vi "SPARC4_AC.vi"() -> ()   [LabVIEW 2018]
uses:
  SPARC4_AC/SPARC4_AC.lvclass
  Channel Manager/Channel Manager.lvclass/Channel Manager.ctl
  Sync Box/Sync Box.lvclass
  Readout delay charact/Readout Delay Charact/Readout Charact.lvclass
  Channel Manager/Channel Manager.lvclass
  RxTx/RxTx.lvclass
  Interface/Interface.lvclass
  State Machine/State Machine.lvclass
  Setup File/Setup File.lvclass
panel:
  out "String":string="#img      1st Time       2nd Time      3th Time      4th Time      5th Time\n------------------------------------------------------------------------\n"
  in  "Camera Setup":T1={"Image Name"="Image", "Image Path"="C:\\Users\\Cliente\\Desktop\\SPARC4_AC\\Imagens\\", "# Images"=0, "Exposure Time"=0.0, "Pre-amp gain"=0, "Readout Rate"=0, "Vertical Shift Speed"=3, "Acquisition Mode"=1, "Read Mode"=4, "EM Mode"=0, "EM Gain"=2, "Shutter Mode"=2, "Shutter TTL"=0, "Time to open shutter"=50, "Time to close shutter"=50, "Vertical Binning"=1, "Horizontal Binning"=1, "Initial Line"=1, "Initial Cloumn"=1, "Final Line"=1024, "Final Column"=1024, "Cooler ON/OFF"=0, "Set temperature"=20, "Number of exp"=0, "Exposições realizadas"=0, "Kinetic Serie Length"=0, "Number of Accumulations"=0, "Kinetic Cycle Time"=0, "Frame Transfer"=FALSE, "Vertical Clock Amplitude"=0, "Trigger"=0} {"Trigger" items=["Internal", "External", "N/A", "N/A", "N/A", "N/A", "External Start"]; "Vertical Clock Amplitude" items=["Normal", "+1", "+2", "+3", "+4"]; "Set temperature" min=0 max=0; "Cooler ON/OFF" items=["Cooler OFF", "Cooler ON"]; "Shutter TTL" items=["TTL Low", "TTl High"]; "Shutter Mode" items=["Fully Auto", "OPEN", "CLOSED"]; "EM Mode" items=["Electron Multiplying", "Conventional"]; "Read Mode" items=["Full Vertical Binning", "Multi-Track", "Random-track", "Single-Track", "Image"]; "Acquisition Mode" items=["N/A", "Single", "Accumulate", "Kinetic", "Fast Kinetic"]; "Vertical Shift Speed" items=["0.6", "1.13", "2.2", "4.33"]; "Readout Rate" items=["1 MHz", "10 MHz", "20 MHz", "30 MHz"]; "Pre-amp gain" items=["Gain 1", "Gain 2"]}
  in  "Setup":T2
  in  "Initial Line 6":u16=1 min=1
  in  "Interface de controle":enum32{"Acquisition", "Setup"}(tab)
  in  "Pausar 5":bool
  in  "Stop Acq 5":bool
  in  "Adquirir 5":bool
  in  "Abort 5":bool
  in  "Pausar 2":bool
  in  "Stop Acq 2":bool
  in  "Adquirir 2":bool
  in  "Abort 2":bool
  in  "Pausar 4":bool
  in  "Stop Acq 4":bool
  in  "Adquirir 4":bool
  in  "Abort 4":bool
  in  "Pausar":bool
  in  "Stop Acq":bool
  in  "Adquirir":bool
  in  "Abort":bool
  in  "Sync Mode":bool
  out "Exposing":bool
  in  "Image Name":string="CH1"
  out "Temperature":i16
  in  "Exposure Time":dbl=1e-05 min=1e-05
  in  "# Ciclos":u32=1 min=1
  out "% Acquired":dbl format="%#.2g"
  in  "Night Directory":string="C:\\Users\\observer\\Desktop\\SPARC4 Acquisition Control\\Imagens"
  in  "COMP":bool
  in  "FLAT":bool
  in  "BIAS":bool
  in  "SCIENCE":bool
  in  "Load Setup":bool
  out "Setup File Path:":string
  in  "Read mode":enum32{"No Selection", "1", "2", "3"}(radio)=enum."1"
  in  "Sync Mode: 2":T3(radio)
  in  "Image Name 4":string="CH1"
  out "Initialization 4":bool
  in  "Exposure Time 6":dbl
  in  "# Images 4":u32=1 min=1
  out "Temperature 4":i16
  out "Exposing 4":bool
  out "% Acquired 4":dbl format="%#.2g"
  out "Exposições realizadas 4":u8(slide) max=1 scale=0.0..1.0
  in  "Image Name 3":string="CH1"
  out "Initialization 3":bool
  in  "Exposure Time 5":dbl
  in  "# Images 3":u32=1 min=1
  out "Temperature 3":i16
  out "Exposing 3":bool
  out "% Acquired 3":dbl format="%#.2g"
  out "Exposições realizadas 3":u8(slide) max=1 scale=0.0..1.0
  in  "Pausar 3":bool
  in  "Stop Acq 3":bool
  in  "Abort 3":bool
  in  "Adquirir 3":bool
  in  "Image Name 2":string="CH2"
  out "Initialization 2":bool
  in  "Exposure Time 3":u32
  in  "# Images 2":u32=1 min=1
  out "Temperature 2":i16
  out "Exposing 2":bool
  out "% Acquired 2":dbl format="%#.2g"
  out "Exposições realizadas 2":u8(slide) max=1 scale=0.0..1.0
  out "Initialization":bool
  out "Exposições realizadas":u8(slide) max=1 scale=0.0..1.0
  in  "Stop Button":bool
  in  "Tab Control 2":T4(tab)
  in  "Cooler ON/OFF":u16(ring) items=["Cooler OFF", "Cooler ON"]
  in  "Set temperature":i8=20 min=-80 max=20
  out "Temperature ºC":dbl(slide)=20.0 min=-120.0 max=20.0 scale=-80.0..20.0
  in  "Exposure Time 2":dbl=1e-05 min=1e-05
  in  "Readout Rate":u8(ring) items=["30 MHz", "20 MHz", "10 MHz", "  1 MHz"]
  in  "Pre-amp gain":u8(ring) items=["Gain 1", "Gain 2"]
  in  "Kinetic Series Length":u8=1 min=1 max=80
  in  "Sub Image":T5(radio)=enum."1024 x 1024"
  in  "Initial Line":u16=1 min=1 max=1024
  in  "Final Line":u16=1024 min=1 max=1024
  in  "Final Column":u16=1024 min=1 max=1024
  in  "Initial Cloumn":u16=1 min=1 max=1024
  in  "Binning 5":u8=1 min=1 max=2
  in  "EM Gain":u16=2 min=2 max=300
  in  "EM Mode":u8(ring) items=["Electron Multiplying", "Conventional"]
  in  "Save CH1":bool
  in  "Save CH2":bool
  in  "Cooler ON/OFF 2":u16(ring) items=["Cooler OFF", "Cooler ON"]
  in  "Set temperature 2":i8=20 min=-120 max=20
  out "Temperature ºC 2":dbl(slide)=20.0 min=-120.0 max=20.0 scale=-80.0..20.0
  in  "Exposure Time 4":u32
  in  "Readout Rate 2":u8(ring) items=["1 MHz", "10 MHz", "20 MHz", "30 MHz"]
  in  "Pre-amp gain 2":u8(ring) items=["Gain 1", "Gain 2"]
  in  "EM Gain 2":u16=2
  in  "EM Mode 2":u8(ring) items=["Electron Multiplying", "Conventional"]
  in  "Sub Image 2":T5(radio)=enum."1024 x 1024"
  in  "Final Line 2":u16=1024
  in  "Final Column 2":u16=1024
  in  "Initial Cloumn 2":u16=1
  in  "Initial Line 2":u16=1
  in  "Binning 6":u16=1
  in  "Save CH3":bool
  in  "Cooler ON/OFF 3":u16(ring) items=["Cooler OFF", "Cooler ON"]
  in  "Set temperature 3":i8=20 min=-120 max=20
  out "Temperature ºC 3":dbl(slide)=20.0 min=-120.0 max=20.0 scale=-80.0..20.0
  in  "Exposure Time 7":dbl
  in  "Readout Rate 3":u8(ring) items=["1 MHz", "10 MHz", "20 MHz", "30 MHz"]
  in  "Pre-amp gain 3":u8(ring) items=["Gain 1", "Gain 2"]
  in  "EM Gain 3":u16=2
  in  "EM Mode 3":u8(ring) items=["Electron Multiplying", "Conventional"]
  in  "Sub Image 3":T5(radio)=enum."1024 x 1024"
  in  "Final Line 3":u16=1024
  in  "Final Column 3":u16=1024
  in  "Initial Cloumn 3":u16=1
  in  "Initial Line 3":u16=1
  in  "Binning 7":u16=1
  in  "Save CH4":bool
  in  "Cooler ON/OFF 4":u16(ring) items=["Cooler OFF", "Cooler ON"]
  in  "Set temperature 4":i8=20 min=-120 max=20
  out "Temperature ºC 4":dbl(slide)=20.0 min=-120.0 max=20.0 scale=-80.0..20.0
  in  "Exposure Time 8":dbl
  in  "Readout Rate 4":u8(ring) items=["1 MHz", "10 MHz", "20 MHz", "30 MHz"]
  in  "Pre-amp gain 4":u8(ring) items=["Gain 1", "Gain 2"]
  in  "EM Gain 4":u16=2
  in  "EM Mode 4":u8(ring) items=["Electron Multiplying", "Conventional"]
  in  "Sub Image 4":T5(radio)=enum."1024 x 1024"
  in  "Final Line 4":u16=1024
  in  "Final Column 4":u16=1024
  in  "Initial Cloumn 4":u16=1
  in  "Initial Line 4":u16=1
  in  "Binning 8":u16=1
  in  "SPARC4_AC.lvclass":refnum<class "SPARC4_AC.lvclass">
  # "#img      1st Time       2nd Time      3th Time      4th Time      5th Time"
  # "Sparc4:\n Acquisition Controller"
  # "Channel 1"
  # "Channel 2"
  # "Channel 3"
  # "Channel 4"
  # "Timings"
  # "Temperature"
  # "HSS & Preamp"
  # "EM Mode"
  # "Sub Image & Binning"
  # "Timings"
  # "Temperature"
  # "EM Mode"
  # "HSS & Preamp"
  # "Sub Image & Binning"
  # "Timings"
  # "Temperature"
  # "HSS & Preamp"
  # "EM Mode"
  # "Sub Image & Binning"
  # "Temperature"
  # "Timings"
  # "EM Mode"
  # "Horizontal pixel shift"
  # "Sub Image & Binning"
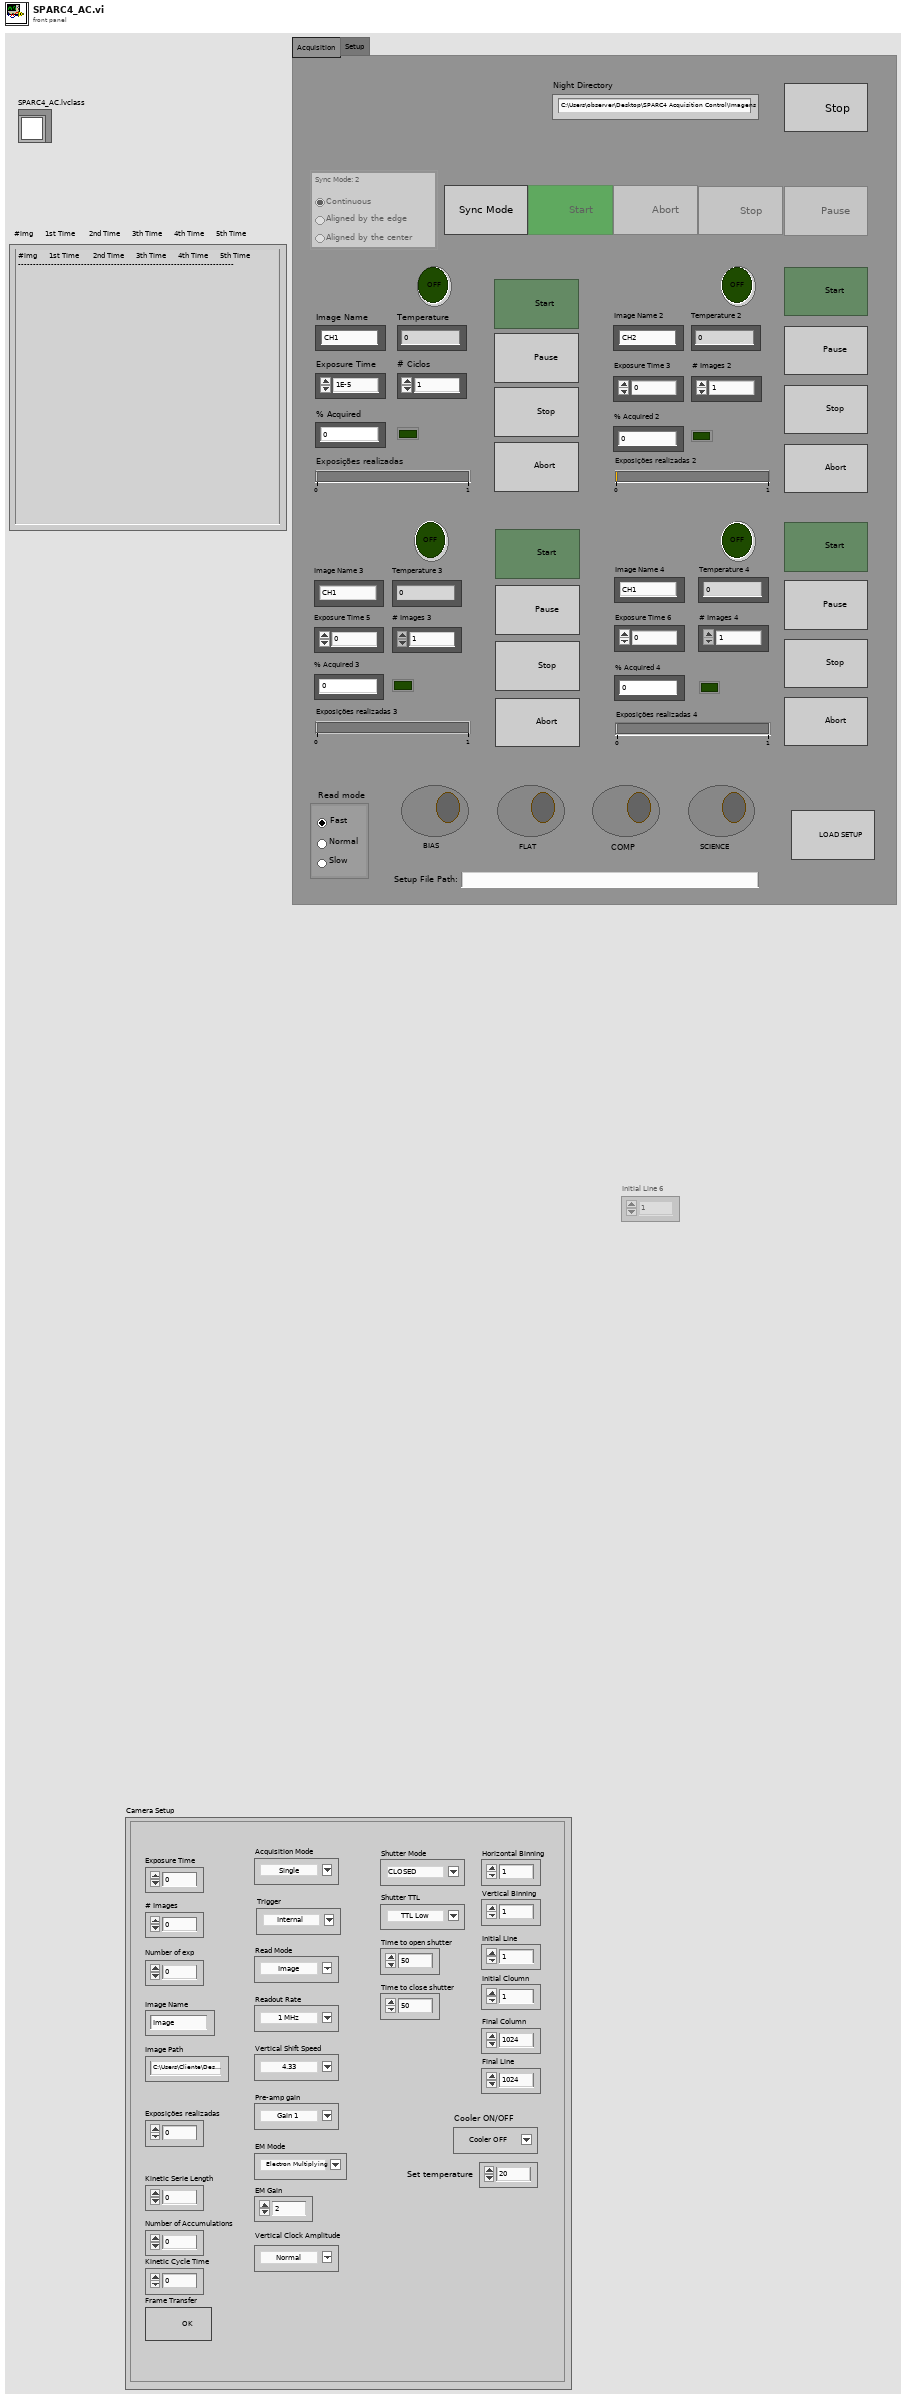
[diagram p1: front panel]
types:
  T1 = cluster{"Image Name":string, "Image Path":string, "# Images":u32, "Exposure Time":dbl, "Pre-amp gain":u8, "Readout Rate":u8, "Vertical Shift Speed":u8, "Acquisition Mode":u8, "Read Mode":u8, "EM Mode":u8, "EM Gain":u16, "Shutter Mode":u8, "Shutter TTL":u8, "Time to open shutter":u16, "Time to close shutter":u16, "Vertical Binning":u16, "Horizontal Binning":u16, "Initial Line":u16, "Initial Cloumn":u16, "Final Line":u16, "Final Column":u16, "Cooler ON/OFF":u16, "Set temperature":i8, "Number of exp":u32, "Exposições realizadas":u16, "Kinetic Serie Length":u32, "Number of Accumulations":u32, "Kinetic Cycle Time":u32, "Frame Transfer":bool, "Vertical Clock Amplitude":u8, "Trigger":u8}
  T2 = cluster{"Read Mode":string, "Acquisition Mode":string, "Trigger":string, "Exposure Time":string, "VShift Speed":string, "Readout rate":string, "Pre amp":string, "Shutter Mode":string, "Shutter TTL":string, "Time to open shutter":string, "Time to close shutter":string, "Cooler":string, "Temperature":string, "Initial Line":string, "Initial Column":string, "Final Line":string, "Final Column":string, "Horizontal binning":string, "Vertical binning":string, "Sub image":string, "CHANNEL":string, "EM Mode":string, "EM Gain":string}
  T3 = enum32{"Radio Selection 1", "Radio Selection 2", "Radio Selection 3", "Radio Selection 4"}
  T4 = enum32{"Channel 1", "Channel 2", "Channel 3", "Channel 4"}
  T5 = enum32{"256 x 256", "512 x 512", "1024 x 1024", "Custom"}
  T6 = cluster{"% Acquired":dbl, "Acquiring":bool, "Current Temperature":dbl, "Temperatue Status":string, "Min Temp":dbl, "Max Temp":dbl, "Exposições realizadas":u32, "Final Column":u16, "Final Line":u16}
  T7 = enum8{"Enabled", "Disabled", "Disabled and Grayed Out"}
  T8 = enum32{"256 x 256", "512 x 512", "1024 x 1024", "Custom", "128 x 128", "64 x 64"}
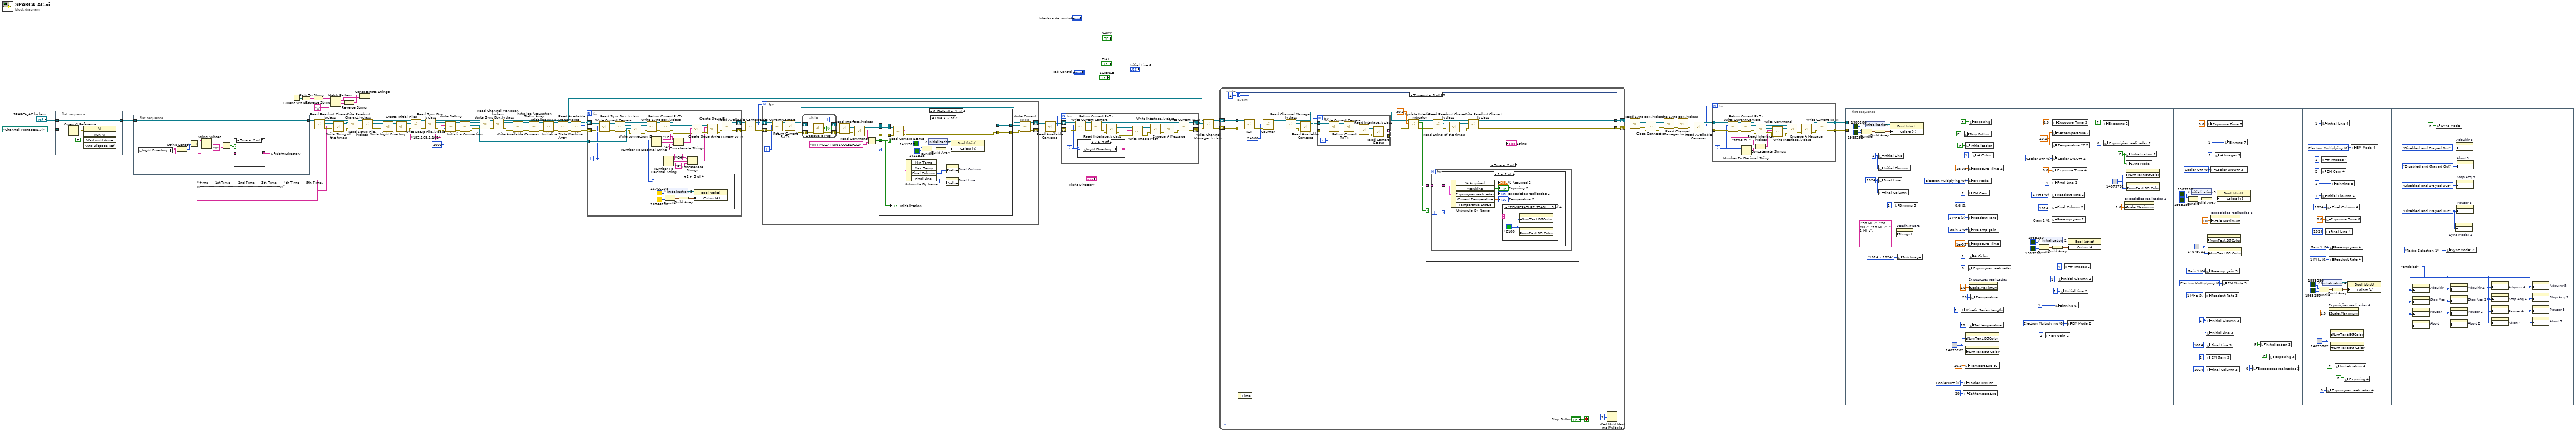
[diagram p0: block diagram]
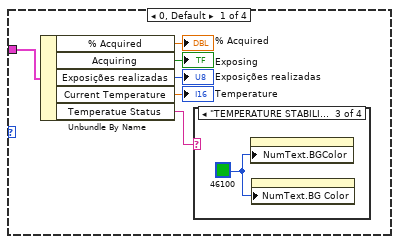
[diagram p3: hidden frame]
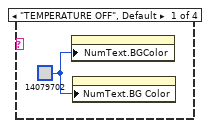
[diagram p4: hidden frame]
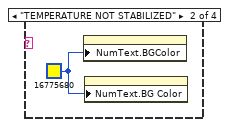
[diagram p5: hidden frame]
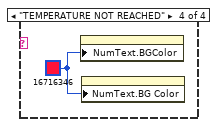
[diagram p6: hidden frame]
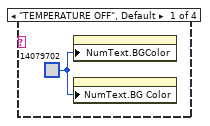
[diagram p7: hidden frame]
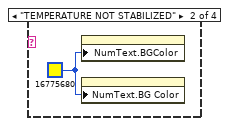
[diagram p8: hidden frame]
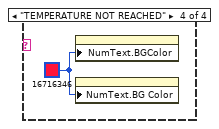
[diagram p9: hidden frame]
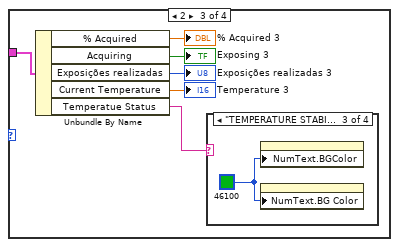
[diagram p10: hidden frame]
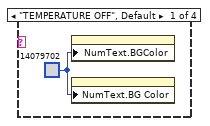
[diagram p11: hidden frame]
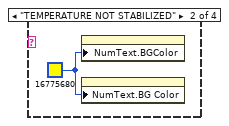
[diagram p12: hidden frame]
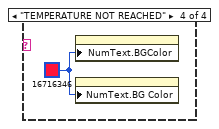
[diagram p13: hidden frame]
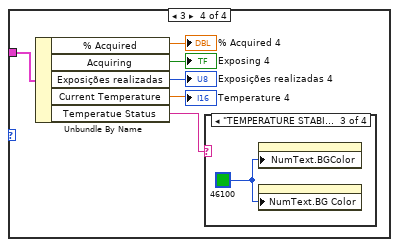
[diagram p14: hidden frame]
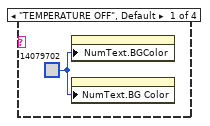
[diagram p15: hidden frame]
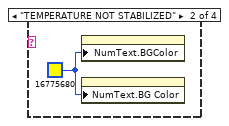
[diagram p16: hidden frame]
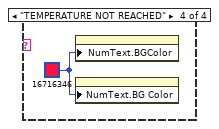
[diagram p17: hidden frame]
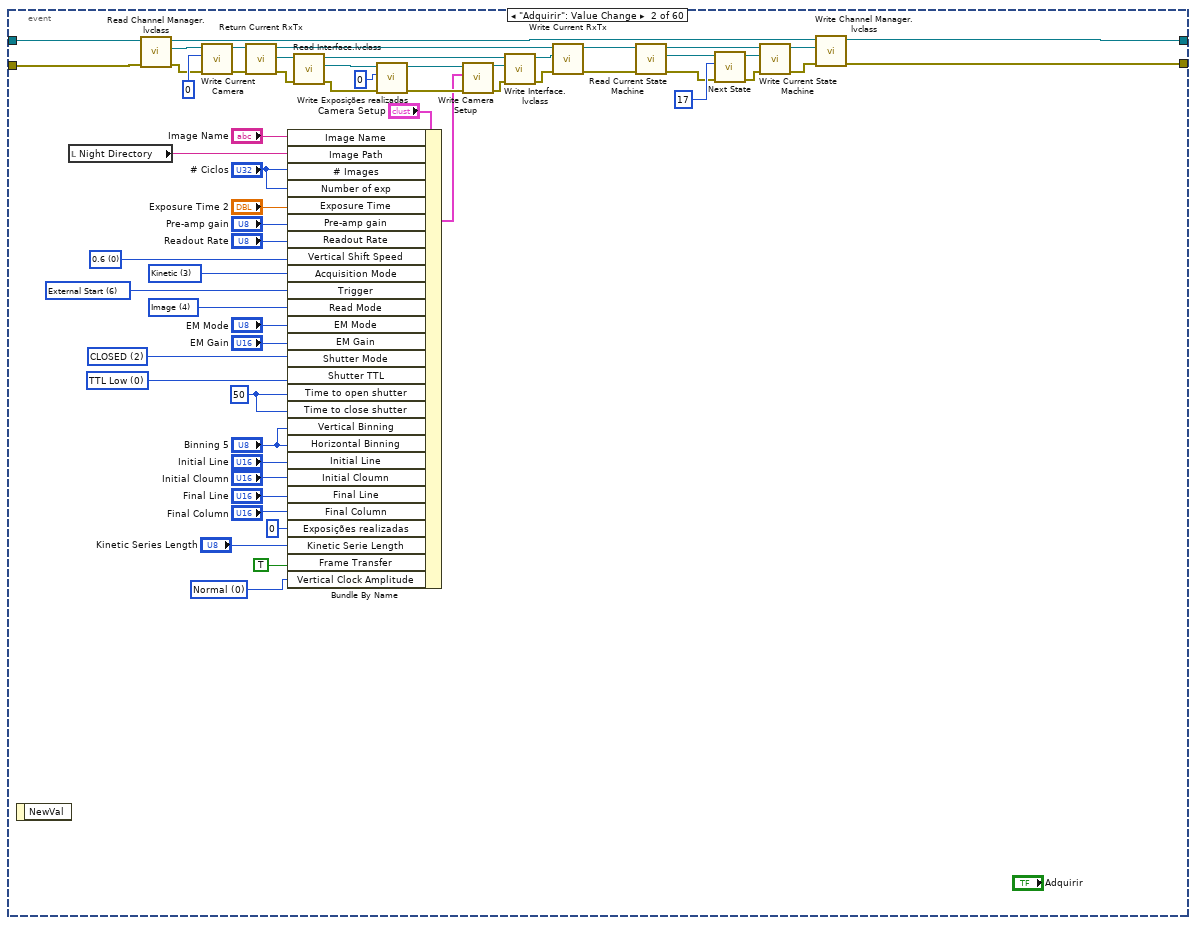
[diagram p18: hidden frame]
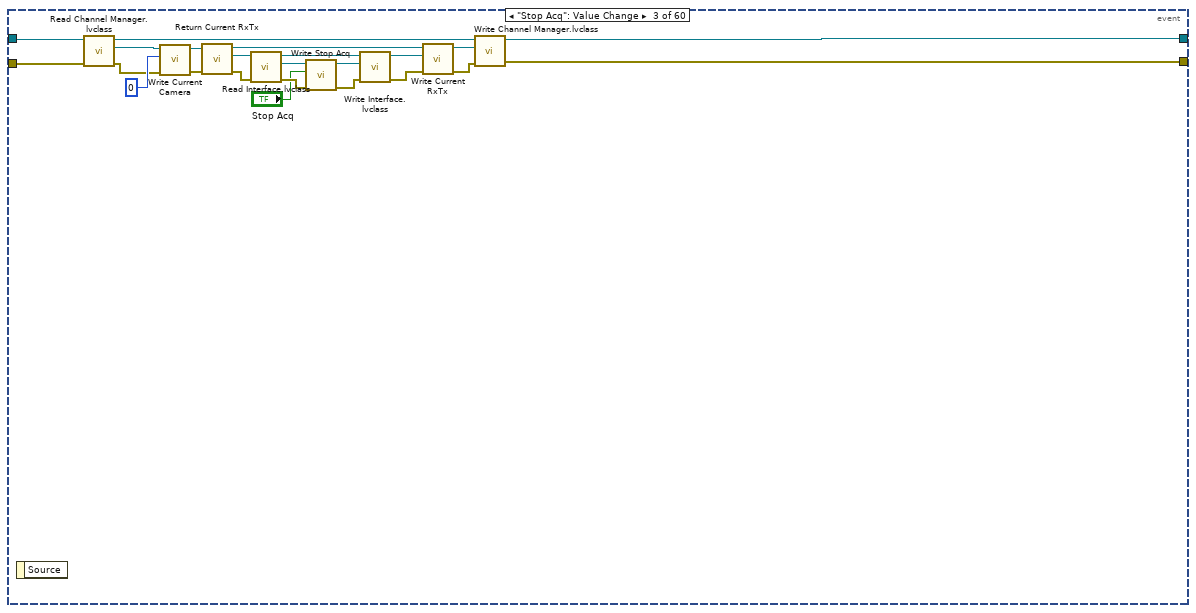
[diagram p19: hidden frame]
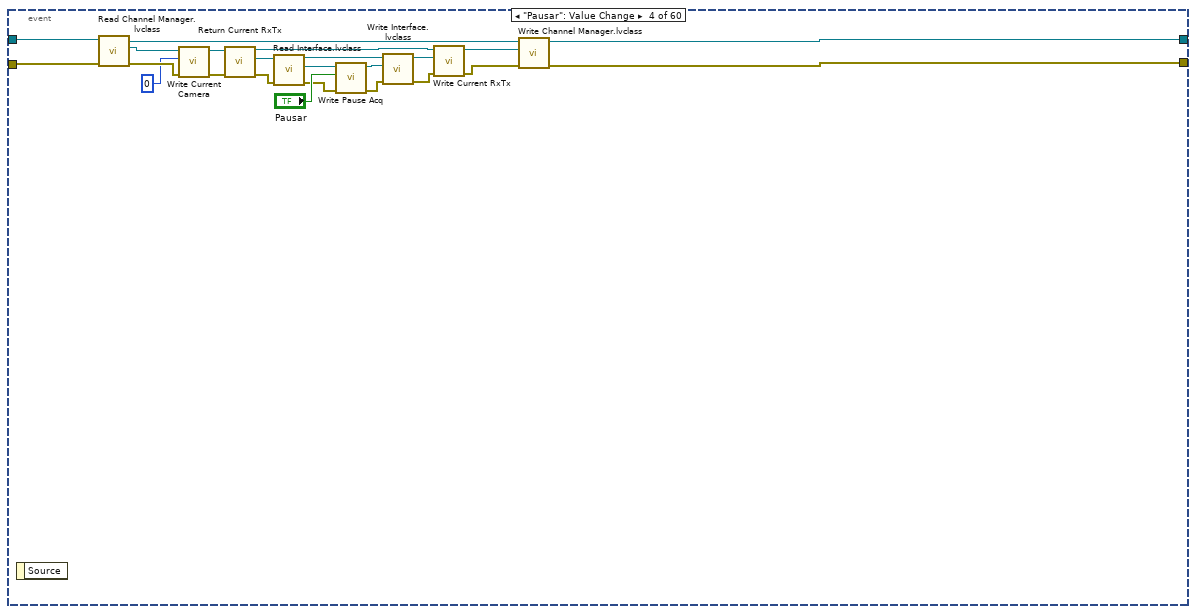
[diagram p20: hidden frame]
diagram:
  n1 = flat-sequence {
    tunnel: "SPARC4_AC.lvclass" -> [w87]
    tunnel: [w87] -> w19
    tunnel: path "Channel_Manager2.vi" ("vi path") -> [w85]
    frame #0 {
      n2 = Open VI Reference(vi path=w85) -> (vi reference=w89:refnum<vi>, error out=w88:errorcluster)  [unwired: 5 in]
      n3 = invoke class="VI" method="Run VI"(reference=w89, error in=w88, "Wait until done"=FALSE ("Wait Until Done")) -> ()  [unwired: 2 in, 5 out]
    }
  }
  n4 = flat-sequence {
    tunnel: w19 -> [w90]
    tunnel: [w90] -> w9
    frame #0 {
      n5 = local read "Night Directory"() -> (w96:string)
      n6 = String Length(string=w96) -> (length=w91:i32)
      n7 = Decrement(x=w91) -> (x-1=w92:i32)
      n8 = String Subset(string=w96, offset (0)=w92) -> (substring=w93:string)  [unwired: 1 in]
      n9 = Equal?(x=w93, y="\\") -> (x = y?=w94:bool)
      n10 = case shown="True" w94 {
        tunnel: [w100 w101] -> w97
        tunnel: w96 -> [w98 w101]
        frame False {
          n11 = Concatenate Strings(w98, "\\") -> (w100:string)
        }
        frame True {
        }
      }
      n12 = local write "Night Directory"(w97) -> ()
    }
  }
  n13 = Current VI's Path() -> (path=w17:path)
  n14 = Path To String(path=w17) -> (string=w16:string)
  n15 = Reverse String(1:w16) -> (0:w15:string)
  n16 = call-dynamic "Read Readout Charact.lvclass.vi"("SPARC4_AC in"=w9) -> ("error out"=w2:errorcluster, "Readout Charact.lvclass"=w4:refnum<class "Readout Charact.lvclass">, "SPARC4_AC out"=w5:refnum<class "SPARC4_AC.lvclass">)  [unwired: 8 in]
  n17 = Match Pattern(string=w15, regular expression="\\") -> (match substring=w11:string, after substring=w13:string)  [unwired: 1 in, 2 out]
  n18 = call-dynamic "Write String of the times.vi"("error in (no error)"=w2, "String of the times"="#img      1st Time       2nd Time      3th Time      4th Time      5th Time\n------------------------------------------------------------------------\n" ("String 2"), "Readout Charact in"=w4) -> ("error out"=w3:errorcluster, "Readout Charact out"=w6:refnum<class "Readout Charact.lvclass">)  [unwired: 7 in]
  n19 = Reverse String(1:w13) -> (0:w12:string)
  n20 = call-dynamic "Write Readout Charact.lvclass.vi"("error in (no error)"=w3, "Readout Charact.lvclass"=w6, "SPARC4_AC in"=w5) -> ("error out"=w7:errorcluster, "SPARC4_AC out"=w8:refnum<class "SPARC4_AC.lvclass">)  [unwired: 7 in]
  n21 = Concatenate Strings(w12, w11) -> (w10:string)
  n22 = call-dynamic "Read Setup File.lvclass.vi"("error in (no error)"=w7, "SPARC4_AC in"=w8) -> ("error out"=w57:errorcluster, "Setup File.lvclass"=w58:refnum<class "Setup File.lvclass">, "SPARC4_AC out"=w61:refnum<class "SPARC4_AC.lvclass">)  [unwired: 7 in]
  n23 = call "Write Night Directory.vi"("error in (no error)"=w57, "Directory"=w10, "Setup File in"=w58) -> ("error out"=w60:errorcluster, "Setup File out"=w59:refnum<class "Setup File.lvclass">)  [unwired: 7 in]
  n24 = call "Create Initial Files.vi"("error in (no error)"=w60, "Setup File in"=w59) -> ("error out"=w62:errorcluster, "Setup File out"=w63:refnum<class "Setup File.lvclass">)  [unwired: 8 in]
  n25 = call-dynamic "Write Setup File.lvclass.vi"("error in (no error)"=w62, "Setup File.lvclass"=w63, "SPARC4_AC in"=w61) -> ("error out"=w65:errorcluster, "SPARC4_AC out"=w64:refnum<class "SPARC4_AC.lvclass">)  [unwired: 7 in]
  n26 = call-dynamic "Read Sync Box.lvclass.vi"("error in (no error)"=w65, "SPARC4_AC in"=w64) -> ("error out"=w78:errorcluster, "Sync Box.lvclass"=w84:refnum<class "Sync Box.lvclass">, "SPARC4_AC out"=w81:refnum<class "SPARC4_AC.lvclass">)  [unwired: 7 in]
  n27 = call "Write Setting.vi"("error in (no error)"=w78, "Remote Port"=u32 2000 ("Remote Port:"), "Address"="192.168.1.101" ("Address:"), "Sync Box in"=w84) -> ("error out"=w83:errorcluster, "Sync Box out"=w82:refnum<class "Sync Box.lvclass">)  [unwired: 6 in]
  n28 = call "Initialize Connection.vi"("error in (no error)"=w83, "Sync Box in"=w82) -> ("error out"=w66:errorcluster, "connection ID"=w51:refnum<k5>, "Sync Box out"=w67:refnum<class "Sync Box.lvclass">)  [unwired: 7 in]
  n29 = call-dynamic "Write Sync Box.lvclass.vi"("error in (no error)"=w66, "Sync Box.lvclass"=w67, "SPARC4_AC in"=w81) -> ("error out"=w35:errorcluster, "SPARC4_AC out"=w36:refnum<class "SPARC4_AC.lvclass">)  [unwired: 7 in]
  n30 = call-dynamic "Read Channel Manager.lvclass.vi"("error in (no error)"=w35, "SPARC4_AC in"=w36) -> ("error out"=w20:errorcluster, "Channel Manager.lvclass"=w21:refnum<class "Channel Manager.lvclass">, "SPARC4_AC out"=w69:refnum<class "SPARC4_AC.lvclass">)  [unwired: 7 in]
  n31 = call-dynamic "Write Available Cameras.vi"("error in (no error)"=w20, "Channel Manager in"=w21) -> ("error out"=w23:errorcluster, "Channel Manager out"=w22:refnum<class "Channel Manager.lvclass">)  [unwired: 8 in]
  n32 = call "Initialize Acquisition Status Array.vi"("error in (no error)"=w23, "Channel Manager in"=w22) -> ("error out"=w25:errorcluster, "Channel Manager out"=w24:refnum<class "Channel Manager.lvclass">)  [unwired: 8 in]
  n33 = call "Initialize RxTx Array.vi"("error in (no error)"=w25, "Channel Manager in"=w24) -> ("error out"=w32:errorcluster, "Channel Manager out"=w31:refnum<class "Channel Manager.lvclass">)  [unwired: 8 in]
  n34 = call "Initialize State Machine Array.vi"("error in (no error)"=w32, "Channel Manager in"=w31) -> ("error out"=w34:errorcluster, "Channel Manager out"=w33:refnum<class "Channel Manager.lvclass">)  [unwired: 8 in]
  n35 = call-dynamic "Read Available Cameras.vi"("error in (no error)"=w34, "Channel Manager in"=w33) -> ("error out"=w48:errorcluster, "Available Cameras"=w50:u8, "Channel Manager out"=w49:refnum<class "Channel Manager.lvclass">)  [unwired: 7 in]
  n36 = for {
    N: w50 -> [_]
    tunnel: w51 -> [w114]
    shift-right: [w102] -> w46
    shift-left: w49 -> [w106]
    shift-right: [w103] -> w47
    shift-left: w48 -> [w105]
    i -> [w104]
    n37 = call-dynamic "Write Current Camera.vi"("error in (no error)"=w105, "Current Camera"=w104, "Channel Manager in"=w106) -> ("error out"=w108:errorcluster, "Channel Manager out"=w107:refnum<class "Channel Manager.lvclass">)  [unwired: 7 in]
    n38 = call "Read Sync Box.lvclass.vi"("error in (no error)"=w108, "Channel Manager in"=w107) -> ("error out"=w110:errorcluster, "Sync Box.lvclass"=w113:refnum<class "Sync Box.lvclass">, "Channel Manager out"=w109:refnum<class "Channel Manager.lvclass">)  [unwired: 7 in]
    n39 = call-dynamic "Write connection ID.vi"("error in (no error)"=w110, "connection ID"=w114, "Sync Box in"=w113) -> ("error out"=w111:errorcluster, "Sync Box out"=w112:refnum<class "Sync Box.lvclass">)  [unwired: 7 in]
    n40 = call "Write Sync Box.lvclass.vi"("error in (no error)"=w111, "Sync Box.lvclass"=w112, "Channel Manager in"=w109) -> ("error out"=w116:errorcluster, "Channel Manager out"=w115:refnum<class "Channel Manager.lvclass">)  [unwired: 7 in]
    n41 = Number To Decimal String(number=w104) -> (decimal integer string=w128:string)  [unwired: 1 in]
    n42 = case shown="2" w104 {
      frame 0, Default {
        n43 = Bundle(u32 16766208, u32 16766208) -> (w136:cluster{u32, u32})  [unwired: 1 in]
        n44 = control-ref of="Initialization"() -> (w134:refnum<vi>)
        n45 = Build Array(w136) -> (w135:cluster{u32, u32}[])
        n46 = property on="Property Node" class="Bool (strict)"(reference=w134, "Colors [4]"=w135) -> ()  [unwired: 1 in, 2 out]
      }
      frame 1 {
        n47 = Bundle(u32 16766208, u32 16766208) -> (w139:cluster{u32, u32})  [unwired: 1 in]
        n48 = control-ref of="Initialization 2"() -> (w141:refnum<vi>)
        n49 = Build Array(w139) -> (w140:cluster{u32, u32}[])
        n50 = property on="Property Node" class="Bool (strict)"(reference=w141, "Colors [4]"=w140) -> ()  [unwired: 1 in, 2 out]
      }
      frame 2 {
        n51 = Bundle(u32 16766208, u32 16766208) -> (w146:cluster{u32, u32})  [unwired: 1 in]
        n52 = control-ref of="Initialization 3"() -> (w144:refnum<vi>)
        n53 = Build Array(w146) -> (w145:cluster{u32, u32}[])
        n54 = property on="Property Node" class="Bool (strict)"(reference=w144, "Colors [4]"=w145) -> ()  [unwired: 1 in, 2 out]
      }
      frame 3 {
        n55 = Bundle(u32 16766208, u32 16766208) -> (w149:cluster{u32, u32})  [unwired: 1 in]
        n56 = control-ref of="Initialization 4"() -> (w151:refnum<vi>)
        n57 = Build Array(w149) -> (w150:cluster{u32, u32}[])
        n58 = property on="Property Node" class="Bool (strict)"(reference=w151, "Colors [4]"=w150) -> ()  [unwired: 1 in, 2 out]
      }
    }
    n59 = call "Return Current RxTx.vi"("error in (no error)"=w116, "Channel Manager in"=w115) -> ("error out"=w120:errorcluster, "RxTx"=w121:refnum<class "RxTx.lvclass">, "Channel Manager out"=w119:refnum<class "Channel Manager.lvclass">)  [unwired: 7 in]
    n60 = Number To Decimal String(number=w104) -> (decimal integer string=w125:string)  [unwired: 1 in]
    n61 = Concatenate Strings("CH", w128, "A") -> (w126:string)
    n62 = Concatenate Strings("CH", w125, "B") -> (w122:string)
    n63 = call "Create Qeue A.vi"("error in (no error)"=w120, "Qeue A"=w126, "RxTx in"=w121) -> ("error out"=w131:errorcluster, "RxTx out"=w130:refnum<class "RxTx.lvclass">)  [unwired: 7 in]
    n64 = call "Create Qeue B.vi"("error in (no error)"=w131, "Qeue B"=w122, "RxTx in"=w130) -> ("error out"=w117:errorcluster, "RxTx out"=w118:refnum<class "RxTx.lvclass">)  [unwired: 7 in]
    n65 = call "Write Current RxTx.vi"("error in (no error)"=w117, "RxTx"=w118, "Channel Manager in"=w119) -> ("error out"=w103:errorcluster, "Channel Manager out"=w102:refnum<class "Channel Manager.lvclass">)  [unwired: 7 in]
  }
  n66 = call-dynamic "Read Available Cameras.vi"("error in (no error)"=w47, "Channel Manager in"=w46) -> ("error out"=w43:errorcluster, "Available Cameras"=w45:u8, "Channel Manager out"=w44:refnum<class "Channel Manager.lvclass">)  [unwired: 7 in]
  n67 = for {
    N: w45 -> [_]
    shift-right: [w158] -> w41
    shift-left: w43 -> [w153]
    shift-right: [w157] -> w40
    shift-left: w44 -> [w154]
    i -> [w152]
    n68 = call-dynamic "Write Current Camera.vi"("error in (no error)"=w153, "Current Camera"=w152, "Channel Manager in"=w154) -> ("error out"=w156:errorcluster, "Channel Manager out"=w155:refnum<class "Channel Manager.lvclass">)  [unwired: 7 in]
    n69 = call "Return Current RxTx.vi"("error in (no error)"=w156, "Channel Manager in"=w155) -> ("error out"=w173:errorcluster, "RxTx"=w172:refnum<class "RxTx.lvclass">, "Channel Manager out"=w159:refnum<class "Channel Manager.lvclass">)  [unwired: 7 in]
    n70 = while {
      shift-right: [w176] -> w167
      shift-left: w173 -> [w178]
      shift-right: [w175] -> w166
      shift-left: w172 -> [w177]
      stop <- w174 continue-if-true
      n71 = call "Deqeue B Msg.vi"("error in (no error)"=w178, "RxTx in"=w177) -> ("error out"=w176:errorcluster, "timeout?"=w174:bool, "RxTx out"=w175:refnum<class "RxTx.lvclass">)  [unwired: 7 in]
    }
    n72 = call-dynamic "Read Interface.lvclass.vi"("error in (no error)"=w167, "RxTx in"=w166) -> ("error out"=w169:errorcluster, "Interface.lvclass"=w168:refnum<class "Interface.lvclass">, "RxTx out"=w162:refnum<class "RxTx.lvclass">)  [unwired: 7 in]
    n73 = call "Read Command.vi"("error in (no error)"=w169, "Interface in"=w168) -> ("error out"=w163:errorcluster, "Command"=w171:string, "Interface out"=w164:refnum<class "Interface.lvclass">)  [unwired: 7 in]
    n74 = Equal?(x=w171, y="INITIALIZATION SUCCESFULL") -> (x = y?=w165:bool)
    n75 = case shown="0, Default" w152 {
      tunnel: w165 -> [w184 w209 w234 w261]
      tunnel: w164 -> [w183 w212 w238 w265]
      tunnel: w163 -> [w182 w211 w237 w264]
      tunnel: w162 -> [w181 w210 w239 w266]
      tunnel: [w180 w208 w235 w262] -> w161
      tunnel: [w179 w207 w236 w263] -> w160
      frame 0, Default {
        n76 = case shown="True" w184 {
          tunnel: w183 -> [w193 w205]
          tunnel: w182 -> [w192 w206]
          tunnel: w181 -> [w194 w203]
          tunnel: [w191 w203] -> w180
          tunnel: [w190 w202] -> w179
          frame False {
            n77 = call-dynamic "Write Interface.lvclass.vi"("error in (no error)"=w192, "Interface.lvclass"=w193, "RxTx in"=w194) -> ("error out"=w190:errorcluster, "RxTx out"=w191:refnum<class "RxTx.lvclass">)  [unwired: 7 in]
            n78 = Bundle(u32 1985280, u32 1985280) -> (w187:cluster{u32, u32})  [unwired: 1 in]
            n79 = control-ref of="Initialization"() -> (w189:refnum<vi>)
            n80 = Build Array(w187) -> (w188:cluster{u32, u32}[])
            n81 = property on="Property Node" class="Bool (strict)"(reference=w189, "Colors [4]"=w188) -> ()  [unwired: 1 in, 2 out]
          }
          frame True {
            n82 = call "Read Camera Status.vi"("error in (no error)"=w206, "Interface in"=w205) -> ("error out"=w202:errorcluster, "Camera Status"=w204:T6)  [unwired: 7 in, 1 out]
            n83 = Unbundle By Name(w204) -> ("Final Column"=w197:u16, "Final Line"=w196:u16)  [unwired: 2 out]
            n84 = Bundle(u32 1411328, u32 1411328) -> (w201:cluster{u32, u32})  [unwired: 1 in]
            n85 = control-ref of="Initialization"() -> (w199:refnum<vi>)
            n86 = Build Array(w201) -> (w200:cluster{u32, u32}[])
            n87 = property on="Final Line" class="DigNum (strict)"("Value"=w196) -> ()  [unwired: 2 in, 2 out]
            n88 = property on="Final Column" class="DigNum (strict)"("Value"=w197) -> ()  [unwired: 2 in, 2 out]
            n89 = property on="Property Node" class="Bool (strict)"(reference=w199, "Colors [4]"=w200) -> ()  [unwired: 1 in, 2 out]
          }
        }
        "Initialization" <- w184
      }
      frame 1 {
        n90 = case shown="True" w209 {
          tunnel: w212 -> [w221 w232]
          tunnel: w211 -> [w220 w233]
          tunnel: w210 -> [w222 w230]
          tunnel: [w219 w230] -> w208
          tunnel: [w218 w229] -> w207
          frame False {
            n91 = call-dynamic "Write Interface.lvclass.vi"("error in (no error)"=w220, "Interface.lvclass"=w221, "RxTx in"=w222) -> ("error out"=w218:errorcluster, "RxTx out"=w219:refnum<class "RxTx.lvclass">)  [unwired: 7 in]
            n92 = Bundle(u32 1985280, u32 1985280) -> (w216:cluster{u32, u32})  [unwired: 1 in]
            n93 = control-ref of="Initialization 2"() -> (w213:refnum<vi>)
            n94 = Build Array(w216) -> (w217:cluster{u32, u32}[])
            n95 = property on="Property Node" class="Bool (strict)"(reference=w213, "Colors [4]"=w217) -> ()  [unwired: 1 in, 2 out]
          }
          frame True {
            w223 = u32 1411328
            n96 = call "Read Camera Status.vi"("error in (no error)"=w233, "Interface in"=w232) -> ("error out"=w229:errorcluster, "Camera Status"=w231:T6)  [unwired: 7 in, 1 out]
            n97 = Unbundle By Name(w231) -> ("Final Line"=w225:u16, "Final Column"=w224:u16)  [unwired: 2 out]
            n98 = Bundle(w223, w223) -> (w228:cluster{u32, u32})  [unwired: 1 in]
            n99 = control-ref of="Initialization 2"() -> (w226:refnum<vi>)
            n100 = Build Array(w228) -> (w227:cluster{u32, u32}[])
            n101 = property on="Final Line 2" class="DigNum (strict)"("Value"=w225) -> ()  [unwired: 2 in, 2 out]
            n102 = property on="Final Column 2" class="DigNum (strict)"("Value"=w224) -> ()  [unwired: 2 in, 2 out]
            n103 = property on="Property Node" class="Bool (strict)"(reference=w226, "Colors [4]"=w227) -> ()  [unwired: 1 in, 2 out]
          }
        }
        "Initialization 2" <- w209
      }
      frame 2 {
        n104 = case shown="True" w234 {
          tunnel: w238 -> [w248 w259]
          tunnel: w237 -> [w247 w260]
          tunnel: w239 -> [w249 w257]
          tunnel: [w246 w257] -> w235
          tunnel: [w245 w256] -> w236
          frame False {
            n105 = call-dynamic "Write Interface.lvclass.vi"("error in (no error)"=w247, "Interface.lvclass"=w248, "RxTx in"=w249) -> ("error out"=w245:errorcluster, "RxTx out"=w246:refnum<class "RxTx.lvclass">)  [unwired: 7 in]
            n106 = Bundle(u32 1985280, u32 1985280) -> (w243:cluster{u32, u32})  [unwired: 1 in]
            n107 = control-ref of="Initialization 3"() -> (w240:refnum<vi>)
            n108 = Build Array(w243) -> (w244:cluster{u32, u32}[])
            n109 = property on="Property Node" class="Bool (strict)"(reference=w240, "Colors [4]"=w244) -> ()  [unwired: 1 in, 2 out]
          }
          frame True {
            w250 = u32 1411328
            n110 = call "Read Camera Status.vi"("error in (no error)"=w260, "Interface in"=w259) -> ("error out"=w256:errorcluster, "Camera Status"=w258:T6)  [unwired: 7 in, 1 out]
            n111 = Bundle(w250, w250) -> (w255:cluster{u32, u32})  [unwired: 1 in]
            n112 = Unbundle By Name(w258) -> ("Final Column"=w252:u16, "Final Line"=w251:u16)  [unwired: 2 out]
            n113 = control-ref of="Initialization 3"() -> (w253:refnum<vi>)
            n114 = Build Array(w255) -> (w254:cluster{u32, u32}[])
            n115 = property on="Property Node" class="Bool (strict)"(reference=w253, "Colors [4]"=w254) -> ()  [unwired: 1 in, 2 out]
            n116 = property on="Final Column 3" class="DigNum (strict)"("Value"=w252) -> ()  [unwired: 2 in, 2 out]
            n117 = property on="Final Line 3" class="DigNum (strict)"("Value"=w251) -> ()  [unwired: 2 in, 2 out]
          }
        }
        "Initialization 3" <- w234
      }
      frame 3 {
        n118 = case shown="True" w261 {
          tunnel: w265 -> [w275 w286]
          tunnel: w264 -> [w274 w287]
          tunnel: w266 -> [w276 w284]
          tunnel: [w273 w284] -> w262
          tunnel: [w272 w283] -> w263
          frame False {
            n119 = call-dynamic "Write Interface.lvclass.vi"("error in (no error)"=w274, "Interface.lvclass"=w275, "RxTx in"=w276) -> ("error out"=w272:errorcluster, "RxTx out"=w273:refnum<class "RxTx.lvclass">)  [unwired: 7 in]
            n120 = Bundle(u32 1985280, u32 1985280) -> (w270:cluster{u32, u32})  [unwired: 1 in]
            n121 = control-ref of="Initialization 4"() -> (w267:refnum<vi>)
            n122 = Build Array(w270) -> (w271:cluster{u32, u32}[])
            n123 = property on="Property Node" class="Bool (strict)"(reference=w267, "Colors [4]"=w271) -> ()  [unwired: 1 in, 2 out]
          }
          frame True {
            w277 = u32 1411328
            n124 = call "Read Camera Status.vi"("error in (no error)"=w287, "Interface in"=w286) -> ("error out"=w283:errorcluster, "Camera Status"=w285:T6)  [unwired: 7 in, 1 out]
            n125 = Unbundle By Name(w285) -> ("Final Line"=w279:u16, "Final Column"=w278:u16)  [unwired: 2 out]
            n126 = Bundle(w277, w277) -> (w282:cluster{u32, u32})  [unwired: 1 in]
            n127 = control-ref of="Initialization 4"() -> (w280:refnum<vi>)
            n128 = Build Array(w282) -> (w281:cluster{u32, u32}[])
            n129 = property on="Property Node" class="Bool (strict)"(reference=w280, "Colors [4]"=w281) -> ()  [unwired: 1 in, 2 out]
            n130 = property on="Final Column 4" class="DigNum (strict)"("Value"=w278) -> ()  [unwired: 2 in, 2 out]
            n131 = property on="Final Line 4" class="DigNum (strict)"("Value"=w279) -> ()  [unwired: 2 in, 2 out]
          }
        }
        "Initialization 4" <- w261
      }
    }
    n132 = call "Write Current RxTx.vi"("error in (no error)"=w160, "RxTx"=w161, "Channel Manager in"=w159) -> ("error out"=w158:errorcluster, "Channel Manager out"=w157:refnum<class "Channel Manager.lvclass">)  [unwired: 7 in]
  }
  n133 = call-dynamic "Read Available Cameras.vi"("error in (no error)"=w41, "Channel Manager in"=w40) -> ("error out"=w37:errorcluster, "Available Cameras"=w39:u8, "Channel Manager out"=w38:refnum<class "Channel Manager.lvclass">)  [unwired: 7 in]
  n134 = for {
    N: w39 -> [_]
    shift-right: [w294] -> w56
    shift-left: w37 -> [w289]
    shift-right: [w293] -> w42
    shift-left: w38 -> [w290]
    i -> [w288]
    n135 = call-dynamic "Write Current Camera.vi"("error in (no error)"=w289, "Current Camera"=w288, "Channel Manager in"=w290) -> ("error out"=w292:errorcluster, "Channel Manager out"=w291:refnum<class "Channel Manager.lvclass">)  [unwired: 7 in]
    n136 = case shown="2" w288 {
      tunnel: [w308 w309 w310 w311] -> w295
      frame 0, Default {
        n137 = local read "Night Directory"() -> (w308:string)
      }
      frame 1 {
        n138 = local read "Night Directory"() -> (w309:string)
      }
      frame 2 {
        n139 = local read "Night Directory"() -> (w310:string)
      }
      frame 3 {
        n140 = local read "Night Directory"() -> (w311:string)
      }
    }
    n141 = call "Return Current RxTx.vi"("error in (no error)"=w292, "Channel Manager in"=w291) -> ("error out"=w306:errorcluster, "RxTx"=w307:refnum<class "RxTx.lvclass">, "Channel Manager out"=w304:refnum<class "Channel Manager.lvclass">)  [unwired: 7 in]
    n142 = call-dynamic "Read Interface.lvclass.vi"("error in (no error)"=w306, "RxTx in"=w307) -> ("error out"=w296:errorcluster, "Interface.lvclass"=w297:refnum<class "Interface.lvclass">, "RxTx out"=w305:refnum<class "RxTx.lvclass">)  [unwired: 7 in]
    n143 = call-dynamic "Write Image Path.vi"("error in (no error)"=w296, "Image Path"=w295, "Interface in"=w297) -> ("error out"=w299:errorcluster, "Interface out"=w298:refnum<class "Interface.lvclass">)  [unwired: 7 in]
    n144 = call-dynamic "Write Interface.lvclass.vi"("error in (no error)"=w299, "Interface.lvclass"=w298, "RxTx in"=w305) -> ("error out"=w303:errorcluster, "RxTx out"=w302:refnum<class "RxTx.lvclass">)  [unwired: 7 in]
    n145 = call "Enqeue A Message.vi"("error in (no error)"=w303, "RxTx in"=w302) -> ("error out"=w300:errorcluster, "RxTx out"=w301:refnum<class "RxTx.lvclass">)  [unwired: 8 in]
    n146 = call "Write Current RxTx.vi"("error in (no error)"=w300, "RxTx"=w301, "Channel Manager in"=w304) -> ("error out"=w294:errorcluster, "Channel Manager out"=w293:refnum<class "Channel Manager.lvclass">)  [unwired: 7 in]
  }
  n147 = call-dynamic "Write Channel Manager.lvclass.vi"("error in (no error)"=w56, "Channel Manager.lvclass"=w42, "SPARC4_AC in"=w69) -> ("error out"=w53:errorcluster, "SPARC4_AC out"=w52:refnum<class "SPARC4_AC.lvclass">)  [unwired: 7 in]
  n148 = while {
    shift-right: [w317] -> w77
    shift-left: w52 -> [w312]
    shift-right: [w315] -> _
    shift-left: w53 -> [w313]
    stop <- "Stop Button" stop-if-true
    n149 = event shown="[0] Timeout" {
      selector: _ -> [_ _ _ _ _ _ _ _ _ _ _ _ _ _ _ _ _ _ _ _ _ _ _ _ _ _ _ _ _ _ _ _ _ _ _ _ _ _ _ _ _ _ _ _ _ _ _ _ _ _ _ _ _ _ _ _ _ _ _ _]
      dyn-events: _ -> [_ _ _ _ _ _ _ _ _ _ _ _ _ _ _ _ _ _ _ _ _ _ _ _ _ _ _ _ _ _ _ _ _ _ _ _ _ _ _ _ _ _ _ _ _ _ _ _ _ _ _ _ _ _ _ _ _ _ _ _]
      timeout: 1 -> [_ _ _ _ _ _ _ _ _ _ _ _ _ _ _ _ _ _ _ _ _ _ _ _ _ _ _ _ _ _ _ _ _ _ _ _ _ _ _ _ _ _ _ _ _ _ _ _ _ _ _ _ _ _ _ _ _ _ _ _]
      tunnel: w313 -> [w345 w457 w481 w503 w526 w556 w589 w592 w598 w602 w637 w656 w723 w746 w769 w791 w822 w853 w857 w861 w866 w883 w921 w944 w1160 w1182 w1205 w1236 w1269 w1324 w1347 w1370 w1393 w1423 w1454 w1458 w1460 w1463 w1481 w1518 w1583 w1606 w1630 w1652 w1682 w1714 w1717 w1720 w1724 w1740 w1778 w1806 w2132 w2220 w2255 w2317 w2362 w2367 w2375 w2390]
      tunnel: w312 -> [w344 w458 w480 w502 w525 w555 w588 w591 w597 w601 w636 w657 w722 w745 w768 w792 w821 w854 w858 w862 w867 w884 w922 w943 w1161 w1181 w1204 w1235 w1268 w1323 w1346 w1369 w1392 w1422 w1455 w1457 w1461 w1464 w1480 w1519 w1584 w1607 w1629 w1653 w1683 w1715 w1718 w1721 w1723 w1739 w1779 w1807 w2133 w2221 w2256 w2316 w2363 w2366 w2374 w2391]
      tunnel: [w322 w456 w477 w500 w523 w553 w586 w592 w596 w602 w615 w656 w720 w743 w766 w789 w819 w851 w857 w860 w866 w881 w921 w941 w1156 w1179 w1203 w1233 w1265 w1321 w1344 w1367 w1390 w1420 w1453 w1458 w1460 w1463 w1478 w1518 w1581 w1604 w1627 w1650 w1680 w1712 w1717 w1720 w1724 w1737 w1778 w1793 w2135 w2223 w2258 w2319 w2362 w2367 w2375 w2390] -> w315
      tunnel: [w323 w455 w478 w501 w524 w554 w587 w591 w595 w601 w616 w657 w721 w744 w767 w790 w820 w852 w858 w859 w867 w882 w922 w940 w1157 w1180 w1202 w1234 w1264 w1322 w1345 w1368 w1391 w1421 w1452 w1457 w1461 w1464 w1479 w1519 w1582 w1605 w1628 w1651 w1681 w1713 w1718 w1721 w1723 w1738 w1779 w1792 w2134 w2222 w2257 w2318 w2363 w2366 w2374 w2391] -> w317
      event Timeout {
        n150 = event-data() -> ()  [unwired: 1 in, 1 out]
        n151 = call "RUN.vi"("error in (no error)"=w345, "SPARC4_AC in"=w344) -> ("error out"=w330:errorcluster, "SPARC4_AC out"=w331:refnum<class "SPARC4_AC.lvclass">)  [unwired: 8 in]
        n152 = call "Counter.vi"("error in (no error)"=w330, "Units"=u16 24000, "SPARC4_AC in"=w331) -> ("error out"=w333:errorcluster, "SPARC4_AC out"=w332:refnum<class "SPARC4_AC.lvclass">)  [unwired: 6 in, 1 out]
        n153 = call-dynamic "Read Channel Manager.lvclass.vi"("error in (no error)"=w333, "SPARC4_AC in"=w332) -> ("error out"=w337:errorcluster, "Channel Manager.lvclass"=w338:refnum<class "Channel Manager.lvclass">, "SPARC4_AC out"=w340:refnum<class "SPARC4_AC.lvclass">)  [unwired: 7 in]
        n154 = call-dynamic "Read Available Cameras.vi"("error in (no error)"=w337, "Channel Manager in"=w338) -> ("error out"=w334:errorcluster, "Available Cameras"=w336:u8, "Channel Manager out"=w335:refnum<class "Channel Manager.lvclass">)  [unwired: 7 in]
        n155 = for {
          N: w336 -> [_]
          tunnel: [w395] -> w343 mode=indexing
          tunnel: w335 -> [w392]
          tunnel: w334 -> [w393]
          tunnel: [w394] -> w339
          i -> [w389]
          n156 = call-dynamic "Write Current Camera.vi"("error in (no error)"=w393, "Current Camera"=w389, "Channel Manager in"=w392) -> ("error out"=w390:errorcluster, "Channel Manager out"=w391:refnum<class "Channel Manager.lvclass">)  [unwired: 7 in]
          n157 = call "Return Current RxTx.vi"("error in (no error)"=w390, "Channel Manager in"=w391) -> ("error out"=w396:errorcluster, "RxTx"=w397:refnum<class "RxTx.lvclass">)  [unwired: 7 in, 1 out]
          n158 = call-dynamic "Read Interface.lvclass.vi"("error in (no error)"=w396, "RxTx in"=w397) -> ("error out"=w399:errorcluster, "Interface.lvclass"=w398:refnum<class "Interface.lvclass">)  [unwired: 7 in, 1 out]
          n159 = call "Read Camera Status.vi"("error in (no error)"=w399, "Interface in"=w398) -> ("error out"=w394:errorcluster, "Camera Status"=w395:T6)  [unwired: 7 in, 1 out]
        }
        n160 = call "Update Interface indicator.vi"("error in (no error)"=w339, "Interval"=30.0, "SPARC4_AC in"=w340) -> ("error out"=w324:errorcluster, "update indicator?"=w341:bool, "SPARC4_AC out"=w325:refnum<class "SPARC4_AC.lvclass">)  [unwired: 6 in]
        n161 = case shown="True" w341 {
          tunnel: w343 -> [_ w346]
          frame False {
          }
          frame True {
            n162 = for {
              tunnel: w346 -> [w347] mode=indexing
              i -> [w348]
              n163 = case shown="1" w348 {
                tunnel: w347 -> [w349 w359 w374 w384]
                frame 0, Default {
                  n164 = Unbundle By Name(w349) -> ("% Acquired"=→"% Acquired":dbl, "Acquiring"=→"Exposing":bool, "Exposições realizadas"=→"Exposições realizadas":u32, "Current Temperature"=→"Temperature":dbl, "Temperatue Status"=w353:string)
                  n165 = case shown="\"TEMPERATURE STABILIZED\"" w353 {
                    frame "TEMPERATURE OFF", Default {
                      w355 = u32 14079702
                      n166 = property on="Temperature" class="DigNum (strict)"("NumText.BGColor"=w355) -> ()  [unwired: 2 in, 2 out]
                      n167 = property on="Temperature" class="DigNum (strict)"("NumText.BG Color"=w355) -> ()  [unwired: 2 in, 2 out]
                    }
                    frame "TEMPERATURE NOT STABILIZED" {
                      w356 = u32 16775680
                      n168 = property on="Temperature" class="DigNum (strict)"("NumText.BGColor"=w356) -> ()  [unwired: 2 in, 2 out]
                      n169 = property on="Temperature" class="DigNum (strict)"("NumText.BG Color"=w356) -> ()  [unwired: 2 in, 2 out]
                    }
                    frame "TEMPERATURE STABILIZED" {
                      w357 = u32 46100
                      n170 = property on="Temperature" class="DigNum (strict)"("NumText.BGColor"=w357) -> ()  [unwired: 2 in, 2 out]
                      n171 = property on="Temperature" class="DigNum (strict)"("NumText.BG Color"=w357) -> ()  [unwired: 2 in, 2 out]
                    }
                    frame "TEMPERATURE NOT REACHED" {
                      w358 = u32 16716346
                      n172 = property on="Temperature" class="DigNum (strict)"("NumText.BGColor"=w358) -> ()  [unwired: 2 in, 2 out]
                      n173 = property on="Temperature" class="DigNum (strict)"("NumText.BG Color"=w358) -> ()  [unwired: 2 in, 2 out]
                    }
                  }
                }
                frame 1 {
                  n174 = Unbundle By Name(w359) -> ("% Acquired"=→"% Acquired 2":dbl, "Acquiring"=→"Exposing 2":bool, "Exposições realizadas"=→"Exposições realizadas 2":u32, "Current Temperature"=→"Temperature 2":dbl, "Temperatue Status"=w364:string)
                  n175 = case shown="\"TEMPERATURE STABILIZED\"" w364 {
                    frame "TEMPERATURE OFF", Default {
                      w365 = u32 14079702
                      n176 = property on="Temperature 2" class="DigNum (strict)"("NumText.BGColor"=w365) -> ()  [unwired: 2 in, 2 out]
                      n177 = property on="Temperature 2" class="DigNum (strict)"("NumText.BG Color"=w365) -> ()  [unwired: 2 in, 2 out]
                    }
                    frame "TEMPERATURE NOT STABILIZED" {
                      w366 = u32 16775680
                      n178 = property on="Temperature 2" class="DigNum (strict)"("NumText.BGColor"=w366) -> ()  [unwired: 2 in, 2 out]
                      n179 = property on="Temperature 2" class="DigNum (strict)"("NumText.BG Color"=w366) -> ()  [unwired: 2 in, 2 out]
                    }
                    frame "TEMPERATURE STABILIZED" {
                      w367 = u32 46100
                      n180 = property on="Temperature 2" class="DigNum (strict)"("NumText.BGColor"=w367) -> ()  [unwired: 2 in, 2 out]
                      n181 = property on="Temperature 2" class="DigNum (strict)"("NumText.BG Color"=w367) -> ()  [unwired: 2 in, 2 out]
                    }
                    frame "TEMPERATURE NOT REACHED" {
                      w368 = u32 16716346
                      n182 = property on="Temperature 2" class="DigNum (strict)"("NumText.BGColor"=w368) -> ()  [unwired: 2 in, 2 out]
                      n183 = property on="Temperature 2" class="DigNum (strict)"("NumText.BG Color"=w368) -> ()  [unwired: 2 in, 2 out]
                    }
                  }
                }
                frame 2 {
                  n184 = Unbundle By Name(w374) -> ("% Acquired"=→"% Acquired 3":dbl, "Acquiring"=→"Exposing 3":bool, "Exposições realizadas"=→"Exposições realizadas 3":u32, "Current Temperature"=→"Temperature 3":dbl, "Temperatue Status"=w370:string)
                  n185 = case shown="\"TEMPERATURE STABILIZED\"" w370 {
                    frame "TEMPERATURE OFF", Default {
                      w375 = u32 14079702
                      n186 = property on="Temperature 3" class="DigNum (strict)"("NumText.BGColor"=w375) -> ()  [unwired: 2 in, 2 out]
                      n187 = property on="Temperature 3" class="DigNum (strict)"("NumText.BG Color"=w375) -> ()  [unwired: 2 in, 2 out]
                    }
                    frame "TEMPERATURE NOT STABILIZED" {
                      w376 = u32 16775680
                      n188 = property on="Temperature 2" class="DigNum (strict)"("NumText.BGColor"=w376) -> ()  [unwired: 2 in, 2 out]
                      n189 = property on="Temperature 2" class="DigNum (strict)"("NumText.BG Color"=w376) -> ()  [unwired: 2 in, 2 out]
                    }
                    frame "TEMPERATURE STABILIZED" {
                      w377 = u32 46100
                      n190 = property on="Temperature 2" class="DigNum (strict)"("NumText.BGColor"=w377) -> ()  [unwired: 2 in, 2 out]
                      n191 = property on="Temperature 2" class="DigNum (strict)"("NumText.BG Color"=w377) -> ()  [unwired: 2 in, 2 out]
                    }
                    frame "TEMPERATURE NOT REACHED" {
                      w378 = u32 16716346
                      n192 = property on="Temperature 2" class="DigNum (strict)"("NumText.BGColor"=w378) -> ()  [unwired: 2 in, 2 out]
                      n193 = property on="Temperature 2" class="DigNum (strict)"("NumText.BG Color"=w378) -> ()  [unwired: 2 in, 2 out]
                    }
                  }
                }
                frame 3 {
                  n194 = Unbundle By Name(w384) -> ("% Acquired"=→"% Acquired 4":dbl, "Acquiring"=→"Exposing 4":bool, "Exposições realizadas"=→"Exposições realizadas 4":u32, "Current Temperature"=→"Temperature 4":dbl, "Temperatue Status"=w383:string)
                  n195 = case shown="\"TEMPERATURE STABILIZED\"" w383 {
                    frame "TEMPERATURE OFF", Default {
                      w385 = u32 14079702
                      n196 = property on="Temperature 4" class="DigNum (strict)"("NumText.BGColor"=w385) -> ()  [unwired: 2 in, 2 out]
                      n197 = property on="Temperature 4" class="DigNum (strict)"("NumText.BG Color"=w385) -> ()  [unwired: 2 in, 2 out]
                    }
                    frame "TEMPERATURE NOT STABILIZED" {
                      w386 = u32 16775680
                      n198 = property on="Temperature 2" class="DigNum (strict)"("NumText.BGColor"=w386) -> ()  [unwired: 2 in, 2 out]
                      n199 = property on="Temperature 2" class="DigNum (strict)"("NumText.BG Color"=w386) -> ()  [unwired: 2 in, 2 out]
                    }
                    frame "TEMPERATURE STABILIZED" {
                      w387 = u32 46100
                      n200 = property on="Temperature 2" class="DigNum (strict)"("NumText.BGColor"=w387) -> ()  [unwired: 2 in, 2 out]
                      n201 = property on="Temperature 2" class="DigNum (strict)"("NumText.BG Color"=w387) -> ()  [unwired: 2 in, 2 out]
                    }
                    frame "TEMPERATURE NOT REACHED" {
                      w388 = u32 16716346
                      n202 = property on="Temperature 2" class="DigNum (strict)"("NumText.BGColor"=w388) -> ()  [unwired: 2 in, 2 out]
                      n203 = property on="Temperature 2" class="DigNum (strict)"("NumText.BG Color"=w388) -> ()  [unwired: 2 in, 2 out]
                    }
                  }
                }
              }
            }
          }
        }
        n204 = call-dynamic "Read Readout Charact.lvclass.vi"("error in (no error)"=w324, "SPARC4_AC in"=w325) -> ("error out"=w320:errorcluster, "Readout Charact.lvclass"=w321:refnum<class "Readout Charact.lvclass">, "SPARC4_AC out"=w328:refnum<class "SPARC4_AC.lvclass">)  [unwired: 7 in]
        n205 = call-dynamic "Read String of the times.vi"("error in (no error)"=w320, "Readout Charact in"=w321) -> ("error out"=w326:errorcluster, "String of the times"=→"String":string, "Readout Charact out"=w327:refnum<class "Readout Charact.lvclass">)  [unwired: 7 in]
        n206 = call-dynamic "Write Readout Charact.lvclass.vi"("error in (no error)"=w326, "Readout Charact.lvclass"=w327, "SPARC4_AC in"=w328) -> ("error out"=w322:errorcluster, "SPARC4_AC out"=w323:refnum<class "SPARC4_AC.lvclass">)  [unwired: 7 in]
      }
      event "Adquirir": Value Change {
        w450 = u8 0 items=["Normal", "+1", "+2", "+3", "+4"] ("Vertical Clock Amplitude")
        w419 = u8 0 items=["0.6", "1.13", "2.2", "4.33"] ("Vertical Shift Speed")
        w423 = u8 4 items=["Full Vertical Binning", "Multi-Track", "Random-track", "Single-Track", "Image"] ("Read Mode")
        w425 = u8 3 items=["N/A", "Single", "Accumulate", "Kinetic", "Fast Kinetic"] ("Acquisition Mode")
        w424 = u8 6 items=["Internal", "External", "RESERVED", "RESERVED", "RESERVED", "RESERVED", "External Start"] ("Trigger")
        w416 = u8 2 items=["Fully Auto", "OPEN", "CLOSED"] ("Shutter Mode")
        w415 = u8 0 items=["TTL Low", "TTl High"] ("Shutter TTL")
        w401 = u16 50 ("Time to open shutter")
        n207 = event-data() -> ()  [unwired: 1 in, 1 out]
        n208 = local read "Night Directory"() -> (w400:string)
        n209 = call-dynamic "Read Channel Manager.lvclass.vi"("error in (no error)"=w457, "SPARC4_AC in"=w458) -> ("error out"=w408:errorcluster, "Channel Manager.lvclass"=w409:refnum<class "Channel Manager.lvclass">, "SPARC4_AC out"=w454:refnum<class "SPARC4_AC.lvclass">)  [unwired: 7 in]
        n210 = call-dynamic "Write Current Camera.vi"("error in (no error)"=w408, "Current Camera"=0, "Channel Manager in"=w409) -> ("error out"=w411:errorcluster, "Channel Manager out"=w412:refnum<class "Channel Manager.lvclass">)  [unwired: 7 in]
        n211 = call "Return Current RxTx.vi"("error in (no error)"=w411, "Channel Manager in"=w412) -> ("error out"=w439:errorcluster, "RxTx"=w438:refnum<class "RxTx.lvclass">, "Channel Manager out"=w435:refnum<class "Channel Manager.lvclass">)  [unwired: 7 in]
        n212 = Bundle By Name(cluster="Camera Setup", "Image Name"="Image Name", "Image Path"=w400, "# Images"="# Ciclos", "Number of exp"="# Ciclos", "Exposure Time"="Exposure Time 2", "Pre-amp gain"="Pre-amp gain", "Readout Rate"="Readout Rate", "Vertical Shift Speed"=w419, "Acquisition Mode"=w425, "Trigger"=w424, "Read Mode"=w423, "EM Mode"="EM Mode", "EM Gain"="EM Gain", "Shutter Mode"=w416, "Shutter TTL"=w415, "Time to open shutter"=w401, "Time to close shutter"=w401, "Vertical Binning"="Binning 5", "Horizontal Binning"="Binning 5", "Initial Line"="Initial Line", "Initial Cloumn"="Initial Cloumn", "Final Line"="Final Line", "Final Column"="Final Column", "Exposições realizadas"=u8 0, "Kinetic Serie Length"="Kinetic Series Length", "Frame Transfer"=TRUE, "Vertical Clock Amplitude"=w450) -> (w430:T1)
        n213 = call-dynamic "Read Interface.lvclass.vi"("error in (no error)"=w439, "RxTx in"=w438) -> ("error out"=w433:errorcluster, "Interface.lvclass"=w434:refnum<class "Interface.lvclass">, "RxTx out"=w429:refnum<class "RxTx.lvclass">)  [unwired: 7 in]
        n214 = call-dynamic "Write Exposições realizadas.vi"("error in (no error)"=w433, "Exposições realizadas"=0, "Interface in"=w434) -> ("error out"=w431:errorcluster, "Interface out"=w432:refnum<class "Interface.lvclass">)  [unwired: 7 in]
        n215 = call "Write Camera Setup.vi"("error in (no error)"=w431, "Camera Setup"=w430, "Interface in"=w432) -> ("error out"=w427:errorcluster, "Interface out"=w428:refnum<class "Interface.lvclass">)  [unwired: 7 in]
        n216 = call-dynamic "Write Interface.lvclass.vi"("error in (no error)"=w427, "Interface.lvclass"=w428, "RxTx in"=w429) -> ("error out"=w437:errorcluster, "RxTx out"=w436:refnum<class "RxTx.lvclass">)  [unwired: 7 in]
        n217 = call "Write Current RxTx.vi"("error in (no error)"=w437, "RxTx"=w436, "Channel Manager in"=w435) -> ("error out"=w441:errorcluster, "Channel Manager out"=w440:refnum<class "Channel Manager.lvclass">)  [unwired: 7 in]
        n218 = call "Read Current State Machine.vi"("error in (no error)"=w441, "Channel Manager in"=w440) -> ("error out"=w443:errorcluster, "State Machine.lvclass"=w442:refnum<class "State Machine.lvclass">, "Channel Manager out"=w446:refnum<class "Channel Manager.lvclass">)  [unwired: 7 in]
        n219 = call "Next State.vi"("error in (no error)"=w443, "New_State"=u32 17, "State Machine in"=w442) -> ("error out"=w444:errorcluster, "State Machine out"=w445:refnum<class "State Machine.lvclass">)  [unwired: 7 in]
        n220 = call "Write Current State Machine.vi"("error in (no error)"=w444, "State Machine.lvclass"=w445, "Channel Manager in"=w446) -> ("error out"=w453:errorcluster, "Channel Manager out"=w407:refnum<class "Channel Manager.lvclass">)  [unwired: 7 in]
        n221 = call-dynamic "Write Channel Manager.lvclass.vi"("error in (no error)"=w453, "Channel Manager.lvclass"=w407, "SPARC4_AC in"=w454) -> ("error out"=w456:errorcluster, "SPARC4_AC out"=w455:refnum<class "SPARC4_AC.lvclass">)  [unwired: 7 in]
      }
      event "Stop Acq": Value Change {
        n222 = event-data() -> ()  [unwired: 1 in, 1 out]
        n223 = call-dynamic "Read Channel Manager.lvclass.vi"("error in (no error)"=w481, "SPARC4_AC in"=w480) -> ("error out"=w460:errorcluster, "Channel Manager.lvclass"=w459:refnum<class "Channel Manager.lvclass">, "SPARC4_AC out"=w479:refnum<class "SPARC4_AC.lvclass">)  [unwired: 7 in]
        n224 = call-dynamic "Write Current Camera.vi"("error in (no error)"=w460, "Current Camera"=0, "Channel Manager in"=w459) -> ("error out"=w463:errorcluster, "Channel Manager out"=w462:refnum<class "Channel Manager.lvclass">)  [unwired: 7 in]
        n225 = call "Return Current RxTx.vi"("error in (no error)"=w463, "Channel Manager in"=w462) -> ("error out"=w473:errorcluster, "RxTx"=w472:refnum<class "RxTx.lvclass">, "Channel Manager out"=w465:refnum<class "Channel Manager.lvclass">)  [unwired: 7 in]
        n226 = call-dynamic "Read Interface.lvclass.vi"("error in (no error)"=w473, "RxTx in"=w472) -> ("error out"=w468:errorcluster, "Interface.lvclass"=w467:refnum<class "Interface.lvclass">, "RxTx out"=w471:refnum<class "RxTx.lvclass">)  [unwired: 7 in]
        n227 = call-dynamic "Write Stop Acq.vi"("error in (no error)"=w468, "Stop Acq"="Stop Acq", "Interface in"=w467) -> ("error out"=w469:errorcluster, "Interface out"=w470:refnum<class "Interface.lvclass">)  [unwired: 7 in]
        n228 = call-dynamic "Write Interface.lvclass.vi"("error in (no error)"=w469, "Interface.lvclass"=w470, "RxTx in"=w471) -> ("error out"=w475:errorcluster, "RxTx out"=w474:refnum<class "RxTx.lvclass">)  [unwired: 7 in]
        n229 = call "Write Current RxTx.vi"("error in (no error)"=w475, "RxTx"=w474, "Channel Manager in"=w465) -> ("error out"=w476:errorcluster, "Channel Manager out"=w464:refnum<class "Channel Manager.lvclass">)  [unwired: 7 in]
        n230 = call-dynamic "Write Channel Manager.lvclass.vi"("error in (no error)"=w476, "Channel Manager.lvclass"=w464, "SPARC4_AC in"=w479) -> ("error out"=w477:errorcluster, "SPARC4_AC out"=w478:refnum<class "SPARC4_AC.lvclass">)  [unwired: 7 in]
      }
      event "Pausar": Value Change {
        n231 = event-data() -> ()  [unwired: 1 in, 1 out]
        n232 = call-dynamic "Read Channel Manager.lvclass.vi"("error in (no error)"=w503, "SPARC4_AC in"=w502) -> ("error out"=w484:errorcluster, "Channel Manager.lvclass"=w483:refnum<class "Channel Manager.lvclass">, "SPARC4_AC out"=w504:refnum<class "SPARC4_AC.lvclass">)  [unwired: 7 in]
        n233 = call-dynamic "Write Current Camera.vi"("error in (no error)"=w484, "Current Camera"=0, "Channel Manager in"=w483) -> ("error out"=w488:errorcluster, "Channel Manager out"=w487:refnum<class "Channel Manager.lvclass">)  [unwired: 7 in]
        n234 = call "Return Current RxTx.vi"("error in (no error)"=w488, "Channel Manager in"=w487) -> ("error out"=w492:errorcluster, "RxTx"=w491:refnum<class "RxTx.lvclass">, "Channel Manager out"=w489:refnum<class "Channel Manager.lvclass">)  [unwired: 7 in]
        n235 = call-dynamic "Read Interface.lvclass.vi"("error in (no error)"=w492, "RxTx in"=w491) -> ("error out"=w498:errorcluster, "Interface.lvclass"=w495:refnum<class "Interface.lvclass">, "RxTx out"=w490:refnum<class "RxTx.lvclass">)  [unwired: 7 in]
        n236 = call-dynamic "Write Pause Acq.vi"("error in (no error)"=w498, "Pause Acq"="Pausar", "Interface in"=w495) -> ("error out"=w497:errorcluster, "Interface out"=w496:refnum<class "Interface.lvclass">)  [unwired: 7 in]
        n237 = call-dynamic "Write Interface.lvclass.vi"("error in (no error)"=w497, "Interface.lvclass"=w496, "RxTx in"=w490) -> ("error out"=w494:errorcluster, "RxTx out"=w493:refnum<class "RxTx.lvclass">)  [unwired: 7 in]
        n238 = call "Write Current RxTx.vi"("error in (no error)"=w494, "RxTx"=w493, "Channel Manager in"=w489) -> ("error out"=w485:errorcluster, "Channel Manager out"=w486:refnum<class "Channel Manager.lvclass">)  [unwired: 7 in]
        n239 = call-dynamic "Write Channel Manager.lvclass.vi"("error in (no error)"=w485, "Channel Manager.lvclass"=w486, "SPARC4_AC in"=w504) -> ("error out"=w500:errorcluster, "SPARC4_AC out"=w501:refnum<class "SPARC4_AC.lvclass">)  [unwired: 7 in]
      }
      event "Abort": Value Change {
        n240 = event-data() -> ()  [unwired: 1 in, 1 out]
        n241 = call-dynamic "Read Channel Manager.lvclass.vi"("error in (no error)"=w526, "SPARC4_AC in"=w525) -> ("error out"=w506:errorcluster, "Channel Manager.lvclass"=w507:refnum<class "Channel Manager.lvclass">, "SPARC4_AC out"=w527:refnum<class "SPARC4_AC.lvclass">)  [unwired: 7 in]
        n242 = call-dynamic "Write Current Camera.vi"("error in (no error)"=w506, "Current Camera"=0, "Channel Manager in"=w507) -> ("error out"=w511:errorcluster, "Channel Manager out"=w510:refnum<class "Channel Manager.lvclass">)  [unwired: 7 in]
        n243 = call "Return Current RxTx.vi"("error in (no error)"=w511, "Channel Manager in"=w510) -> ("error out"=w514:errorcluster, "RxTx"=w513:refnum<class "RxTx.lvclass">, "Channel Manager out"=w517:refnum<class "Channel Manager.lvclass">)  [unwired: 7 in]
        n244 = call-dynamic "Read Interface.lvclass.vi"("error in (no error)"=w514, "RxTx in"=w513) -> ("error out"=w521:errorcluster, "Interface.lvclass"=w520:refnum<class "Interface.lvclass">, "RxTx out"=w512:refnum<class "RxTx.lvclass">)  [unwired: 7 in]
        n245 = call-dynamic "Write Abort.vi"("error in (no error)"=w521, "Abort"="Abort", "Interface in"=w520) -> ("error out"=w522:errorcluster, "Interface out"=w518:refnum<class "Interface.lvclass">)  [unwired: 7 in]
        n246 = call-dynamic "Write Interface.lvclass.vi"("error in (no error)"=w522, "Interface.lvclass"=w518, "RxTx in"=w512) -> ("error out"=w516:errorcluster, "RxTx out"=w515:refnum<class "RxTx.lvclass">)  [unwired: 7 in]
        n247 = call "Write Current RxTx.vi"("error in (no error)"=w516, "RxTx"=w515, "Channel Manager in"=w517) -> ("error out"=w508:errorcluster, "Channel Manager out"=w509:refnum<class "Channel Manager.lvclass">)  [unwired: 7 in]
        n248 = call-dynamic "Write Channel Manager.lvclass.vi"("error in (no error)"=w508, "Channel Manager.lvclass"=w509, "SPARC4_AC in"=w527) -> ("error out"=w523:errorcluster, "SPARC4_AC out"=w524:refnum<class "SPARC4_AC.lvclass">)  [unwired: 7 in]
      }
      event "Cooler ON/OFF": Value Change {
        n249 = event-data() -> ()  [unwired: 1 in, 1 out]
        n250 = call-dynamic "Read Channel Manager.lvclass.vi"("error in (no error)"=w556, "SPARC4_AC in"=w555) -> ("error out"=w529:errorcluster, "Channel Manager.lvclass"=w530:refnum<class "Channel Manager.lvclass">, "SPARC4_AC out"=w557:refnum<class "SPARC4_AC.lvclass">)  [unwired: 7 in]
        n251 = call-dynamic "Write Current Camera.vi"("error in (no error)"=w529, "Current Camera"=0, "Channel Manager in"=w530) -> ("error out"=w533:errorcluster, "Channel Manager out"=w532:refnum<class "Channel Manager.lvclass">)  [unwired: 7 in]
        n252 = local read "Camera Setup"() -> (w551:T1)
        n253 = case shown="0, Default" "Cooler ON/OFF" {
          tunnel: ["TURN COOLER OFF" "TURN COOLER ON"] -> w543
          frame 0, Default {
            n254 = local write "Set temperature"(i8 20 ("Set temperature")) -> ()
          }
          frame 1 {
          }
        }
        n255 = Bundle By Name(cluster=w551, "Cooler ON/OFF"="Cooler ON/OFF") -> (w536:T1)
        n256 = call "Return Current RxTx.vi"("error in (no error)"=w533, "Channel Manager in"=w532) -> ("error out"=w550:errorcluster, "RxTx"=w549:refnum<class "RxTx.lvclass">, "Channel Manager out"=w534:refnum<class "Channel Manager.lvclass">)  [unwired: 7 in]
        n257 = call-dynamic "Read Interface.lvclass.vi"("error in (no error)"=w550, "RxTx in"=w549) -> ("error out"=w537:errorcluster, "Interface.lvclass"=w535:refnum<class "Interface.lvclass">, "RxTx out"=w546:refnum<class "RxTx.lvclass">)  [unwired: 7 in]
        n258 = call "Write Camera Setup.vi"("error in (no error)"=w537, "Camera Setup"=w536, "Interface in"=w535) -> ("error out"=w545:errorcluster, "Interface out"=w544:refnum<class "Interface.lvclass">)  [unwired: 7 in]
        n259 = call "Write Command.vi"("error in (no error)"=w545, "Command"=w543, "Interface in"=w544) -> ("error out"=w540:errorcluster, "Interface out"=w541:refnum<class "Interface.lvclass">)  [unwired: 7 in]
        n260 = call-dynamic "Write Interface.lvclass.vi"("error in (no error)"=w540, "Interface.lvclass"=w541, "RxTx in"=w546) -> ("error out"=w538:errorcluster, "RxTx out"=w539:refnum<class "RxTx.lvclass">)  [unwired: 7 in]
        n261 = call "Enqeue A Message.vi"("error in (no error)"=w538, "RxTx in"=w539) -> ("error out"=w548:errorcluster, "RxTx out"=w547:refnum<class "RxTx.lvclass">)  [unwired: 8 in]
        n262 = call "Write Current RxTx.vi"("error in (no error)"=w548, "RxTx"=w547, "Channel Manager in"=w534) -> ("error out"=w552:errorcluster, "Channel Manager out"=w531:refnum<class "Channel Manager.lvclass">)  [unwired: 7 in]
        n263 = call-dynamic "Write Channel Manager.lvclass.vi"("error in (no error)"=w552, "Channel Manager.lvclass"=w531, "SPARC4_AC in"=w557) -> ("error out"=w553:errorcluster, "SPARC4_AC out"=w554:refnum<class "SPARC4_AC.lvclass">)  [unwired: 7 in]
      }
      event "Set temperature": Value Change {
        n264 = event-data() -> ()  [unwired: 1 in, 1 out]
        n265 = call-dynamic "Read Channel Manager.lvclass.vi"("error in (no error)"=w589, "SPARC4_AC in"=w588) -> ("error out"=w563:errorcluster, "Channel Manager.lvclass"=w562:refnum<class "Channel Manager.lvclass">, "SPARC4_AC out"=w590:refnum<class "SPARC4_AC.lvclass">)  [unwired: 7 in]
        n266 = call-dynamic "Write Current Camera.vi"("error in (no error)"=w563, "Current Camera"=0, "Channel Manager in"=w562) -> ("error out"=w565:errorcluster, "Channel Manager out"=w564:refnum<class "Channel Manager.lvclass">)  [unwired: 7 in]
        n267 = call "Return Current RxTx.vi"("error in (no error)"=w565, "Channel Manager in"=w564) -> ("error out"=w568:errorcluster, "RxTx"=w571:refnum<class "RxTx.lvclass">, "Channel Manager out"=w572:refnum<class "Channel Manager.lvclass">)  [unwired: 7 in]
        n268 = call-dynamic "Read Interface.lvclass.vi"("error in (no error)"=w568, "RxTx in"=w571) -> ("error out"=w577:errorcluster, "Interface.lvclass"=w576:refnum<class "Interface.lvclass">, "RxTx out"=w584:refnum<class "RxTx.lvclass">)  [unwired: 7 in]
        n269 = local read "Camera Setup"() -> (w567:T1)
        n270 = Bundle By Name(cluster=w567, "Set temperature"="Set temperature") -> (w575:T1)
        n271 = call "Write Camera Setup.vi"("error in (no error)"=w577, "Camera Setup"=w575, "Interface in"=w576) -> ("error out"=w574:errorcluster, "Interface out"=w573:refnum<class "Interface.lvclass">)  [unwired: 7 in]
        n272 = call "Write Command.vi"("error in (no error)"=w574, "Command"="SET TEMPERATURE", "Interface in"=w573) -> ("error out"=w582:errorcluster, "Interface out"=w583:refnum<class "Interface.lvclass">)  [unwired: 7 in]
        n273 = call-dynamic "Write Interface.lvclass.vi"("error in (no error)"=w582, "Interface.lvclass"=w583, "RxTx in"=w584) -> ("error out"=w580:errorcluster, "RxTx out"=w581:refnum<class "RxTx.lvclass">)  [unwired: 7 in]
        n274 = call "Enqeue A Message.vi"("error in (no error)"=w580, "RxTx in"=w581) -> ("error out"=w569:errorcluster, "RxTx out"=w570:refnum<class "RxTx.lvclass">)  [unwired: 8 in]
        n275 = call "Write Current RxTx.vi"("error in (no error)"=w569, "RxTx"=w570, "Channel Manager in"=w572) -> ("error out"=w585:errorcluster, "Channel Manager out"=w566:refnum<class "Channel Manager.lvclass">)  [unwired: 7 in]
        n276 = call-dynamic "Write Channel Manager.lvclass.vi"("error in (no error)"=w585, "Channel Manager.lvclass"=w566, "SPARC4_AC in"=w590) -> ("error out"=w586:errorcluster, "SPARC4_AC out"=w587:refnum<class "SPARC4_AC.lvclass">)  [unwired: 7 in]
        "Temperature ºC" <- "Set temperature"
      }
      event "Exposure Time": Value Change {
        n277 = event-data() -> ()  [unwired: 1 in, 1 out]
        n278 = local write "Exposure Time 2"("Exposure Time") -> ()
      }
      event "# Ciclos": Value Change {
        n279 = event-data() -> ()  [unwired: 1 in, 1 out]
        n280 = local read "# Ciclos"() -> (w599:u32)
        n281 = property on="Exposições realizadas" class="Slide (strict)"("Scale.Maximum"=w599) -> ()  [unwired: 2 in, 2 out]
        n282 = call-dynamic "Read Sync Mode.vi"("error in (no error)"=w598, "SPARC4_AC in"=w597) -> ("error out"=w596:errorcluster, "Sync Mode"=w594:u16, "SPARC4_AC out"=w595:refnum<class "SPARC4_AC.lvclass">)  [unwired: 7 in]
        n283 = case shown="1, Default" w594 {
          frame 0 {
          }
          frame 1, Default {
            n284 = local read "# Ciclos"() -> (w600:u32)
            n285 = local write "# Images 2"(w600) -> ()
            n286 = property on="Exposições realizadas 2" class="Slide (strict)"("Scale.Maximum"=w600) -> ()  [unwired: 2 in, 2 out]
          }
        }
      }
      event "Exposure Time 2": Value Change {
        n287 = event-data() -> ()  [unwired: 1 in, 1 out]
        n288 = local read "Exposure Time 2"() -> (w603:dbl)
        n289 = local write "Exposure Time"(w603) -> ()
      }
      event "Sub Image": Value Change {
        n290 = event-data() -> ()  [unwired: 1 in, 1 out]
        n291 = call-dynamic "Read Channel Manager.lvclass.vi"("error in (no error)"=w637, "SPARC4_AC in"=w636) -> ("error out"=w610:errorcluster, "Channel Manager.lvclass"=w611:refnum<class "Channel Manager.lvclass">, "SPARC4_AC out"=w619:refnum<class "SPARC4_AC.lvclass">)  [unwired: 7 in]
        n292 = call-dynamic "Write Current Camera.vi"("error in (no error)"=w610, "Current Camera"=0, "Channel Manager in"=w611) -> ("error out"=w613:errorcluster, "Channel Manager out"=w612:refnum<class "Channel Manager.lvclass">)  [unwired: 7 in]
        n293 = call "Return Current RxTx.vi"("error in (no error)"=w613, "Channel Manager in"=w612) -> ("error out"=w634:errorcluster, "RxTx"=w635:refnum<class "RxTx.lvclass">, "Channel Manager out"=w608:refnum<class "Channel Manager.lvclass">)  [unwired: 7 in]
        n294 = call-dynamic "Read Interface.lvclass.vi"("error in (no error)"=w634, "RxTx in"=w635) -> ("error out"=w632:errorcluster, "Interface.lvclass"=w633:refnum<class "Interface.lvclass">)  [unwired: 7 in, 1 out]
        n295 = call "Read Camera Status.vi"("error in (no error)"=w632, "Interface in"=w633) -> ("error out"=w620:errorcluster, "Camera Status"=w631:T6)  [unwired: 7 in, 1 out]
        n296 = Unbundle By Name(w631) -> ("Final Column"=w626:u16, "Final Line"=w625:u16)
        n297 = call-dynamic "Write Channel Manager.lvclass.vi"("error in (no error)"=w620, "Channel Manager.lvclass"=w608, "SPARC4_AC in"=w619) -> ("error out"=w618:errorcluster, "SPARC4_AC out"=w617:refnum<class "SPARC4_AC.lvclass">)  [unwired: 7 in]
        n298 = case shown="\"1024 x 1024\", Default" "Sub Image" {
          tunnel: [128 256 512 512] -> w624
          frame "256 x 256" {
          }
          frame "512 x 512" {
          }
          frame "1024 x 1024", Default {
          }
          frame "Custom" {
          }
        }
        n299 = case shown="\"1024 x 1024\", Default" "Sub Image" {
          tunnel: [T7."Disabled and Grayed Out" ("Disabled") T7."Enabled" ("Disabled")] -> w614
          frame "1024 x 1024", Default {
          }
          frame "Custom" {
          }
        }
        n300 = Divide(x=w626, y=2) -> (x/y=w629:dbl)
        n301 = Divide(x=w625, y=2) -> (x/y=w630:dbl)
        n302 = Add(x=w629, y=w624) -> (x+y=w607:dbl)
        n303 = Subtract(x=w629, y=w624) -> (x-y=w623:dbl)
        n304 = Subtract(x=w630, y=w624) -> (x-y=w622:dbl)
        n305 = Add(x=w630, y=w624) -> (x+y=w605:dbl)
        n306 = Increment(x=w623) -> (x+1=w606:dbl)
        n307 = Increment(x=w622) -> (x+1=w604:dbl)
        n308 = local write "Final Column"(w607) -> ()
        n309 = local write "Final Line"(w605) -> ()
        n310 = local write "Initial Cloumn"(w606) -> ()
        n311 = local write "Initial Line"(w604) -> ()
        n312 = property on="Initial Line" class="DigNum (strict)"("DisabledEnum"=w614) -> ()  [unwired: 2 in, 2 out]
        n313 = property on="Initial Cloumn" class="DigNum (strict)"("DisabledEnum"=w614) -> ()  [unwired: 2 in, 2 out]
        n314 = property on="Final Line" class="DigNum (strict)"("DisabledEnum"=w614) -> ()  [unwired: 2 in, 2 out]
        n315 = property on="Final Column" class="DigNum (strict)"("DisabledEnum"=w614) -> ()  [unwired: 2 in, 2 out]
        n316 = flat-sequence {
          tunnel: w618 -> [w648]
          tunnel: w617 -> [w649]
          tunnel: [w649] -> w616
          tunnel: [w648] -> w615
          frame #0 {
            w642 = cluster{dbl, dbl} {0.0, 0.0}
            n317 = local read "Initial Cloumn"() -> (w641:u16)
            n318 = local read "Final Column"() -> (w639:u16)
            n319 = local read "Initial Line"() -> (w640:u16)
            n320 = local read "Final Line"() -> (w638:u16)
            n321 = Bundle(cluster=w642, w641, w640) -> (w647:cluster{dbl, dbl})
            n322 = Bundle(cluster=w642, w641, w638) -> (w646:cluster{dbl, dbl})
            n323 = Bundle(cluster=w642, w639, w638) -> (w645:cluster{dbl, dbl})
            n324 = Bundle(cluster=w642, w639, w640) -> (w644:cluster{dbl, dbl})
            n325 = Bundle(cluster=w642, w641, w640) -> (w643:cluster{dbl, dbl})
            n326 = Build Array(w647, w646, w645, w644, w643) -> ()  [unwired: 1 out]
          }
        }
      }
      event "Initial Line", "Initial Cloumn", "Final Line", "Final Column": Value Change {
        n327 = event-data() -> ()  [unwired: 1 in, 1 out]
        n328 = disable-structure shown="Disabled" {
          frame Disabled {
            w659 = cluster{dbl, dbl} {0.0, 0.0}
            n329 = local read "Initial Cloumn"() -> (w663:u16)
            n330 = local read "Final Column"() -> (w661:u16)
            n331 = local read "Initial Line"() -> (w662:u16)
            n332 = local read "Final Line"() -> (w660:u16)
            n333 = Bundle(cluster=w659, w663, w662) -> (w668:cluster{dbl, dbl})
            n334 = Bundle(cluster=w659, w663, w660) -> (w667:cluster{dbl, dbl})
            n335 = Bundle(cluster=w659, w661, w660) -> (w666:cluster{dbl, dbl})
            n336 = Bundle(cluster=w659, w661, w662) -> (w665:cluster{dbl, dbl})
            n337 = Bundle(cluster=w659, w663, w662) -> (w664:cluster{dbl, dbl})
            n338 = Build Array(w668, w667, w666, w665, w664) -> (w658:cluster{dbl, dbl}[])
            n339 = local write item#-1(w658) -> ()
          }
          frame Enabled {
          }
        }
      }
      event "Adquirir 2": Value Change {
        w673 = u8 4 items=["Full Vertical Binning", "Multi-Track", "Random-track", "Single-Track", "Image"] ("Read Mode")
        w676 = u8 3 items=["0.6", "1.13", "2.2", "4.33"] ("Vertical Shift \nSpeed")
        w674 = u8 3 items=["N/A", "Single", "Accumulate", "Kinetic", "Fast Kinetic"] ("Acquisition Mode")
        w675 = u8 6 items=["Internal", "External", "RESERVED", "RESERVED", "RESERVED", "RESERVED", "External Start"] ("Trigger")
        w672 = u8 2 items=["Fully Auto", "OPEN", "CLOSED"] ("Shutter Mode")
        w671 = u8 0 items=["TTL Low", "TTl High"] ("Shutter TTL")
        w670 = u16 50 ("Time to open shutter")
        n340 = event-data() -> ()  [unwired: 1 in, 1 out]
        n341 = local read "Night Directory"() -> (w669:string)
        n342 = call-dynamic "Read Channel Manager.lvclass.vi"("error in (no error)"=w723, "SPARC4_AC in"=w722) -> ("error out"=w678:errorcluster, "Channel Manager.lvclass"=w679:refnum<class "Channel Manager.lvclass">, "SPARC4_AC out"=w724:refnum<class "SPARC4_AC.lvclass">)  [unwired: 7 in]
        n343 = call-dynamic "Write Current Camera.vi"("error in (no error)"=w678, "Current Camera"=1, "Channel Manager in"=w679) -> ("error out"=w683:errorcluster, "Channel Manager out"=w682:refnum<class "Channel Manager.lvclass">)  [unwired: 7 in]
        n344 = local read "Camera Setup"() -> (w684:T1)
        n345 = call "Return Current RxTx.vi"("error in (no error)"=w683, "Channel Manager in"=w682) -> ("error out"=w704:errorcluster, "RxTx"=w705:refnum<class "RxTx.lvclass">, "Channel Manager out"=w708:refnum<class "Channel Manager.lvclass">)  [unwired: 7 in]
        n346 = call-dynamic "Read Interface.lvclass.vi"("error in (no error)"=w704, "RxTx in"=w705) -> ("error out"=w711:errorcluster, "Interface.lvclass"=w710:refnum<class "Interface.lvclass">, "RxTx out"=w715:refnum<class "RxTx.lvclass">)  [unwired: 7 in]
        n347 = Bundle By Name(cluster=w684, "Image Name"="Image Name 2", "Image Path"=w669, "# Images"="# Images 2", "Number of exp"="# Images 2", "Exposure Time"="Exposure Time 4", "Pre-amp gain"="Pre-amp gain 2", "Readout Rate"="Readout Rate 2", "Vertical Shift Speed"=w676, "Acquisition Mode"=w674, "Trigger"=w675, "Read Mode"=w673, "EM Mode"="EM Mode 2", "EM Gain"="EM Gain 2", "Shutter Mode"=w672, "Shutter TTL"=w671, "Time to open shutter"=w670, "Time to close shutter"=w670, "Vertical Binning"="Binning 6", "Horizontal Binning"="Binning 6", "Initial Line"="Initial Line 2", "Initial Cloumn"="Initial Cloumn 2", "Final Line"="Final Line 2", "Final Column"="Final Column 2", "Exposições realizadas"=u8 0) -> (w714:T1)
        n348 = call-dynamic "Write Exposições realizadas.vi"("error in (no error)"=w711, "Exposições realizadas"=0, "Interface in"=w710) -> ("error out"=w713:errorcluster, "Interface out"=w712:refnum<class "Interface.lvclass">)  [unwired: 7 in]
        n349 = call "Write Camera Setup.vi"("error in (no error)"=w713, "Camera Setup"=w714, "Interface in"=w712) -> ("error out"=w717:errorcluster, "Interface out"=w716:refnum<class "Interface.lvclass">)  [unwired: 7 in]
        n350 = call-dynamic "Write Interface.lvclass.vi"("error in (no error)"=w717, "Interface.lvclass"=w716, "RxTx in"=w715) -> ("error out"=w706:errorcluster, "RxTx out"=w707:refnum<class "RxTx.lvclass">)  [unwired: 7 in]
        n351 = call "Write Current RxTx.vi"("error in (no error)"=w706, "RxTx"=w707, "Channel Manager in"=w708) -> ("error out"=w702:errorcluster, "Channel Manager out"=w703:refnum<class "Channel Manager.lvclass">)  [unwired: 7 in]
        n352 = call "Read Current State Machine.vi"("error in (no error)"=w702, "Channel Manager in"=w703) -> ("error out"=w700:errorcluster, "State Machine.lvclass"=w701:refnum<class "State Machine.lvclass">, "Channel Manager out"=w697:refnum<class "Channel Manager.lvclass">)  [unwired: 7 in]
        n353 = call "Next State.vi"("error in (no error)"=w700, "New_State"=u32 2, "State Machine in"=w701) -> ("error out"=w699:errorcluster, "State Machine out"=w698:refnum<class "State Machine.lvclass">)  [unwired: 7 in]
        n354 = call "Write Current State Machine.vi"("error in (no error)"=w699, "State Machine.lvclass"=w698, "Channel Manager in"=w697) -> ("error out"=w719:errorcluster, "Channel Manager out"=w681:refnum<class "Channel Manager.lvclass">)  [unwired: 7 in]
        n355 = call-dynamic "Write Channel Manager.lvclass.vi"("error in (no error)"=w719, "Channel Manager.lvclass"=w681, "SPARC4_AC in"=w724) -> ("error out"=w720:errorcluster, "SPARC4_AC out"=w721:refnum<class "SPARC4_AC.lvclass">)  [unwired: 7 in]
      }
      event "Stop Acq 2": Value Change {
        n356 = event-data() -> ()  [unwired: 1 in, 1 out]
        n357 = call-dynamic "Read Channel Manager.lvclass.vi"("error in (no error)"=w746, "SPARC4_AC in"=w745) -> ("error out"=w726:errorcluster, "Channel Manager.lvclass"=w727:refnum<class "Channel Manager.lvclass">, "SPARC4_AC out"=w747:refnum<class "SPARC4_AC.lvclass">)  [unwired: 7 in]
        n358 = call-dynamic "Write Current Camera.vi"("error in (no error)"=w726, "Current Camera"=1, "Channel Manager in"=w727) -> ("error out"=w729:errorcluster, "Channel Manager out"=w728:refnum<class "Channel Manager.lvclass">)  [unwired: 7 in]
        n359 = call "Return Current RxTx.vi"("error in (no error)"=w729, "Channel Manager in"=w728) -> ("error out"=w738:errorcluster, "RxTx"=w737:refnum<class "RxTx.lvclass">, "Channel Manager out"=w731:refnum<class "Channel Manager.lvclass">)  [unwired: 7 in]
        n360 = call-dynamic "Read Interface.lvclass.vi"("error in (no error)"=w738, "RxTx in"=w737) -> ("error out"=w733:errorcluster, "Interface.lvclass"=w732:refnum<class "Interface.lvclass">, "RxTx out"=w736:refnum<class "RxTx.lvclass">)  [unwired: 7 in]
        n361 = call-dynamic "Write Stop Acq.vi"("error in (no error)"=w733, "Stop Acq"="Stop Acq 2", "Interface in"=w732) -> ("error out"=w734:errorcluster, "Interface out"=w735:refnum<class "Interface.lvclass">)  [unwired: 7 in]
        n362 = call-dynamic "Write Interface.lvclass.vi"("error in (no error)"=w734, "Interface.lvclass"=w735, "RxTx in"=w736) -> ("error out"=w740:errorcluster, "RxTx out"=w739:refnum<class "RxTx.lvclass">)  [unwired: 7 in]
        n363 = call "Write Current RxTx.vi"("error in (no error)"=w740, "RxTx"=w739, "Channel Manager in"=w731) -> ("error out"=w742:errorcluster, "Channel Manager out"=w730:refnum<class "Channel Manager.lvclass">)  [unwired: 7 in]
        n364 = call-dynamic "Write Channel Manager.lvclass.vi"("error in (no error)"=w742, "Channel Manager.lvclass"=w730, "SPARC4_AC in"=w747) -> ("error out"=w743:errorcluster, "SPARC4_AC out"=w744:refnum<class "SPARC4_AC.lvclass">)  [unwired: 7 in]
      }
      event "Pausar 2": Value Change {
        n365 = event-data() -> ()  [unwired: 1 in, 1 out]
        n366 = call-dynamic "Read Channel Manager.lvclass.vi"("error in (no error)"=w769, "SPARC4_AC in"=w768) -> ("error out"=w751:errorcluster, "Channel Manager.lvclass"=w749:refnum<class "Channel Manager.lvclass">, "SPARC4_AC out"=w770:refnum<class "SPARC4_AC.lvclass">)  [unwired: 7 in]
        n367 = call-dynamic "Write Current Camera.vi"("error in (no error)"=w751, "Current Camera"=1, "Channel Manager in"=w749) -> ("error out"=w753:errorcluster, "Channel Manager out"=w752:refnum<class "Channel Manager.lvclass">)  [unwired: 7 in]
        n368 = call "Return Current RxTx.vi"("error in (no error)"=w753, "Channel Manager in"=w752) -> ("error out"=w756:errorcluster, "RxTx"=w755:refnum<class "RxTx.lvclass">, "Channel Manager out"=w759:refnum<class "Channel Manager.lvclass">)  [unwired: 7 in]
        n369 = call-dynamic "Read Interface.lvclass.vi"("error in (no error)"=w756, "RxTx in"=w755) -> ("error out"=w763:errorcluster, "Interface.lvclass"=w760:refnum<class "Interface.lvclass">, "RxTx out"=w754:refnum<class "RxTx.lvclass">)  [unwired: 7 in]
        n370 = call-dynamic "Write Pause Acq.vi"("error in (no error)"=w763, "Pause Acq"="Pausar 2", "Interface in"=w760) -> ("error out"=w762:errorcluster, "Interface out"=w761:refnum<class "Interface.lvclass">)  [unwired: 7 in]
        n371 = call-dynamic "Write Interface.lvclass.vi"("error in (no error)"=w762, "Interface.lvclass"=w761, "RxTx in"=w754) -> ("error out"=w758:errorcluster, "RxTx out"=w757:refnum<class "RxTx.lvclass">)  [unwired: 7 in]
        n372 = call "Write Current RxTx.vi"("error in (no error)"=w758, "RxTx"=w757, "Channel Manager in"=w759) -> ("error out"=w765:errorcluster, "Channel Manager out"=w750:refnum<class "Channel Manager.lvclass">)  [unwired: 7 in]
        n373 = call-dynamic "Write Channel Manager.lvclass.vi"("error in (no error)"=w765, "Channel Manager.lvclass"=w750, "SPARC4_AC in"=w770) -> ("error out"=w766:errorcluster, "SPARC4_AC out"=w767:refnum<class "SPARC4_AC.lvclass">)  [unwired: 7 in]
      }
      event "Abort 2": Value Change {
        n374 = event-data() -> ()  [unwired: 1 in, 1 out]
        n375 = call-dynamic "Read Channel Manager.lvclass.vi"("error in (no error)"=w791, "SPARC4_AC in"=w792) -> ("error out"=w774:errorcluster, "Channel Manager.lvclass"=w773:refnum<class "Channel Manager.lvclass">, "SPARC4_AC out"=w793:refnum<class "SPARC4_AC.lvclass">)  [unwired: 7 in]
        n376 = call-dynamic "Write Current Camera.vi"("error in (no error)"=w774, "Current Camera"=1, "Channel Manager in"=w773) -> ("error out"=w776:errorcluster, "Channel Manager out"=w775:refnum<class "Channel Manager.lvclass">)  [unwired: 7 in]
        n377 = call "Return Current RxTx.vi"("error in (no error)"=w776, "Channel Manager in"=w775) -> ("error out"=w779:errorcluster, "RxTx"=w778:refnum<class "RxTx.lvclass">, "Channel Manager out"=w782:refnum<class "Channel Manager.lvclass">)  [unwired: 7 in]
        n378 = call-dynamic "Read Interface.lvclass.vi"("error in (no error)"=w779, "RxTx in"=w778) -> ("error out"=w785:errorcluster, "Interface.lvclass"=w784:refnum<class "Interface.lvclass">, "RxTx out"=w777:refnum<class "RxTx.lvclass">)  [unwired: 7 in]
        n379 = call-dynamic "Write Abort.vi"("error in (no error)"=w785, "Abort"="Abort 2", "Interface in"=w784) -> ("error out"=w786:errorcluster, "Interface out"=w783:refnum<class "Interface.lvclass">)  [unwired: 7 in]
        n380 = call-dynamic "Write Interface.lvclass.vi"("error in (no error)"=w786, "Interface.lvclass"=w783, "RxTx in"=w777) -> ("error out"=w781:errorcluster, "RxTx out"=w780:refnum<class "RxTx.lvclass">)  [unwired: 7 in]
        n381 = call "Write Current RxTx.vi"("error in (no error)"=w781, "RxTx"=w780, "Channel Manager in"=w782) -> ("error out"=w788:errorcluster, "Channel Manager out"=w772:refnum<class "Channel Manager.lvclass">)  [unwired: 7 in]
        n382 = call-dynamic "Write Channel Manager.lvclass.vi"("error in (no error)"=w788, "Channel Manager.lvclass"=w772, "SPARC4_AC in"=w793) -> ("error out"=w789:errorcluster, "SPARC4_AC out"=w790:refnum<class "SPARC4_AC.lvclass">)  [unwired: 7 in]
      }
      event "Cooler ON/OFF 2": Value Change {
        n383 = event-data() -> ()  [unwired: 1 in, 1 out]
        n384 = call-dynamic "Read Channel Manager.lvclass.vi"("error in (no error)"=w822, "SPARC4_AC in"=w821) -> ("error out"=w796:errorcluster, "Channel Manager.lvclass"=w797:refnum<class "Channel Manager.lvclass">, "SPARC4_AC out"=w823:refnum<class "SPARC4_AC.lvclass">)  [unwired: 7 in]
        n385 = call-dynamic "Write Current Camera.vi"("error in (no error)"=w796, "Current Camera"=1, "Channel Manager in"=w797) -> ("error out"=w799:errorcluster, "Channel Manager out"=w798:refnum<class "Channel Manager.lvclass">)  [unwired: 7 in]
        n386 = local read "Camera Setup"() -> (w800:T1)
        n387 = Bundle By Name(cluster=w800, "Cooler ON/OFF"="Cooler ON/OFF 2") -> (w816:T1)
        n388 = case shown="0, Default" "Cooler ON/OFF 2" {
          tunnel: ["TURN COOLER OFF" "TURN COOLER ON"] -> w810
          frame 0, Default {
          }
          frame 1 {
          }
        }
        n389 = call "Return Current RxTx.vi"("error in (no error)"=w799, "Channel Manager in"=w798) -> ("error out"=w802:errorcluster, "RxTx"=w803:refnum<class "RxTx.lvclass">, "Channel Manager out"=w806:refnum<class "Channel Manager.lvclass">)  [unwired: 7 in]
        n390 = call-dynamic "Read Interface.lvclass.vi"("error in (no error)"=w802, "RxTx in"=w803) -> ("error out"=w815:errorcluster, "Interface.lvclass"=w817:refnum<class "Interface.lvclass">, "RxTx out"=w807:refnum<class "RxTx.lvclass">)  [unwired: 7 in]
        n391 = call "Write Camera Setup.vi"("error in (no error)"=w815, "Camera Setup"=w816, "Interface in"=w817) -> ("error out"=w808:errorcluster, "Interface out"=w809:refnum<class "Interface.lvclass">)  [unwired: 7 in]
        n392 = call "Write Command.vi"("error in (no error)"=w808, "Command"=w810, "Interface in"=w809) -> ("error out"=w812:errorcluster, "Interface out"=w811:refnum<class "Interface.lvclass">)  [unwired: 7 in]
        n393 = call-dynamic "Write Interface.lvclass.vi"("error in (no error)"=w812, "Interface.lvclass"=w811, "RxTx in"=w807) -> ("error out"=w814:errorcluster, "RxTx out"=w813:refnum<class "RxTx.lvclass">)  [unwired: 7 in]
        n394 = call "Enqeue A Message.vi"("error in (no error)"=w814, "RxTx in"=w813) -> ("error out"=w804:errorcluster, "RxTx out"=w805:refnum<class "RxTx.lvclass">)  [unwired: 8 in]
        n395 = call "Write Current RxTx.vi"("error in (no error)"=w804, "RxTx"=w805, "Channel Manager in"=w806) -> ("error out"=w818:errorcluster, "Channel Manager out"=w795:refnum<class "Channel Manager.lvclass">)  [unwired: 7 in]
        n396 = call-dynamic "Write Channel Manager.lvclass.vi"("error in (no error)"=w818, "Channel Manager.lvclass"=w795, "SPARC4_AC in"=w823) -> ("error out"=w819:errorcluster, "SPARC4_AC out"=w820:refnum<class "SPARC4_AC.lvclass">)  [unwired: 7 in]
      }
      event "Set temperature 2": Value Change {
        n397 = event-data() -> ()  [unwired: 1 in, 1 out]
        n398 = call-dynamic "Read Channel Manager.lvclass.vi"("error in (no error)"=w853, "SPARC4_AC in"=w854) -> ("error out"=w827:errorcluster, "Channel Manager.lvclass"=w826:refnum<class "Channel Manager.lvclass">, "SPARC4_AC out"=w855:refnum<class "SPARC4_AC.lvclass">)  [unwired: 7 in]
        n399 = call-dynamic "Write Current Camera.vi"("error in (no error)"=w827, "Current Camera"=1, "Channel Manager in"=w826) -> ("error out"=w831:errorcluster, "Channel Manager out"=w830:refnum<class "Channel Manager.lvclass">)  [unwired: 7 in]
        n400 = call "Return Current RxTx.vi"("error in (no error)"=w831, "Channel Manager in"=w830) -> ("error out"=w835:errorcluster, "RxTx"=w838:refnum<class "RxTx.lvclass">, "Channel Manager out"=w839:refnum<class "Channel Manager.lvclass">)  [unwired: 7 in]
        n401 = call-dynamic "Read Interface.lvclass.vi"("error in (no error)"=w835, "RxTx in"=w838) -> ("error out"=w843:errorcluster, "Interface.lvclass"=w842:refnum<class "Interface.lvclass">, "RxTx out"=w849:refnum<class "RxTx.lvclass">)  [unwired: 7 in]
        n402 = local read "Camera Setup"() -> (w832:T1)
        n403 = Bundle By Name(cluster=w832, "Set temperature"="Set temperature 2") -> (w833:T1)
        n404 = call "Write Camera Setup.vi"("error in (no error)"=w843, "Camera Setup"=w833, "Interface in"=w842) -> ("error out"=w841:errorcluster, "Interface out"=w840:refnum<class "Interface.lvclass">)  [unwired: 7 in]
        n405 = call "Write Command.vi"("error in (no error)"=w841, "Command"="SET TEMPERATURE", "Interface in"=w840) -> ("error out"=w847:errorcluster, "Interface out"=w848:refnum<class "Interface.lvclass">)  [unwired: 7 in]
        n406 = call-dynamic "Write Interface.lvclass.vi"("error in (no error)"=w847, "Interface.lvclass"=w848, "RxTx in"=w849) -> ("error out"=w845:errorcluster, "RxTx out"=w846:refnum<class "RxTx.lvclass">)  [unwired: 7 in]
        n407 = call "Enqeue A Message.vi"("error in (no error)"=w845, "RxTx in"=w846) -> ("error out"=w836:errorcluster, "RxTx out"=w837:refnum<class "RxTx.lvclass">)  [unwired: 8 in]
        n408 = call "Write Current RxTx.vi"("error in (no error)"=w836, "RxTx"=w837, "Channel Manager in"=w839) -> ("error out"=w850:errorcluster, "Channel Manager out"=w829:refnum<class "Channel Manager.lvclass">)  [unwired: 7 in]
        n409 = call-dynamic "Write Channel Manager.lvclass.vi"("error in (no error)"=w850, "Channel Manager.lvclass"=w829, "SPARC4_AC in"=w855) -> ("error out"=w851:errorcluster, "SPARC4_AC out"=w852:refnum<class "SPARC4_AC.lvclass">)  [unwired: 7 in]
        "Temperature ºC 2" <- "Set temperature 2"
      }
      event "Exposure Time 3": Value Change {
        n410 = event-data() -> ()  [unwired: 1 in, 1 out]
        n411 = local write "Exposure Time 4"("Exposure Time 3") -> ()
      }
      event "# Images 2": Value Change {
        n412 = event-data() -> ()  [unwired: 1 in, 1 out]
        n413 = local read "# Images 2"() -> (w864:u32)
        n414 = property on="Exposições realizadas 2" class="Slide (strict)"("Scale.Maximum"=w864) -> ()  [unwired: 2 in, 2 out]
        n415 = call-dynamic "Read Sync Mode.vi"("error in (no error)"=w861, "SPARC4_AC in"=w862) -> ("error out"=w860:errorcluster, "Sync Mode"=w863:u16, "SPARC4_AC out"=w859:refnum<class "SPARC4_AC.lvclass">)  [unwired: 7 in]
        n416 = case shown="1, Default" w863 {
          frame 0 {
          }
          frame 1, Default {
            n417 = local read "# Images 2"() -> (w865:u32)
            n418 = property on="Exposições realizadas" class="Slide (strict)"("Scale.Maximum"=w865) -> ()  [unwired: 2 in, 2 out]
            n419 = local write "# Ciclos"(w865) -> ()
          }
        }
      }
      event "Exposure Time 4": Value Change {
        n420 = event-data() -> ()  [unwired: 1 in, 1 out]
        n421 = local read "Exposure Time 4"() -> (w868:u32)
        n422 = local write "Exposure Time 3"(w868) -> ()
      }
      event "Sub Image 2": Value Change {
        n423 = event-data() -> ()  [unwired: 1 in, 1 out]
        n424 = call-dynamic "Read Channel Manager.lvclass.vi"("error in (no error)"=w883, "SPARC4_AC in"=w884) -> ("error out"=w871:errorcluster, "Channel Manager.lvclass"=w872:refnum<class "Channel Manager.lvclass">, "SPARC4_AC out"=w889:refnum<class "SPARC4_AC.lvclass">)  [unwired: 7 in]
        n425 = call-dynamic "Write Current Camera.vi"("error in (no error)"=w871, "Current Camera"=1, "Channel Manager in"=w872) -> ("error out"=w874:errorcluster, "Channel Manager out"=w873:refnum<class "Channel Manager.lvclass">)  [unwired: 7 in]
        n426 = call "Return Current RxTx.vi"("error in (no error)"=w874, "Channel Manager in"=w873) -> ("error out"=w901:errorcluster, "RxTx"=w902:refnum<class "RxTx.lvclass">, "Channel Manager out"=w869:refnum<class "Channel Manager.lvclass">)  [unwired: 7 in]
        n427 = call-dynamic "Read Interface.lvclass.vi"("error in (no error)"=w901, "RxTx in"=w902) -> ("error out"=w899:errorcluster, "Interface.lvclass"=w900:refnum<class "Interface.lvclass">)  [unwired: 7 in, 1 out]
        n428 = call "Read Camera Status.vi"("error in (no error)"=w899, "Interface in"=w900) -> ("error out"=w890:errorcluster, "Camera Status"=w898:T6)  [unwired: 7 in, 1 out]
        n429 = Unbundle By Name(w898) -> ("Final Column"=w895:u16, "Final Line"=w894:u16)
        n430 = call-dynamic "Write Channel Manager.lvclass.vi"("error in (no error)"=w890, "Channel Manager.lvclass"=w869, "SPARC4_AC in"=w889) -> ("error out"=w888:errorcluster, "SPARC4_AC out"=w887:refnum<class "SPARC4_AC.lvclass">)  [unwired: 7 in]
        n431 = case shown="\"256 x 256\"" "Sub Image 2" {
          tunnel: [128 256 512 512] -> w893
          frame "256 x 256" {
          }
          frame "512 x 512" {
          }
          frame "1024 x 1024", Default {
          }
          frame "Custom" {
          }
        }
        n432 = case shown="\"1024 x 1024\", Default" "Sub Image 2" {
          tunnel: [T7."Disabled and Grayed Out" ("Disabled") T7."Enabled" ("Disabled")] -> w879
          frame "1024 x 1024", Default {
          }
          frame "Custom" {
          }
        }
        n433 = Divide(x=w895, y=2) -> (x/y=w896:dbl)
        n434 = Divide(x=w894, y=2) -> (x/y=w897:dbl)
        n435 = Add(x=w896, y=w893) -> (x+y=w878:dbl)
        n436 = Subtract(x=w896, y=w893) -> (x-y=w892:dbl)
        n437 = Subtract(x=w897, y=w893) -> (x-y=w891:dbl)
        n438 = Add(x=w897, y=w893) -> (x+y=w875:dbl)
        n439 = Increment(x=w892) -> (x+1=w877:dbl)
        n440 = Increment(x=w891) -> (x+1=w876:dbl)
        n441 = local write "Initial Line 2"(w878) -> ()
        n442 = local write "Initial Cloumn 2"(w877) -> ()
        n443 = local write "Final Line 2"(w876) -> ()
        n444 = local write "Final Column 2"(w875) -> ()
        n445 = property on="Initial Line 2" class="DigNum (strict)"("DisabledEnum"=w879) -> ()  [unwired: 2 in, 2 out]
        n446 = property on="Initial Cloumn 2" class="DigNum (strict)"("DisabledEnum"=w879) -> ()  [unwired: 2 in, 2 out]
        n447 = property on="Final Line 2" class="DigNum (strict)"("DisabledEnum"=w879) -> ()  [unwired: 2 in, 2 out]
        n448 = property on="Final Column 2" class="DigNum (strict)"("DisabledEnum"=w879) -> ()  [unwired: 2 in, 2 out]
        n449 = flat-sequence {
          tunnel: w888 -> [w913]
          tunnel: w887 -> [w914]
          tunnel: [w914] -> w882
          tunnel: [w913] -> w881
          frame #0 {
            w907 = cluster{dbl, dbl} {0.0, 0.0}
            n450 = local read "Initial Cloumn 2"() -> (w906:u16)
            n451 = local read "Final Column 2"() -> (w904:u16)
            n452 = local read "Initial Line 2"() -> (w905:u16)
            n453 = local read "Final Line 2"() -> (w903:u16)
            n454 = Bundle(cluster=w907, w906, w905) -> (w912:cluster{dbl, dbl})
            n455 = Bundle(cluster=w907, w906, w903) -> (w911:cluster{dbl, dbl})
            n456 = Bundle(cluster=w907, w904, w903) -> (w910:cluster{dbl, dbl})
            n457 = Bundle(cluster=w907, w904, w905) -> (w909:cluster{dbl, dbl})
            n458 = Bundle(cluster=w907, w906, w905) -> (w908:cluster{dbl, dbl})
            n459 = Build Array(w912, w911, w910, w909, w908) -> ()  [unwired: 1 out]
          }
        }
      }
      event "Initial Line 2", "Initial Cloumn 2", "Final Line 2", "Final Column 2": Value Change {
        n460 = event-data() -> ()  [unwired: 1 in, 1 out]
        n461 = disable-structure shown="Disabled" {
          frame Disabled {
            w927 = cluster{dbl, dbl} {0.0, 0.0}
            n462 = local read "Initial Cloumn 2"() -> (w926:u16)
            n463 = local read "Final Column 2"() -> (w924:u16)
            n464 = local read "Initial Line 2"() -> (w925:u16)
            n465 = local read "Final Line 2"() -> (w923:u16)
            n466 = Bundle(cluster=w927, w926, w925) -> (w932:cluster{dbl, dbl})
            n467 = Bundle(cluster=w927, w926, w923) -> (w931:cluster{dbl, dbl})
            n468 = Bundle(cluster=w927, w924, w923) -> (w930:cluster{dbl, dbl})
            n469 = Bundle(cluster=w927, w924, w925) -> (w929:cluster{dbl, dbl})
            n470 = Bundle(cluster=w927, w926, w925) -> (w928:cluster{dbl, dbl})
            n471 = Build Array(w932, w931, w930, w929, w928) -> ()  [unwired: 1 out]
          }
          frame Enabled {
          }
        }
      }
      event "Adquirir 3": Value Change {
        n472 = event-data() -> ()  [unwired: 1 in, 1 out]
        n473 = call-dynamic "Read Channel Manager.lvclass.vi"("error in (no error)"=w944, "SPARC4_AC in"=w943) -> ("error out"=w935:errorcluster, "Channel Manager.lvclass"=w934:refnum<class "Channel Manager.lvclass">, "SPARC4_AC out"=w942:refnum<class "SPARC4_AC.lvclass">)  [unwired: 7 in]
        n474 = call-dynamic "Read Available Cameras.vi"("error in (no error)"=w935, "Channel Manager in"=w934) -> ("error out"=w936:errorcluster, "Available Cameras"=w938:u8, "Channel Manager out"=w937:refnum<class "Channel Manager.lvclass">)  [unwired: 7 in]
        n475 = for {
          N: w938 -> [_]
          tunnel: [w946] -> w939
          tunnel: w936 -> [w945]
          shift-right: [w947] -> w933
          shift-left: w937 -> [w948]
          i -> [w949]
          n476 = case shown="0, Default" w949 {
            tunnel: [w964 w1015 w1065 w1116] -> w947
            tunnel: [w963 w1014 w1066 w1117] -> w946
            tunnel: w948 -> [w962 w1013 w1064 w1115]
            tunnel: w945 -> [w959 w1010 w1061 w1112]
            frame 0, Default {
              w955 = u8 4 items=["Full Vertical Binning", "Multi-Track", "Random-track", "Single-Track", "Image"] ("Read Mode")
              w958 = u8 3 items=["0.6", "1.13", "2.2", "4.33"] ("Vertical Shift \nSpeed")
              w957 = u8 3 items=["N/A", "Single", "Accumulate", "Kinetic", "Fast Kinetic"] ("Acquisition Mode")
              w956 = u8 6 items=["Internal", "External", "RESERVED", "RESERVED", "RESERVED", "RESERVED", "External Start"] ("Trigger")
              w954 = u8 2 items=["Fully Auto", "OPEN", "CLOSED"] ("Shutter Mode")
              w953 = u8 0 items=["TTL Low", "TTl High"] ("Shutter TTL")
              w952 = u16 50 ("Time to open shutter")
              n477 = local read "Image Name"() -> (w991:string)
              n478 = local read "Exposure Time 2"() -> (w994:dbl)
              n479 = local read "Pre-amp gain"() -> (w997:u8)
              n480 = local read "Readout Rate"() -> (w998:u8)
              n481 = local read "EM Mode"() -> (w996:u8)
              n482 = local read "EM Gain"() -> (w999:u16)
              n483 = local read "Initial Line"() -> (w995:u16)
              n484 = local read "Initial Cloumn"() -> (w993:u16)
              n485 = local read "Final Line"() -> (w990:u16)
              n486 = local read "Final Column"() -> (w992:u16)
              n487 = local read "# Ciclos"() -> (w1000:u32)
              n488 = local read "Night Directory"() -> (w950:string)
              n489 = local read "Binning 5"() -> (w951:u8)
              n490 = call-dynamic "Write Current Camera.vi"("error in (no error)"=w959, "Current Camera"=0, "Channel Manager in"=w962) -> ("error out"=w976:errorcluster, "Channel Manager out"=w977:refnum<class "Channel Manager.lvclass">)  [unwired: 7 in]
              n491 = call "Return Current RxTx.vi"("error in (no error)"=w976, "Channel Manager in"=w977) -> ("error out"=w982:errorcluster, "RxTx"=w981:refnum<class "RxTx.lvclass">, "Channel Manager out"=w978:refnum<class "Channel Manager.lvclass">)  [unwired: 7 in]
              n492 = call-dynamic "Read Interface.lvclass.vi"("error in (no error)"=w982, "RxTx in"=w981) -> ("error out"=w974:errorcluster, "Interface.lvclass"=w975:refnum<class "Interface.lvclass">, "RxTx out"=w970:refnum<class "RxTx.lvclass">)  [unwired: 7 in]
              n493 = local read "Camera Setup"() -> (w960:T1)
              n494 = Bundle By Name(cluster=w960, "Image Name"=w991, "Image Path"=w950, "# Images"=w1000, "Exposure Time"=w994, "Pre-amp gain"=w997, "Readout Rate"=w998, "Vertical Shift Speed"=w958, "Acquisition Mode"=w957, "Trigger"=w956, "Read Mode"=w955, "EM Mode"=w996, "EM Gain"=w999, "Shutter Mode"=w954, "Shutter TTL"=w953, "Time to open shutter"=w952, "Time to close shutter"=w952, "Vertical Binning"=w951, "Horizontal Binning"=w951, "Initial Line"=w995, "Initial Cloumn"=w993, "Final Line"=w990, "Final Column"=w992, "Exposições realizadas"=u8 0) -> (w971:T1)
              n495 = call-dynamic "Write Exposições realizadas.vi"("error in (no error)"=w974, "Exposições realizadas"=0, "Interface in"=w975) -> ("error out"=w972:errorcluster, "Interface out"=w973:refnum<class "Interface.lvclass">)  [unwired: 7 in]
              n496 = call "Write Camera Setup.vi"("error in (no error)"=w972, "Camera Setup"=w971, "Interface in"=w973) -> ("error out"=w968:errorcluster, "Interface out"=w969:refnum<class "Interface.lvclass">)  [unwired: 7 in]
              n497 = call-dynamic "Write Interface.lvclass.vi"("error in (no error)"=w968, "Interface.lvclass"=w969, "RxTx in"=w970) -> ("error out"=w980:errorcluster, "RxTx out"=w979:refnum<class "RxTx.lvclass">)  [unwired: 7 in]
              n498 = call "Write Current RxTx.vi"("error in (no error)"=w980, "RxTx"=w979, "Channel Manager in"=w978) -> ("error out"=w984:errorcluster, "Channel Manager out"=w983:refnum<class "Channel Manager.lvclass">)  [unwired: 7 in]
              n499 = call "Read Current State Machine.vi"("error in (no error)"=w984, "Channel Manager in"=w983) -> ("error out"=w986:errorcluster, "State Machine.lvclass"=w985:refnum<class "State Machine.lvclass">, "Channel Manager out"=w989:refnum<class "Channel Manager.lvclass">)  [unwired: 7 in]
              n500 = call "Next State.vi"("error in (no error)"=w986, "New_State"=u32 2, "State Machine in"=w985) -> ("error out"=w987:errorcluster, "State Machine out"=w988:refnum<class "State Machine.lvclass">)  [unwired: 7 in]
              n501 = call "Write Current State Machine.vi"("error in (no error)"=w987, "State Machine.lvclass"=w988, "Channel Manager in"=w989) -> ("error out"=w963:errorcluster, "Channel Manager out"=w964:refnum<class "Channel Manager.lvclass">)  [unwired: 7 in]
            }
            frame 1 {
              w1006 = u8 4 items=["Full Vertical Binning", "Multi-Track", "Random-track", "Single-Track", "Image"] ("Read Mode")
              w1009 = u8 3 items=["0.6", "1.13", "2.2", "4.33"] ("Vertical Shift \nSpeed")
              w1008 = u8 3 items=["N/A", "Single", "Accumulate", "Kinetic", "Fast Kinetic"] ("Acquisition Mode")
              w1007 = u8 6 items=["Internal", "External", "RESERVED", "RESERVED", "RESERVED", "RESERVED", "External Start"] ("Trigger")
              w1005 = u8 2 items=["Fully Auto", "OPEN", "CLOSED"] ("Shutter Mode")
              w1004 = u8 0 items=["TTL Low", "TTl High"] ("Shutter TTL")
              w1003 = u16 50 ("Time to open shutter")
              n502 = local read "EM Mode 2"() -> (w1045:u8)
              n503 = local read "Initial Cloumn 2"() -> (w1048:u16)
              n504 = local read "Final Column 2"() -> (w1050:u16)
              n505 = local read "Image Name 2"() -> (w1041:string)
              n506 = local read "# Images 2"() -> (w1042:u32)
              n507 = local read "Pre-amp gain 2"() -> (w1044:u8)
              n508 = local read "Readout Rate 2"() -> (w1051:u8)
              n509 = local read "EM Gain 2"() -> (w1046:u16)
              n510 = local read "Initial Line 2"() -> (w1047:u16)
              n511 = local read "Final Line 2"() -> (w1049:u16)
              n512 = local read "Night Directory"() -> (w1001:string)
              n513 = local read "Exposure Time 4"() -> (w1043:u32)
              n514 = local read "Binning 6"() -> (w1002:u16)
              n515 = call-dynamic "Write Current Camera.vi"("error in (no error)"=w1010, "Current Camera"=1, "Channel Manager in"=w1013) -> ("error out"=w1026:errorcluster, "Channel Manager out"=w1027:refnum<class "Channel Manager.lvclass">)  [unwired: 7 in]
              n516 = call "Return Current RxTx.vi"("error in (no error)"=w1026, "Channel Manager in"=w1027) -> ("error out"=w1032:errorcluster, "RxTx"=w1031:refnum<class "RxTx.lvclass">, "Channel Manager out"=w1028:refnum<class "Channel Manager.lvclass">)  [unwired: 7 in]
              n517 = call-dynamic "Read Interface.lvclass.vi"("error in (no error)"=w1032, "RxTx in"=w1031) -> ("error out"=w1024:errorcluster, "Interface.lvclass"=w1025:refnum<class "Interface.lvclass">, "RxTx out"=w1021:refnum<class "RxTx.lvclass">)  [unwired: 7 in]
              n518 = local read "Camera Setup"() -> (w1011:T1)
              n519 = Bundle By Name(cluster=w1011, "Image Name"=w1041, "Image Path"=w1001, "# Images"=w1042, "Exposure Time"=w1043, "Pre-amp gain"=w1044, "Readout Rate"=w1051, "Vertical Shift Speed"=w1009, "Acquisition Mode"=w1008, "Trigger"=w1007, "Read Mode"=w1006, "EM Mode"=w1045, "EM Gain"=w1046, "Shutter Mode"=w1005, "Shutter TTL"=w1004, "Time to open shutter"=w1003, "Time to close shutter"=w1003, "Vertical Binning"=w1002, "Horizontal Binning"=w1002, "Initial Line"=w1047, "Initial Cloumn"=w1048, "Final Line"=w1049, "Final Column"=w1050, "Exposições realizadas"=u8 0) -> (w1040:T1)
              n520 = call-dynamic "Write Exposições realizadas.vi"("error in (no error)"=w1024, "Exposições realizadas"=0, "Interface in"=w1025) -> ("error out"=w1022:errorcluster, "Interface out"=w1023:refnum<class "Interface.lvclass">)  [unwired: 7 in]
              n521 = call "Write Camera Setup.vi"("error in (no error)"=w1022, "Camera Setup"=w1040, "Interface in"=w1023) -> ("error out"=w1019:errorcluster, "Interface out"=w1020:refnum<class "Interface.lvclass">)  [unwired: 7 in]
              n522 = call-dynamic "Write Interface.lvclass.vi"("error in (no error)"=w1019, "Interface.lvclass"=w1020, "RxTx in"=w1021) -> ("error out"=w1030:errorcluster, "RxTx out"=w1029:refnum<class "RxTx.lvclass">)  [unwired: 7 in]
              n523 = call "Write Current RxTx.vi"("error in (no error)"=w1030, "RxTx"=w1029, "Channel Manager in"=w1028) -> ("error out"=w1034:errorcluster, "Channel Manager out"=w1033:refnum<class "Channel Manager.lvclass">)  [unwired: 7 in]
              n524 = call "Read Current State Machine.vi"("error in (no error)"=w1034, "Channel Manager in"=w1033) -> ("error out"=w1036:errorcluster, "State Machine.lvclass"=w1035:refnum<class "State Machine.lvclass">, "Channel Manager out"=w1039:refnum<class "Channel Manager.lvclass">)  [unwired: 7 in]
              n525 = call "Next State.vi"("error in (no error)"=w1036, "New_State"=u32 2, "State Machine in"=w1035) -> ("error out"=w1037:errorcluster, "State Machine out"=w1038:refnum<class "State Machine.lvclass">)  [unwired: 7 in]
              n526 = call "Write Current State Machine.vi"("error in (no error)"=w1037, "State Machine.lvclass"=w1038, "Channel Manager in"=w1039) -> ("error out"=w1014:errorcluster, "Channel Manager out"=w1015:refnum<class "Channel Manager.lvclass">)  [unwired: 7 in]
            }
            frame 2 {
              w1057 = u8 4 items=["Full Vertical Binning", "Multi-Track", "Random-track", "Single-Track", "Image"] ("Read Mode")
              w1060 = u8 3 items=["0.6", "1.13", "2.2", "4.33"] ("Vertical Shift \nSpeed")
              w1059 = u8 3 items=["N/A", "Single", "Accumulate", "Kinetic", "Fast Kinetic"] ("Acquisition Mode")
              w1058 = u8 6 items=["Internal", "External", "RESERVED", "RESERVED", "RESERVED", "RESERVED", "External Start"] ("Trigger")
              w1056 = u8 2 items=["Fully Auto", "OPEN", "CLOSED"] ("Shutter Mode")
              w1055 = u8 0 items=["TTL Low", "TTl High"] ("Shutter TTL")
              w1054 = u16 50 ("Time to open shutter")
              n527 = local read "EM Mode 3"() -> (w1096:u8)
              n528 = local read "Initial Cloumn 3"() -> (w1099:u16)
              n529 = local read "Final Column 3"() -> (w1101:u16)
              n530 = local read "Image Name 3"() -> (w1092:string)
              n531 = local read "# Images 3"() -> (w1093:u32)
              n532 = local read "Pre-amp gain 3"() -> (w1095:u8)
              n533 = local read "Readout Rate 3"() -> (w1102:u8)
              n534 = local read "EM Gain 3"() -> (w1097:u16)
              n535 = local read "Initial Line 3"() -> (w1098:u16)
              n536 = local read "Final Line 3"() -> (w1100:u16)
              n537 = local read "Exposure Time 7"() -> (w1094:dbl)
              n538 = local read "Night Directory"() -> (w1052:string)
              n539 = local read "Binning 7"() -> (w1053:u16)
              n540 = call-dynamic "Write Current Camera.vi"("error in (no error)"=w1061, "Current Camera"=2, "Channel Manager in"=w1064) -> ("error out"=w1077:errorcluster, "Channel Manager out"=w1078:refnum<class "Channel Manager.lvclass">)  [unwired: 7 in]
              n541 = call "Return Current RxTx.vi"("error in (no error)"=w1077, "Channel Manager in"=w1078) -> ("error out"=w1083:errorcluster, "RxTx"=w1082:refnum<class "RxTx.lvclass">, "Channel Manager out"=w1079:refnum<class "Channel Manager.lvclass">)  [unwired: 7 in]
              n542 = call-dynamic "Read Interface.lvclass.vi"("error in (no error)"=w1083, "RxTx in"=w1082) -> ("error out"=w1075:errorcluster, "Interface.lvclass"=w1076:refnum<class "Interface.lvclass">, "RxTx out"=w1072:refnum<class "RxTx.lvclass">)  [unwired: 7 in]
              n543 = local read "Camera Setup"() -> (w1062:T1)
              n544 = Bundle By Name(cluster=w1062, "Image Name"=w1092, "Image Path"=w1052, "# Images"=w1093, "Exposure Time"=w1094, "Pre-amp gain"=w1095, "Readout Rate"=w1102, "Vertical Shift Speed"=w1060, "Acquisition Mode"=w1059, "Trigger"=w1058, "Read Mode"=w1057, "EM Mode"=w1096, "EM Gain"=w1097, "Shutter Mode"=w1056, "Shutter TTL"=w1055, "Time to open shutter"=w1054, "Time to close shutter"=w1054, "Vertical Binning"=w1053, "Horizontal Binning"=w1053, "Initial Line"=w1098, "Initial Cloumn"=w1099, "Final Line"=w1100, "Final Column"=w1101, "Exposições realizadas"=u8 0) -> (w1091:T1)
              n545 = call-dynamic "Write Exposições realizadas.vi"("error in (no error)"=w1075, "Exposições realizadas"=0, "Interface in"=w1076) -> ("error out"=w1073:errorcluster, "Interface out"=w1074:refnum<class "Interface.lvclass">)  [unwired: 7 in]
              n546 = call "Write Camera Setup.vi"("error in (no error)"=w1073, "Camera Setup"=w1091, "Interface in"=w1074) -> ("error out"=w1070:errorcluster, "Interface out"=w1071:refnum<class "Interface.lvclass">)  [unwired: 7 in]
              n547 = call-dynamic "Write Interface.lvclass.vi"("error in (no error)"=w1070, "Interface.lvclass"=w1071, "RxTx in"=w1072) -> ("error out"=w1081:errorcluster, "RxTx out"=w1080:refnum<class "RxTx.lvclass">)  [unwired: 7 in]
              n548 = call "Write Current RxTx.vi"("error in (no error)"=w1081, "RxTx"=w1080, "Channel Manager in"=w1079) -> ("error out"=w1085:errorcluster, "Channel Manager out"=w1084:refnum<class "Channel Manager.lvclass">)  [unwired: 7 in]
              n549 = call "Read Current State Machine.vi"("error in (no error)"=w1085, "Channel Manager in"=w1084) -> ("error out"=w1087:errorcluster, "State Machine.lvclass"=w1086:refnum<class "State Machine.lvclass">, "Channel Manager out"=w1090:refnum<class "Channel Manager.lvclass">)  [unwired: 7 in]
              n550 = call "Next State.vi"("error in (no error)"=w1087, "New_State"=u32 2, "State Machine in"=w1086) -> ("error out"=w1088:errorcluster, "State Machine out"=w1089:refnum<class "State Machine.lvclass">)  [unwired: 7 in]
              n551 = call "Write Current State Machine.vi"("error in (no error)"=w1088, "State Machine.lvclass"=w1089, "Channel Manager in"=w1090) -> ("error out"=w1066:errorcluster, "Channel Manager out"=w1065:refnum<class "Channel Manager.lvclass">)  [unwired: 7 in]
            }
            frame 3 {
              w1108 = u8 4 items=["Full Vertical Binning", "Multi-Track", "Random-track", "Single-Track", "Image"] ("Read Mode")
              w1111 = u8 3 items=["0.6", "1.13", "2.2", "4.33"] ("Vertical Shift \nSpeed")
              w1110 = u8 3 items=["N/A", "Single", "Accumulate", "Kinetic", "Fast Kinetic"] ("Acquisition Mode")
              w1109 = u8 6 items=["Internal", "External", "RESERVED", "RESERVED", "RESERVED", "RESERVED", "External Start"] ("Trigger")
              w1107 = u8 2 items=["Fully Auto", "OPEN", "CLOSED"] ("Shutter Mode")
              w1106 = u8 0 items=["TTL Low", "TTl High"] ("Shutter TTL")
              w1105 = u16 50 ("Time to open shutter")
              n552 = local read "EM Mode 4"() -> (w1147:u8)
              n553 = local read "Initial Cloumn 4"() -> (w1150:u16)
              n554 = local read "Final Column 4"() -> (w1152:u16)
              n555 = local read "Image Name 4"() -> (w1143:string)
              n556 = local read "# Images 4"() -> (w1144:u32)
              n557 = local read "Pre-amp gain 4"() -> (w1146:u8)
              n558 = local read "Readout Rate 4"() -> (w1153:u8)
              n559 = local read "EM Gain 4"() -> (w1148:u16)
              n560 = local read "Initial Line 4"() -> (w1149:u16)
              n561 = local read "Final Line 4"() -> (w1151:u16)
              n562 = local read "Exposure Time 8"() -> (w1145:dbl)
              n563 = local read "Night Directory"() -> (w1103:string)
              n564 = local read "Binning 8"() -> (w1104:u16)
              n565 = call-dynamic "Write Current Camera.vi"("error in (no error)"=w1112, "Current Camera"=3, "Channel Manager in"=w1115) -> ("error out"=w1128:errorcluster, "Channel Manager out"=w1129:refnum<class "Channel Manager.lvclass">)  [unwired: 7 in]
              n566 = call "Return Current RxTx.vi"("error in (no error)"=w1128, "Channel Manager in"=w1129) -> ("error out"=w1134:errorcluster, "RxTx"=w1133:refnum<class "RxTx.lvclass">, "Channel Manager out"=w1130:refnum<class "Channel Manager.lvclass">)  [unwired: 7 in]
              n567 = call-dynamic "Read Interface.lvclass.vi"("error in (no error)"=w1134, "RxTx in"=w1133) -> ("error out"=w1126:errorcluster, "Interface.lvclass"=w1127:refnum<class "Interface.lvclass">, "RxTx out"=w1123:refnum<class "RxTx.lvclass">)  [unwired: 7 in]
              n568 = local read "Camera Setup"() -> (w1113:T1)
              n569 = Bundle By Name(cluster=w1113, "Image Name"=w1143, "Image Path"=w1103, "# Images"=w1144, "Exposure Time"=w1145, "Pre-amp gain"=w1146, "Readout Rate"=w1153, "Vertical Shift Speed"=w1111, "Acquisition Mode"=w1110, "Trigger"=w1109, "Read Mode"=w1108, "EM Mode"=w1147, "EM Gain"=w1148, "Shutter Mode"=w1107, "Shutter TTL"=w1106, "Time to open shutter"=w1105, "Time to close shutter"=w1105, "Vertical Binning"=w1104, "Horizontal Binning"=w1104, "Initial Line"=w1149, "Initial Cloumn"=w1150, "Final Line"=w1151, "Final Column"=w1152, "Exposições realizadas"=u8 0) -> (w1142:T1)
              n570 = call-dynamic "Write Exposições realizadas.vi"("error in (no error)"=w1126, "Exposições realizadas"=0, "Interface in"=w1127) -> ("error out"=w1124:errorcluster, "Interface out"=w1125:refnum<class "Interface.lvclass">)  [unwired: 7 in]
              n571 = call "Write Camera Setup.vi"("error in (no error)"=w1124, "Camera Setup"=w1142, "Interface in"=w1125) -> ("error out"=w1121:errorcluster, "Interface out"=w1122:refnum<class "Interface.lvclass">)  [unwired: 7 in]
              n572 = call-dynamic "Write Interface.lvclass.vi"("error in (no error)"=w1121, "Interface.lvclass"=w1122, "RxTx in"=w1123) -> ("error out"=w1132:errorcluster, "RxTx out"=w1131:refnum<class "RxTx.lvclass">)  [unwired: 7 in]
              n573 = call "Write Current RxTx.vi"("error in (no error)"=w1132, "RxTx"=w1131, "Channel Manager in"=w1130) -> ("error out"=w1136:errorcluster, "Channel Manager out"=w1135:refnum<class "Channel Manager.lvclass">)  [unwired: 7 in]
              n574 = call "Read Current State Machine.vi"("error in (no error)"=w1136, "Channel Manager in"=w1135) -> ("error out"=w1138:errorcluster, "State Machine.lvclass"=w1137:refnum<class "State Machine.lvclass">, "Channel Manager out"=w1141:refnum<class "Channel Manager.lvclass">)  [unwired: 7 in]
              n575 = call "Next State.vi"("error in (no error)"=w1138, "New_State"=u32 2, "State Machine in"=w1137) -> ("error out"=w1139:errorcluster, "State Machine out"=w1140:refnum<class "State Machine.lvclass">)  [unwired: 7 in]
              n576 = call "Write Current State Machine.vi"("error in (no error)"=w1139, "State Machine.lvclass"=w1140, "Channel Manager in"=w1141) -> ("error out"=w1117:errorcluster, "Channel Manager out"=w1116:refnum<class "Channel Manager.lvclass">)  [unwired: 7 in]
            }
          }
        }
        n577 = call-dynamic "Write Channel Manager.lvclass.vi"("error in (no error)"=w939, "Channel Manager.lvclass"=w933, "SPARC4_AC in"=w942) -> ("error out"=w941:errorcluster, "SPARC4_AC out"=w940:refnum<class "SPARC4_AC.lvclass">)  [unwired: 7 in]
      }
      event "Sync Mode": Value Change {
        n578 = event-data() -> ()  [unwired: 1 in, 1 out]
        n579 = case shown="True" "Sync Mode" {
          tunnel: [T7."Enabled" ("Disabled") T7."Disabled and Grayed Out" ("Disabled")] -> w1155
          tunnel: [w1164 w1169] -> w1158
          tunnel: [T7."Disabled and Grayed Out" ("Disabled") T7."Enabled" ("Disabled")] -> w1154
          frame False {
            w1164 = u16 0 items=["Not Synchronized", "Continuous Mode", "Aligned by the edge", "Aligned by the center"] ("Sync Mode")
            n580 = local write "Sync Mode: 2"(T3."Radio Selection 1" ("Sync Mode: 2")) -> ()
          }
          frame True {
            w1166 = u32 1 ("# Images 2")
            w1168 = u32 1 ("# Images 2")
            w1169 = u16 1 items=["Not Synchronized", "Continuous Mode", "Aligned by the edge", "Aligned by the center"] ("Sync Mode")
            n581 = property on="Exposições realizadas" class="Slide (strict)"("Scale.Maximum"=w1166) -> ()  [unwired: 2 in, 2 out]
            n582 = property on="Exposições realizadas 2" class="Slide (strict)"("Scale.Maximum"=w1166) -> ()  [unwired: 2 in, 2 out]
            n583 = local write "# Images 2"(w1168) -> ()
            n584 = local write "# Ciclos"(w1168) -> ()
          }
        }
        n585 = property on="Adquirir 3" class="Bool"("DisabledEnum"=w1154) -> ()  [unwired: 2 in, 2 out]
        n586 = property on="Stop Acq 3" class="Bool"("DisabledEnum"=w1154) -> ()  [unwired: 2 in, 2 out]
        n587 = property on="Pausar 3" class="Bool (strict)"("DisabledEnum"=w1154) -> ()  [unwired: 2 in, 2 out]
        n588 = property on="Abort 3" class="Bool"("DisabledEnum"=w1154) -> ()  [unwired: 2 in, 2 out]
        n589 = property on="Sync Mode: 2" class="RadioBtnsControl (strict)"("DisabledEnum"=w1154) -> ()  [unwired: 2 in, 2 out]
        n590 = call-dynamic "Write Sync Mode.vi"("error in (no error)"=w1160, "Sync Mode"=w1158, "SPARC4_AC in"=w1161) -> ("error out"=w1156:errorcluster, "SPARC4_AC out"=w1157:refnum<class "SPARC4_AC.lvclass">)  [unwired: 7 in]
        n591 = property on="Adquirir" class="Bool"("DisabledEnum"=w1155) -> ()  [unwired: 2 in, 2 out]
        n592 = property on="Stop Acq" class="Bool"("DisabledEnum"=w1155) -> ()  [unwired: 2 in, 2 out]
        n593 = property on="Pausar" class="Bool (strict)"("DisabledEnum"=w1155) -> ()  [unwired: 2 in, 2 out]
        n594 = property on="Abort" class="Bool"("DisabledEnum"=w1155) -> ()  [unwired: 2 in, 2 out]
        n595 = property on="Adquirir 2" class="Bool"("DisabledEnum"=w1155) -> ()  [unwired: 2 in, 2 out]
        n596 = property on="Stop Acq 2" class="Bool"("DisabledEnum"=w1155) -> ()  [unwired: 2 in, 2 out]
        n597 = property on="Pausar 2" class="Bool (strict)"("DisabledEnum"=w1155) -> ()  [unwired: 2 in, 2 out]
        n598 = property on="Abort 2" class="Bool"("DisabledEnum"=w1155) -> ()  [unwired: 2 in, 2 out]
        n599 = property on="Adquirir 4" class="Bool"("DisabledEnum"=w1155) -> ()  [unwired: 2 in, 2 out]
        n600 = property on="Stop Acq 4" class="Bool"("DisabledEnum"=w1155) -> ()  [unwired: 2 in, 2 out]
        n601 = property on="Pausar 4" class="Bool (strict)"("DisabledEnum"=w1155) -> ()  [unwired: 2 in, 2 out]
        n602 = property on="Abort 4" class="Bool"("DisabledEnum"=w1155) -> ()  [unwired: 2 in, 2 out]
        n603 = property on="Adquirir 5" class="Bool"("DisabledEnum"=w1155) -> ()  [unwired: 2 in, 2 out]
        n604 = property on="Stop Acq 5" class="Bool"("DisabledEnum"=w1155) -> ()  [unwired: 2 in, 2 out]
        n605 = property on="Pausar 5" class="Bool (strict)"("DisabledEnum"=w1155) -> ()  [unwired: 2 in, 2 out]
        n606 = property on="Abort 5" class="Bool"("DisabledEnum"=w1155) -> ()  [unwired: 2 in, 2 out]
      }
      event "Abort 3": Value Change {
        n607 = event-data() -> ()  [unwired: 1 in, 3 out]
        n608 = call-dynamic "Read Channel Manager.lvclass.vi"("error in (no error)"=w1182, "SPARC4_AC in"=w1181) -> ("error out"=w1172:errorcluster, "Channel Manager.lvclass"=w1173:refnum<class "Channel Manager.lvclass">, "SPARC4_AC out"=w1183:refnum<class "SPARC4_AC.lvclass">)  [unwired: 7 in]
        n609 = call-dynamic "Read Available Cameras.vi"("error in (no error)"=w1172, "Channel Manager in"=w1173) -> ("error out"=w1175:errorcluster, "Available Cameras"=w1171:u8, "Channel Manager out"=w1174:refnum<class "Channel Manager.lvclass">)  [unwired: 7 in]
        n610 = for {
          N: w1171 -> [_]
          tunnel: "Abort 3" -> [w1191]
          shift-right: [w1190] -> w1176
          shift-left: w1174 -> [w1186]
          shift-right: [w1189] -> w1177
          shift-left: w1175 -> [w1185]
          i -> [w1184]
          n611 = call-dynamic "Write Current Camera.vi"("error in (no error)"=w1185, "Current Camera"=w1184, "Channel Manager in"=w1186) -> ("error out"=w1188:errorcluster, "Channel Manager out"=w1187:refnum<class "Channel Manager.lvclass">)  [unwired: 7 in]
          n612 = call "Return Current RxTx.vi"("error in (no error)"=w1188, "Channel Manager in"=w1187) -> ("error out"=w1199:errorcluster, "RxTx"=w1200:refnum<class "RxTx.lvclass">, "Channel Manager out"=w1196:refnum<class "Channel Manager.lvclass">)  [unwired: 7 in]
          n613 = call-dynamic "Read Interface.lvclass.vi"("error in (no error)"=w1199, "RxTx in"=w1200) -> ("error out"=w1192:errorcluster, "Interface.lvclass"=w1195:refnum<class "Interface.lvclass">, "RxTx out"=w1201:refnum<class "RxTx.lvclass">)  [unwired: 7 in]
          n614 = call-dynamic "Write Abort.vi"("error in (no error)"=w1192, "Abort"=w1191, "Interface in"=w1195) -> ("error out"=w1193:errorcluster, "Interface out"=w1194:refnum<class "Interface.lvclass">)  [unwired: 7 in]
          n615 = call-dynamic "Write Interface.lvclass.vi"("error in (no error)"=w1193, "Interface.lvclass"=w1194, "RxTx in"=w1201) -> ("error out"=w1197:errorcluster, "RxTx out"=w1198:refnum<class "RxTx.lvclass">)  [unwired: 7 in]
          n616 = call "Write Current RxTx.vi"("error in (no error)"=w1197, "RxTx"=w1198, "Channel Manager in"=w1196) -> ("error out"=w1189:errorcluster, "Channel Manager out"=w1190:refnum<class "Channel Manager.lvclass">)  [unwired: 7 in]
        }
        n617 = call-dynamic "Write Channel Manager.lvclass.vi"("error in (no error)"=w1177, "Channel Manager.lvclass"=w1176, "SPARC4_AC in"=w1183) -> ("error out"=w1179:errorcluster, "SPARC4_AC out"=w1180:refnum<class "SPARC4_AC.lvclass">)  [unwired: 7 in]
      }
      event "Stop Acq 3": Value Change {
        n618 = event-data() -> ()  [unwired: 1 in, 3 out]
        n619 = call-dynamic "Read Channel Manager.lvclass.vi"("error in (no error)"=w1205, "SPARC4_AC in"=w1204) -> ("error out"=w1208:errorcluster, "Channel Manager.lvclass"=w1209:refnum<class "Channel Manager.lvclass">, "SPARC4_AC out"=w1214:refnum<class "SPARC4_AC.lvclass">)  [unwired: 7 in]
        n620 = call-dynamic "Read Available Cameras.vi"("error in (no error)"=w1208, "Channel Manager in"=w1209) -> ("error out"=w1211:errorcluster, "Available Cameras"=w1207:u8, "Channel Manager out"=w1210:refnum<class "Channel Manager.lvclass">)  [unwired: 7 in]
        n621 = for {
          N: w1207 -> [_]
          shift-right: [w1226] -> w1212
          shift-left: w1210 -> [w1222]
          shift-right: [w1225] -> w1213
          shift-left: w1211 -> [w1221]
          tunnel: "Stop Acq 3" -> [w1215]
          i -> [w1220]
          n622 = call-dynamic "Write Current Camera.vi"("error in (no error)"=w1221, "Current Camera"=w1220, "Channel Manager in"=w1222) -> ("error out"=w1224:errorcluster, "Channel Manager out"=w1223:refnum<class "Channel Manager.lvclass">)  [unwired: 7 in]
          n623 = call "Return Current RxTx.vi"("error in (no error)"=w1224, "Channel Manager in"=w1223) -> ("error out"=w1230:errorcluster, "RxTx"=w1231:refnum<class "RxTx.lvclass">, "Channel Manager out"=w1227:refnum<class "Channel Manager.lvclass">)  [unwired: 7 in]
          n624 = call-dynamic "Read Interface.lvclass.vi"("error in (no error)"=w1230, "RxTx in"=w1231) -> ("error out"=w1219:errorcluster, "Interface.lvclass"=w1218:refnum<class "Interface.lvclass">, "RxTx out"=w1232:refnum<class "RxTx.lvclass">)  [unwired: 7 in]
          n625 = call-dynamic "Write Stop Acq.vi"("error in (no error)"=w1219, "Stop Acq"=w1215, "Interface in"=w1218) -> ("error out"=w1216:errorcluster, "Interface out"=w1217:refnum<class "Interface.lvclass">)  [unwired: 7 in]
          n626 = call-dynamic "Write Interface.lvclass.vi"("error in (no error)"=w1216, "Interface.lvclass"=w1217, "RxTx in"=w1232) -> ("error out"=w1228:errorcluster, "RxTx out"=w1229:refnum<class "RxTx.lvclass">)  [unwired: 7 in]
          n627 = call "Write Current RxTx.vi"("error in (no error)"=w1228, "RxTx"=w1229, "Channel Manager in"=w1227) -> ("error out"=w1225:errorcluster, "Channel Manager out"=w1226:refnum<class "Channel Manager.lvclass">)  [unwired: 7 in]
        }
        n628 = call-dynamic "Write Channel Manager.lvclass.vi"("error in (no error)"=w1213, "Channel Manager.lvclass"=w1212, "SPARC4_AC in"=w1214) -> ("error out"=w1203:errorcluster, "SPARC4_AC out"=w1202:refnum<class "SPARC4_AC.lvclass">)  [unwired: 7 in]
      }
      event "Pausar 3": Value Change {
        n629 = event-data() -> ()  [unwired: 1 in, 3 out]
        n630 = call-dynamic "Read Channel Manager.lvclass.vi"("error in (no error)"=w1236, "SPARC4_AC in"=w1235) -> ("error out"=w1239:errorcluster, "Channel Manager.lvclass"=w1240:refnum<class "Channel Manager.lvclass">, "SPARC4_AC out"=w1245:refnum<class "SPARC4_AC.lvclass">)  [unwired: 7 in]
        n631 = call-dynamic "Read Available Cameras.vi"("error in (no error)"=w1239, "Channel Manager in"=w1240) -> ("error out"=w1242:errorcluster, "Available Cameras"=w1238:u8, "Channel Manager out"=w1241:refnum<class "Channel Manager.lvclass">)  [unwired: 7 in]
        n632 = for {
          N: w1238 -> [_]
          shift-right: [w1257] -> w1243
          shift-left: w1241 -> [w1253]
          shift-right: [w1256] -> w1244
          shift-left: w1242 -> [w1252]
          tunnel: "Pausar 3" -> [w1246]
          i -> [w1251]
          n633 = call-dynamic "Write Current Camera.vi"("error in (no error)"=w1252, "Current Camera"=w1251, "Channel Manager in"=w1253) -> ("error out"=w1255:errorcluster, "Channel Manager out"=w1254:refnum<class "Channel Manager.lvclass">)  [unwired: 7 in]
          n634 = call "Return Current RxTx.vi"("error in (no error)"=w1255, "Channel Manager in"=w1254) -> ("error out"=w1261:errorcluster, "RxTx"=w1262:refnum<class "RxTx.lvclass">, "Channel Manager out"=w1258:refnum<class "Channel Manager.lvclass">)  [unwired: 7 in]
          n635 = call-dynamic "Read Interface.lvclass.vi"("error in (no error)"=w1261, "RxTx in"=w1262) -> ("error out"=w1247:errorcluster, "Interface.lvclass"=w1248:refnum<class "Interface.lvclass">, "RxTx out"=w1263:refnum<class "RxTx.lvclass">)  [unwired: 7 in]
          n636 = call-dynamic "Write Pause Acq.vi"("error in (no error)"=w1247, "Pause Acq"=w1246, "Interface in"=w1248) -> ("error out"=w1250:errorcluster, "Interface out"=w1249:refnum<class "Interface.lvclass">)  [unwired: 7 in]
          n637 = call-dynamic "Write Interface.lvclass.vi"("error in (no error)"=w1250, "Interface.lvclass"=w1249, "RxTx in"=w1263) -> ("error out"=w1259:errorcluster, "RxTx out"=w1260:refnum<class "RxTx.lvclass">)  [unwired: 7 in]
          n638 = call "Write Current RxTx.vi"("error in (no error)"=w1259, "RxTx"=w1260, "Channel Manager in"=w1258) -> ("error out"=w1256:errorcluster, "Channel Manager out"=w1257:refnum<class "Channel Manager.lvclass">)  [unwired: 7 in]
        }
        n639 = call-dynamic "Write Channel Manager.lvclass.vi"("error in (no error)"=w1244, "Channel Manager.lvclass"=w1243, "SPARC4_AC in"=w1245) -> ("error out"=w1233:errorcluster, "SPARC4_AC out"=w1234:refnum<class "SPARC4_AC.lvclass">)  [unwired: 7 in]
      }
      event "Sync Mode: 2": Value Change {
        n640 = event-data() -> ()  [unwired: 1 in, 3 out]
        n641 = Increment(x="Sync Mode: 2") -> (x+1=w1267:T3)
        n642 = call-dynamic "Write Sync Mode.vi"("error in (no error)"=w1269, "Sync Mode"=w1267, "SPARC4_AC in"=w1268) -> ("error out"=w1265:errorcluster, "SPARC4_AC out"=w1264:refnum<class "SPARC4_AC.lvclass">)  [unwired: 7 in]
      }
      event "Adquirir 4": Value Change {
        w1275 = u8 4 items=["Full Vertical Binning", "Multi-Track", "Random-track", "Single-Track", "Image"] ("Read Mode")
        w1278 = u8 3 items=["0.6", "1.13", "2.2", "4.33"] ("Vertical Shift \nSpeed")
        w1277 = u8 3 items=["N/A", "Single", "Accumulate", "Kinetic", "Fast Kinetic"] ("Acquisition Mode")
        w1276 = u8 6 items=["Internal", "External", "RESERVED", "RESERVED", "RESERVED", "RESERVED", "External Start"] ("Trigger")
        w1274 = u8 2 items=["Fully Auto", "OPEN", "CLOSED"] ("Shutter Mode")
        w1273 = u8 0 items=["TTL Low", "TTl High"] ("Shutter TTL")
        w1272 = u16 50 ("Time to open shutter")
        n643 = event-data() -> ()  [unwired: 1 in, 3 out]
        n644 = local read "Night Directory"() -> (w1270:string)
        n645 = call-dynamic "Read Channel Manager.lvclass.vi"("error in (no error)"=w1324, "SPARC4_AC in"=w1323) -> ("error out"=w1282:errorcluster, "Channel Manager.lvclass"=w1281:refnum<class "Channel Manager.lvclass">, "SPARC4_AC out"=w1325:refnum<class "SPARC4_AC.lvclass">)  [unwired: 7 in]
        n646 = call-dynamic "Write Current Camera.vi"("error in (no error)"=w1282, "Current Camera"=2, "Channel Manager in"=w1281) -> ("error out"=w1284:errorcluster, "Channel Manager out"=w1283:refnum<class "Channel Manager.lvclass">)  [unwired: 7 in]
        n647 = call "Return Current RxTx.vi"("error in (no error)"=w1284, "Channel Manager in"=w1283) -> ("error out"=w1308:errorcluster, "RxTx"=w1309:refnum<class "RxTx.lvclass">, "Channel Manager out"=w1312:refnum<class "Channel Manager.lvclass">)  [unwired: 7 in]
        n648 = local write "Exposições realizadas 3"(u8 0 ("Exposições realizadas")) -> ()
        n649 = call-dynamic "Read Interface.lvclass.vi"("error in (no error)"=w1308, "RxTx in"=w1309) -> ("error out"=w1314:errorcluster, "Interface.lvclass"=w1313:refnum<class "Interface.lvclass">, "RxTx out"=w1317:refnum<class "RxTx.lvclass">)  [unwired: 7 in]
        n650 = local read "Camera Setup"() -> (w1285:T1)
        n651 = Bundle By Name(cluster=w1285, "Image Name"="Image Name 3", "Image Path"=w1270, "# Images"="# Images 3", "Exposure Time"="Exposure Time 7", "Pre-amp gain"="Pre-amp gain 3", "Readout Rate"="Readout Rate 3", "Vertical Shift Speed"=w1278, "Acquisition Mode"=w1277, "Trigger"=w1276, "Read Mode"=w1275, "EM Mode"="EM Mode 3", "EM Gain"="EM Gain 3", "Shutter Mode"=w1274, "Shutter TTL"=w1273, "Time to open shutter"=w1272, "Time to close shutter"=w1272, "Vertical Binning"="Binning 7", "Horizontal Binning"="Binning 7", "Initial Line"="Initial Line 3", "Initial Cloumn"="Initial Cloumn 3", "Final Line"="Final Line 3", "Final Column"="Final Column 3") -> (w1286:T1)
        n652 = call-dynamic "Write Exposições realizadas.vi"("error in (no error)"=w1314, "Exposições realizadas"=0, "Interface in"=w1313) -> ("error out"=w1316:errorcluster, "Interface out"=w1315:refnum<class "Interface.lvclass">)  [unwired: 7 in]
        n653 = call "Write Camera Setup.vi"("error in (no error)"=w1316, "Camera Setup"=w1286, "Interface in"=w1315) -> ("error out"=w1319:errorcluster, "Interface out"=w1318:refnum<class "Interface.lvclass">)  [unwired: 7 in]
        n654 = call-dynamic "Write Interface.lvclass.vi"("error in (no error)"=w1319, "Interface.lvclass"=w1318, "RxTx in"=w1317) -> ("error out"=w1310:errorcluster, "RxTx out"=w1311:refnum<class "RxTx.lvclass">)  [unwired: 7 in]
        n655 = call "Write Current RxTx.vi"("error in (no error)"=w1310, "RxTx"=w1311, "Channel Manager in"=w1312) -> ("error out"=w1306:errorcluster, "Channel Manager out"=w1307:refnum<class "Channel Manager.lvclass">)  [unwired: 7 in]
        n656 = call "Read Current State Machine.vi"("error in (no error)"=w1306, "Channel Manager in"=w1307) -> ("error out"=w1304:errorcluster, "State Machine.lvclass"=w1305:refnum<class "State Machine.lvclass">, "Channel Manager out"=w1301:refnum<class "Channel Manager.lvclass">)  [unwired: 7 in]
        n657 = call "Next State.vi"("error in (no error)"=w1304, "New_State"=u32 2, "State Machine in"=w1305) -> ("error out"=w1303:errorcluster, "State Machine out"=w1302:refnum<class "State Machine.lvclass">)  [unwired: 7 in]
        n658 = call "Write Current State Machine.vi"("error in (no error)"=w1303, "State Machine.lvclass"=w1302, "Channel Manager in"=w1301) -> ("error out"=w1320:errorcluster, "Channel Manager out"=w1280:refnum<class "Channel Manager.lvclass">)  [unwired: 7 in]
        n659 = call-dynamic "Write Channel Manager.lvclass.vi"("error in (no error)"=w1320, "Channel Manager.lvclass"=w1280, "SPARC4_AC in"=w1325) -> ("error out"=w1321:errorcluster, "SPARC4_AC out"=w1322:refnum<class "SPARC4_AC.lvclass">)  [unwired: 7 in]
      }
      event "Stop Acq 4": Value Change {
        n660 = event-data() -> ()  [unwired: 1 in, 3 out]
        n661 = call-dynamic "Read Channel Manager.lvclass.vi"("error in (no error)"=w1347, "SPARC4_AC in"=w1346) -> ("error out"=w1328:errorcluster, "Channel Manager.lvclass"=w1327:refnum<class "Channel Manager.lvclass">, "SPARC4_AC out"=w1348:refnum<class "SPARC4_AC.lvclass">)  [unwired: 7 in]
        n662 = call-dynamic "Write Current Camera.vi"("error in (no error)"=w1328, "Current Camera"=2, "Channel Manager in"=w1327) -> ("error out"=w1331:errorcluster, "Channel Manager out"=w1330:refnum<class "Channel Manager.lvclass">)  [unwired: 7 in]
        n663 = call "Return Current RxTx.vi"("error in (no error)"=w1331, "Channel Manager in"=w1330) -> ("error out"=w1336:errorcluster, "RxTx"=w1337:refnum<class "RxTx.lvclass">, "Channel Manager out"=w1333:refnum<class "Channel Manager.lvclass">)  [unwired: 7 in]
        n664 = call-dynamic "Read Interface.lvclass.vi"("error in (no error)"=w1336, "RxTx in"=w1337) -> ("error out"=w1341:errorcluster, "Interface.lvclass"=w1342:refnum<class "Interface.lvclass">, "RxTx out"=w1338:refnum<class "RxTx.lvclass">)  [unwired: 7 in]
        n665 = call-dynamic "Write Stop Acq.vi"("error in (no error)"=w1341, "Stop Acq"="Stop Acq 4", "Interface in"=w1342) -> ("error out"=w1340:errorcluster, "Interface out"=w1339:refnum<class "Interface.lvclass">)  [unwired: 7 in]
        n666 = call-dynamic "Write Interface.lvclass.vi"("error in (no error)"=w1340, "Interface.lvclass"=w1339, "RxTx in"=w1338) -> ("error out"=w1334:errorcluster, "RxTx out"=w1335:refnum<class "RxTx.lvclass">)  [unwired: 7 in]
        n667 = call "Write Current RxTx.vi"("error in (no error)"=w1334, "RxTx"=w1335, "Channel Manager in"=w1333) -> ("error out"=w1343:errorcluster, "Channel Manager out"=w1326:refnum<class "Channel Manager.lvclass">)  [unwired: 7 in]
        n668 = call-dynamic "Write Channel Manager.lvclass.vi"("error in (no error)"=w1343, "Channel Manager.lvclass"=w1326, "SPARC4_AC in"=w1348) -> ("error out"=w1344:errorcluster, "SPARC4_AC out"=w1345:refnum<class "SPARC4_AC.lvclass">)  [unwired: 7 in]
      }
      event "Pausar 4": Value Change {
        n669 = event-data() -> ()  [unwired: 1 in, 3 out]
        n670 = call-dynamic "Read Channel Manager.lvclass.vi"("error in (no error)"=w1370, "SPARC4_AC in"=w1369) -> ("error out"=w1350:errorcluster, "Channel Manager.lvclass"=w1351:refnum<class "Channel Manager.lvclass">, "SPARC4_AC out"=w1371:refnum<class "SPARC4_AC.lvclass">)  [unwired: 7 in]
        n671 = call-dynamic "Write Current Camera.vi"("error in (no error)"=w1350, "Current Camera"=2, "Channel Manager in"=w1351) -> ("error out"=w1354:errorcluster, "Channel Manager out"=w1353:refnum<class "Channel Manager.lvclass">)  [unwired: 7 in]
        n672 = call "Return Current RxTx.vi"("error in (no error)"=w1354, "Channel Manager in"=w1353) -> ("error out"=w1363:errorcluster, "RxTx"=w1364:refnum<class "RxTx.lvclass">, "Channel Manager out"=w1360:refnum<class "Channel Manager.lvclass">)  [unwired: 7 in]
        n673 = call-dynamic "Read Interface.lvclass.vi"("error in (no error)"=w1363, "RxTx in"=w1364) -> ("error out"=w1356:errorcluster, "Interface.lvclass"=w1359:refnum<class "Interface.lvclass">, "RxTx out"=w1365:refnum<class "RxTx.lvclass">)  [unwired: 7 in]
        n674 = call-dynamic "Write Pause Acq.vi"("error in (no error)"=w1356, "Pause Acq"="Pausar 4", "Interface in"=w1359) -> ("error out"=w1357:errorcluster, "Interface out"=w1358:refnum<class "Interface.lvclass">)  [unwired: 7 in]
        n675 = call-dynamic "Write Interface.lvclass.vi"("error in (no error)"=w1357, "Interface.lvclass"=w1358, "RxTx in"=w1365) -> ("error out"=w1361:errorcluster, "RxTx out"=w1362:refnum<class "RxTx.lvclass">)  [unwired: 7 in]
        n676 = call "Write Current RxTx.vi"("error in (no error)"=w1361, "RxTx"=w1362, "Channel Manager in"=w1360) -> ("error out"=w1366:errorcluster, "Channel Manager out"=w1352:refnum<class "Channel Manager.lvclass">)  [unwired: 7 in]
        n677 = call-dynamic "Write Channel Manager.lvclass.vi"("error in (no error)"=w1366, "Channel Manager.lvclass"=w1352, "SPARC4_AC in"=w1371) -> ("error out"=w1367:errorcluster, "SPARC4_AC out"=w1368:refnum<class "SPARC4_AC.lvclass">)  [unwired: 7 in]
      }
      event "Abort 4": Value Change {
        n678 = event-data() -> ()  [unwired: 1 in, 3 out]
        n679 = call-dynamic "Read Channel Manager.lvclass.vi"("error in (no error)"=w1393, "SPARC4_AC in"=w1392) -> ("error out"=w1373:errorcluster, "Channel Manager.lvclass"=w1374:refnum<class "Channel Manager.lvclass">, "SPARC4_AC out"=w1394:refnum<class "SPARC4_AC.lvclass">)  [unwired: 7 in]
        n680 = call-dynamic "Write Current Camera.vi"("error in (no error)"=w1373, "Current Camera"=2, "Channel Manager in"=w1374) -> ("error out"=w1376:errorcluster, "Channel Manager out"=w1375:refnum<class "Channel Manager.lvclass">)  [unwired: 7 in]
        n681 = call "Return Current RxTx.vi"("error in (no error)"=w1376, "Channel Manager in"=w1375) -> ("error out"=w1386:errorcluster, "RxTx"=w1387:refnum<class "RxTx.lvclass">, "Channel Manager out"=w1383:refnum<class "Channel Manager.lvclass">)  [unwired: 7 in]
        n682 = call-dynamic "Read Interface.lvclass.vi"("error in (no error)"=w1386, "RxTx in"=w1387) -> ("error out"=w1380:errorcluster, "Interface.lvclass"=w1381:refnum<class "Interface.lvclass">, "RxTx out"=w1388:refnum<class "RxTx.lvclass">)  [unwired: 7 in]
        n683 = call-dynamic "Write Abort.vi"("error in (no error)"=w1380, "Abort"="Abort 4", "Interface in"=w1381) -> ("error out"=w1379:errorcluster, "Interface out"=w1382:refnum<class "Interface.lvclass">)  [unwired: 7 in]
        n684 = call-dynamic "Write Interface.lvclass.vi"("error in (no error)"=w1379, "Interface.lvclass"=w1382, "RxTx in"=w1388) -> ("error out"=w1384:errorcluster, "RxTx out"=w1385:refnum<class "RxTx.lvclass">)  [unwired: 7 in]
        n685 = call "Write Current RxTx.vi"("error in (no error)"=w1384, "RxTx"=w1385, "Channel Manager in"=w1383) -> ("error out"=w1389:errorcluster, "Channel Manager out"=w1377:refnum<class "Channel Manager.lvclass">)  [unwired: 7 in]
        n686 = call-dynamic "Write Channel Manager.lvclass.vi"("error in (no error)"=w1389, "Channel Manager.lvclass"=w1377, "SPARC4_AC in"=w1394) -> ("error out"=w1390:errorcluster, "SPARC4_AC out"=w1391:refnum<class "SPARC4_AC.lvclass">)  [unwired: 7 in]
      }
      event "Cooler ON/OFF 3": Value Change {
        n687 = event-data() -> ()  [unwired: 1 in, 3 out]
        n688 = call-dynamic "Read Channel Manager.lvclass.vi"("error in (no error)"=w1423, "SPARC4_AC in"=w1422) -> ("error out"=w1396:errorcluster, "Channel Manager.lvclass"=w1397:refnum<class "Channel Manager.lvclass">, "SPARC4_AC out"=w1424:refnum<class "SPARC4_AC.lvclass">)  [unwired: 7 in]
        n689 = call-dynamic "Write Current Camera.vi"("error in (no error)"=w1396, "Current Camera"=2, "Channel Manager in"=w1397) -> ("error out"=w1400:errorcluster, "Channel Manager out"=w1399:refnum<class "Channel Manager.lvclass">)  [unwired: 7 in]
        n690 = local read "Camera Setup"() -> (w1401:T1)
        n691 = Bundle By Name(cluster=w1401, "Cooler ON/OFF"="Cooler ON/OFF 3") -> (w1402:T1)
        n692 = case shown="0, Default" "Cooler ON/OFF 3" {
          tunnel: ["TURN COOLER OFF" "TURN COOLER ON"] -> w1412
          frame 0, Default {
          }
          frame 1 {
          }
        }
        n693 = call "Return Current RxTx.vi"("error in (no error)"=w1400, "Channel Manager in"=w1399) -> ("error out"=w1404:errorcluster, "RxTx"=w1405:refnum<class "RxTx.lvclass">, "Channel Manager out"=w1408:refnum<class "Channel Manager.lvclass">)  [unwired: 7 in]
        n694 = call-dynamic "Read Interface.lvclass.vi"("error in (no error)"=w1404, "RxTx in"=w1405) -> ("error out"=w1417:errorcluster, "Interface.lvclass"=w1418:refnum<class "Interface.lvclass">, "RxTx out"=w1409:refnum<class "RxTx.lvclass">)  [unwired: 7 in]
        n695 = call "Write Camera Setup.vi"("error in (no error)"=w1417, "Camera Setup"=w1402, "Interface in"=w1418) -> ("error out"=w1410:errorcluster, "Interface out"=w1411:refnum<class "Interface.lvclass">)  [unwired: 7 in]
        n696 = call "Write Command.vi"("error in (no error)"=w1410, "Command"=w1412, "Interface in"=w1411) -> ("error out"=w1414:errorcluster, "Interface out"=w1413:refnum<class "Interface.lvclass">)  [unwired: 7 in]
        n697 = call-dynamic "Write Interface.lvclass.vi"("error in (no error)"=w1414, "Interface.lvclass"=w1413, "RxTx in"=w1409) -> ("error out"=w1416:errorcluster, "RxTx out"=w1415:refnum<class "RxTx.lvclass">)  [unwired: 7 in]
        n698 = call "Enqeue A Message.vi"("error in (no error)"=w1416, "RxTx in"=w1415) -> ("error out"=w1406:errorcluster, "RxTx out"=w1407:refnum<class "RxTx.lvclass">)  [unwired: 8 in]
        n699 = call "Write Current RxTx.vi"("error in (no error)"=w1406, "RxTx"=w1407, "Channel Manager in"=w1408) -> ("error out"=w1419:errorcluster, "Channel Manager out"=w1398:refnum<class "Channel Manager.lvclass">)  [unwired: 7 in]
        n700 = call-dynamic "Write Channel Manager.lvclass.vi"("error in (no error)"=w1419, "Channel Manager.lvclass"=w1398, "SPARC4_AC in"=w1424) -> ("error out"=w1420:errorcluster, "SPARC4_AC out"=w1421:refnum<class "SPARC4_AC.lvclass">)  [unwired: 7 in]
      }
      event "Set temperature 3": Value Change {
        n701 = event-data() -> ()  [unwired: 1 in, 3 out]
        n702 = call-dynamic "Read Channel Manager.lvclass.vi"("error in (no error)"=w1454, "SPARC4_AC in"=w1455) -> ("error out"=w1428:errorcluster, "Channel Manager.lvclass"=w1427:refnum<class "Channel Manager.lvclass">, "SPARC4_AC out"=w1456:refnum<class "SPARC4_AC.lvclass">)  [unwired: 7 in]
        n703 = call-dynamic "Write Current Camera.vi"("error in (no error)"=w1428, "Current Camera"=2, "Channel Manager in"=w1427) -> ("error out"=w1432:errorcluster, "Channel Manager out"=w1431:refnum<class "Channel Manager.lvclass">)  [unwired: 7 in]
        n704 = call "Return Current RxTx.vi"("error in (no error)"=w1432, "Channel Manager in"=w1431) -> ("error out"=w1435:errorcluster, "RxTx"=w1438:refnum<class "RxTx.lvclass">, "Channel Manager out"=w1439:refnum<class "Channel Manager.lvclass">)  [unwired: 7 in]
        n705 = call-dynamic "Read Interface.lvclass.vi"("error in (no error)"=w1435, "RxTx in"=w1438) -> ("error out"=w1444:errorcluster, "Interface.lvclass"=w1443:refnum<class "Interface.lvclass">, "RxTx out"=w1450:refnum<class "RxTx.lvclass">)  [unwired: 7 in]
        n706 = local read "Camera Setup"() -> (w1433:T1)
        n707 = Bundle By Name(cluster=w1433, "Set temperature"="Set temperature 3") -> (w1442:T1)
        n708 = call "Write Camera Setup.vi"("error in (no error)"=w1444, "Camera Setup"=w1442, "Interface in"=w1443) -> ("error out"=w1441:errorcluster, "Interface out"=w1440:refnum<class "Interface.lvclass">)  [unwired: 7 in]
        n709 = call "Write Command.vi"("error in (no error)"=w1441, "Command"="SET TEMPERATURE", "Interface in"=w1440) -> ("error out"=w1448:errorcluster, "Interface out"=w1449:refnum<class "Interface.lvclass">)  [unwired: 7 in]
        n710 = call-dynamic "Write Interface.lvclass.vi"("error in (no error)"=w1448, "Interface.lvclass"=w1449, "RxTx in"=w1450) -> ("error out"=w1446:errorcluster, "RxTx out"=w1447:refnum<class "RxTx.lvclass">)  [unwired: 7 in]
        n711 = call "Enqeue A Message.vi"("error in (no error)"=w1446, "RxTx in"=w1447) -> ("error out"=w1436:errorcluster, "RxTx out"=w1437:refnum<class "RxTx.lvclass">)  [unwired: 8 in]
        n712 = call "Write Current RxTx.vi"("error in (no error)"=w1436, "RxTx"=w1437, "Channel Manager in"=w1439) -> ("error out"=w1451:errorcluster, "Channel Manager out"=w1430:refnum<class "Channel Manager.lvclass">)  [unwired: 7 in]
        n713 = call-dynamic "Write Channel Manager.lvclass.vi"("error in (no error)"=w1451, "Channel Manager.lvclass"=w1430, "SPARC4_AC in"=w1456) -> ("error out"=w1453:errorcluster, "SPARC4_AC out"=w1452:refnum<class "SPARC4_AC.lvclass">)  [unwired: 7 in]
        "Temperature ºC 3" <- "Set temperature 3"
      }
      event "Exposure Time 5": Value Change {
        n714 = event-data() -> ()  [unwired: 1 in, 3 out]
        n715 = local write "Exposure Time 7"("Exposure Time 5") -> ()
      }
      event "# Images 3": Value Change {
        n716 = event-data() -> ()  [unwired: 1 in, 3 out]
        n717 = local read "# Images 3"() -> (w1462:u32)
        n718 = property on="Exposições realizadas 3" class="Slide (strict)"("Scale.Maximum"=w1462) -> ()  [unwired: 2 in, 2 out]
      }
      event "Exposure Time 7": Value Change {
        n719 = event-data() -> ()  [unwired: 1 in, 3 out]
        n720 = local read "Exposure Time 7"() -> (w1465:dbl)
        n721 = local write "Exposure Time 5"(w1465) -> ()
      }
      event "Sub Image 3": Value Change {
        n722 = event-data() -> ()  [unwired: 1 in, 3 out]
        n723 = call-dynamic "Read Channel Manager.lvclass.vi"("error in (no error)"=w1481, "SPARC4_AC in"=w1480) -> ("error out"=w1469:errorcluster, "Channel Manager.lvclass"=w1468:refnum<class "Channel Manager.lvclass">, "SPARC4_AC out"=w1486:refnum<class "SPARC4_AC.lvclass">)  [unwired: 7 in]
        n724 = call-dynamic "Write Current Camera.vi"("error in (no error)"=w1469, "Current Camera"=2, "Channel Manager in"=w1468) -> ("error out"=w1470:errorcluster, "Channel Manager out"=w1471:refnum<class "Channel Manager.lvclass">)  [unwired: 7 in]
        n725 = call "Return Current RxTx.vi"("error in (no error)"=w1470, "Channel Manager in"=w1471) -> ("error out"=w1498:errorcluster, "RxTx"=w1499:refnum<class "RxTx.lvclass">, "Channel Manager out"=w1466:refnum<class "Channel Manager.lvclass">)  [unwired: 7 in]
        n726 = call-dynamic "Read Interface.lvclass.vi"("error in (no error)"=w1498, "RxTx in"=w1499) -> ("error out"=w1496:errorcluster, "Interface.lvclass"=w1497:refnum<class "Interface.lvclass">)  [unwired: 7 in, 1 out]
        n727 = call "Read Camera Status.vi"("error in (no error)"=w1496, "Interface in"=w1497) -> ("error out"=w1487:errorcluster, "Camera Status"=w1495:T6)  [unwired: 7 in, 1 out]
        n728 = Unbundle By Name(w1495) -> ("Final Column"=w1492:u16, "Final Line"=w1491:u16)
        n729 = call-dynamic "Write Channel Manager.lvclass.vi"("error in (no error)"=w1487, "Channel Manager.lvclass"=w1466, "SPARC4_AC in"=w1486) -> ("error out"=w1485:errorcluster, "SPARC4_AC out"=w1484:refnum<class "SPARC4_AC.lvclass">)  [unwired: 7 in]
        n730 = case shown="\"256 x 256\"" "Sub Image 3" {
          tunnel: [128 256 512 512] -> w1490
          frame "256 x 256" {
          }
          frame "512 x 512" {
          }
          frame "1024 x 1024", Default {
          }
          frame "Custom" {
          }
        }
        n731 = case shown="\"1024 x 1024\", Default" "Sub Image 3" {
          tunnel: [T7."Disabled and Grayed Out" ("Disabled") T7."Enabled" ("Disabled")] -> w1476
          frame "1024 x 1024", Default {
          }
          frame "Custom" {
          }
        }
        n732 = Divide(x=w1492, y=2) -> (x/y=w1493:dbl)
        n733 = Divide(x=w1491, y=2) -> (x/y=w1494:dbl)
        n734 = Add(x=w1493, y=w1490) -> (x+y=w1475:dbl)
        n735 = Subtract(x=w1493, y=w1490) -> (x-y=w1489:dbl)
        n736 = Subtract(x=w1494, y=w1490) -> (x-y=w1488:dbl)
        n737 = Add(x=w1494, y=w1490) -> (x+y=w1472:dbl)
        n738 = Increment(x=w1489) -> (x+1=w1474:dbl)
        n739 = Increment(x=w1488) -> (x+1=w1473:dbl)
        n740 = local write "Initial Line 3"(w1475) -> ()
        n741 = local write "Initial Cloumn 3"(w1474) -> ()
        n742 = local write "Final Line 3"(w1473) -> ()
        n743 = local write "Final Column 3"(w1472) -> ()
        n744 = property on="Initial Line 3" class="DigNum (strict)"("DisabledEnum"=w1476) -> ()  [unwired: 2 in, 2 out]
        n745 = property on="Initial Cloumn 3" class="DigNum (strict)"("DisabledEnum"=w1476) -> ()  [unwired: 2 in, 2 out]
        n746 = property on="Final Column 3" class="DigNum (strict)"("DisabledEnum"=w1476) -> ()  [unwired: 2 in, 2 out]
        n747 = property on="Final Line 3" class="DigNum (strict)"("DisabledEnum"=w1476) -> ()  [unwired: 2 in, 2 out]
        n748 = flat-sequence {
          tunnel: w1485 -> [w1510]
          tunnel: w1484 -> [w1511]
          tunnel: [w1511] -> w1479
          tunnel: [w1510] -> w1478
          frame #0 {
            w1504 = cluster{dbl, dbl} {0.0, 0.0}
            n749 = local read "Initial Cloumn 3"() -> (w1503:u16)
            n750 = local read "Final Column 3"() -> (w1501:u16)
            n751 = local read "Initial Line 3"() -> (w1502:u16)
            n752 = local read "Final Line 3"() -> (w1500:u16)
            n753 = Bundle(cluster=w1504, w1503, w1502) -> (w1509:cluster{dbl, dbl})
            n754 = Bundle(cluster=w1504, w1503, w1500) -> (w1508:cluster{dbl, dbl})
            n755 = Bundle(cluster=w1504, w1501, w1500) -> (w1507:cluster{dbl, dbl})
            n756 = Bundle(cluster=w1504, w1501, w1502) -> (w1506:cluster{dbl, dbl})
            n757 = Bundle(cluster=w1504, w1503, w1502) -> (w1505:cluster{dbl, dbl})
            n758 = Build Array(w1509, w1508, w1507, w1506, w1505) -> ()  [unwired: 1 out]
          }
        }
      }
      event "Final Line 3", "Final Column 3", "Initial Cloumn 3", "Initial Line 3": Value Change {
        n759 = event-data() -> ()  [unwired: 1 in, 3 out]
        n760 = disable-structure shown="Disabled" {
          frame Disabled {
            w1520 = cluster{dbl, dbl} {0.0, 0.0}
            n761 = local read "Initial Cloumn 3"() -> (w1524:u16)
            n762 = local read "Final Column 3"() -> (w1522:u16)
            n763 = local read "Initial Line 3"() -> (w1523:u16)
            n764 = local read "Final Line 3"() -> (w1521:u16)
            n765 = Bundle(cluster=w1520, w1524, w1523) -> (w1529:cluster{dbl, dbl})
            n766 = Bundle(cluster=w1520, w1524, w1521) -> (w1528:cluster{dbl, dbl})
            n767 = Bundle(cluster=w1520, w1522, w1521) -> (w1527:cluster{dbl, dbl})
            n768 = Bundle(cluster=w1520, w1522, w1523) -> (w1526:cluster{dbl, dbl})
            n769 = Bundle(cluster=w1520, w1524, w1523) -> (w1525:cluster{dbl, dbl})
            n770 = Build Array(w1529, w1528, w1527, w1526, w1525) -> ()  [unwired: 1 out]
          }
          frame Enabled {
          }
        }
      }
      event "Adquirir 5": Value Change {
        w1535 = u8 4 items=["Full Vertical Binning", "Multi-Track", "Random-track", "Single-Track", "Image"] ("Read Mode")
        w1538 = u8 3 items=["0.6", "1.13", "2.2", "4.33"] ("Vertical Shift \nSpeed")
        w1537 = u8 3 items=["N/A", "Single", "Accumulate", "Kinetic", "Fast Kinetic"] ("Acquisition Mode")
        w1536 = u8 6 items=["Internal", "External", "RESERVED", "RESERVED", "RESERVED", "RESERVED", "External Start"] ("Trigger")
        w1534 = u8 2 items=["Fully Auto", "OPEN", "CLOSED"] ("Shutter Mode")
        w1533 = u8 0 items=["TTL Low", "TTl High"] ("Shutter TTL")
        w1532 = u16 50 ("Time to open shutter")
        n771 = event-data() -> ()  [unwired: 1 in, 1 out]
        n772 = local read "Night Directory"() -> (w1530:string)
        n773 = call-dynamic "Read Channel Manager.lvclass.vi"("error in (no error)"=w1583, "SPARC4_AC in"=w1584) -> ("error out"=w1542:errorcluster, "Channel Manager.lvclass"=w1541:refnum<class "Channel Manager.lvclass">, "SPARC4_AC out"=w1585:refnum<class "SPARC4_AC.lvclass">)  [unwired: 7 in]
        n774 = call-dynamic "Write Current Camera.vi"("error in (no error)"=w1542, "Current Camera"=3, "Channel Manager in"=w1541) -> ("error out"=w1544:errorcluster, "Channel Manager out"=w1543:refnum<class "Channel Manager.lvclass">)  [unwired: 7 in]
        n775 = call "Return Current RxTx.vi"("error in (no error)"=w1544, "Channel Manager in"=w1543) -> ("error out"=w1568:errorcluster, "RxTx"=w1569:refnum<class "RxTx.lvclass">, "Channel Manager out"=w1572:refnum<class "Channel Manager.lvclass">)  [unwired: 7 in]
        n776 = local write "Exposições realizadas 4"(u8 0 ("Exposições realizadas")) -> ()
        n777 = call-dynamic "Read Interface.lvclass.vi"("error in (no error)"=w1568, "RxTx in"=w1569) -> ("error out"=w1574:errorcluster, "Interface.lvclass"=w1573:refnum<class "Interface.lvclass">, "RxTx out"=w1577:refnum<class "RxTx.lvclass">)  [unwired: 7 in]
        n778 = local read "Camera Setup"() -> (w1545:T1)
        n779 = Bundle By Name(cluster=w1545, "Image Name"="Image Name 4", "Image Path"=w1530, "# Images"="# Images 4", "Exposure Time"="Exposure Time 8", "Pre-amp gain"="Pre-amp gain 4", "Readout Rate"="Readout Rate 4", "Vertical Shift Speed"=w1538, "Acquisition Mode"=w1537, "Trigger"=w1536, "Read Mode"=w1535, "EM Mode"="EM Mode 4", "EM Gain"="EM Gain 4", "Shutter Mode"=w1534, "Shutter TTL"=w1533, "Time to open shutter"=w1532, "Time to close shutter"=w1532, "Vertical Binning"="Binning 8", "Horizontal Binning"="Binning 8", "Initial Line"="Initial Line 4", "Initial Cloumn"="Initial Cloumn 4", "Final Line"="Final Line 4", "Final Column"="Final Column 4") -> (w1557:T1)
        n780 = call-dynamic "Write Exposições realizadas.vi"("error in (no error)"=w1574, "Exposições realizadas"=0, "Interface in"=w1573) -> ("error out"=w1576:errorcluster, "Interface out"=w1575:refnum<class "Interface.lvclass">)  [unwired: 7 in]
        n781 = call "Write Camera Setup.vi"("error in (no error)"=w1576, "Camera Setup"=w1557, "Interface in"=w1575) -> ("error out"=w1579:errorcluster, "Interface out"=w1578:refnum<class "Interface.lvclass">)  [unwired: 7 in]
        n782 = call-dynamic "Write Interface.lvclass.vi"("error in (no error)"=w1579, "Interface.lvclass"=w1578, "RxTx in"=w1577) -> ("error out"=w1570:errorcluster, "RxTx out"=w1571:refnum<class "RxTx.lvclass">)  [unwired: 7 in]
        n783 = call "Write Current RxTx.vi"("error in (no error)"=w1570, "RxTx"=w1571, "Channel Manager in"=w1572) -> ("error out"=w1566:errorcluster, "Channel Manager out"=w1567:refnum<class "Channel Manager.lvclass">)  [unwired: 7 in]
        n784 = call "Read Current State Machine.vi"("error in (no error)"=w1566, "Channel Manager in"=w1567) -> ("error out"=w1564:errorcluster, "State Machine.lvclass"=w1565:refnum<class "State Machine.lvclass">, "Channel Manager out"=w1561:refnum<class "Channel Manager.lvclass">)  [unwired: 7 in]
        n785 = call "Next State.vi"("error in (no error)"=w1564, "New_State"=u32 2, "State Machine in"=w1565) -> ("error out"=w1563:errorcluster, "State Machine out"=w1562:refnum<class "State Machine.lvclass">)  [unwired: 7 in]
        n786 = call "Write Current State Machine.vi"("error in (no error)"=w1563, "State Machine.lvclass"=w1562, "Channel Manager in"=w1561) -> ("error out"=w1580:errorcluster, "Channel Manager out"=w1539:refnum<class "Channel Manager.lvclass">)  [unwired: 7 in]
        n787 = call-dynamic "Write Channel Manager.lvclass.vi"("error in (no error)"=w1580, "Channel Manager.lvclass"=w1539, "SPARC4_AC in"=w1585) -> ("error out"=w1581:errorcluster, "SPARC4_AC out"=w1582:refnum<class "SPARC4_AC.lvclass">)  [unwired: 7 in]
      }
      event "Stop Acq 5": Value Change {
        n788 = event-data() -> ()  [unwired: 1 in, 1 out]
        n789 = call-dynamic "Read Channel Manager.lvclass.vi"("error in (no error)"=w1606, "SPARC4_AC in"=w1607) -> ("error out"=w1587:errorcluster, "Channel Manager.lvclass"=w1588:refnum<class "Channel Manager.lvclass">, "SPARC4_AC out"=w1608:refnum<class "SPARC4_AC.lvclass">)  [unwired: 7 in]
        n790 = call-dynamic "Write Current Camera.vi"("error in (no error)"=w1587, "Current Camera"=3, "Channel Manager in"=w1588) -> ("error out"=w1591:errorcluster, "Channel Manager out"=w1590:refnum<class "Channel Manager.lvclass">)  [unwired: 7 in]
        n791 = call "Return Current RxTx.vi"("error in (no error)"=w1591, "Channel Manager in"=w1590) -> ("error out"=w1596:errorcluster, "RxTx"=w1597:refnum<class "RxTx.lvclass">, "Channel Manager out"=w1593:refnum<class "Channel Manager.lvclass">)  [unwired: 7 in]
        n792 = call-dynamic "Read Interface.lvclass.vi"("error in (no error)"=w1596, "RxTx in"=w1597) -> ("error out"=w1601:errorcluster, "Interface.lvclass"=w1602:refnum<class "Interface.lvclass">, "RxTx out"=w1598:refnum<class "RxTx.lvclass">)  [unwired: 7 in]
        n793 = call-dynamic "Write Stop Acq.vi"("error in (no error)"=w1601, "Stop Acq"="Stop Acq 5", "Interface in"=w1602) -> ("error out"=w1600:errorcluster, "Interface out"=w1599:refnum<class "Interface.lvclass">)  [unwired: 7 in]
        n794 = call-dynamic "Write Interface.lvclass.vi"("error in (no error)"=w1600, "Interface.lvclass"=w1599, "RxTx in"=w1598) -> ("error out"=w1594:errorcluster, "RxTx out"=w1595:refnum<class "RxTx.lvclass">)  [unwired: 7 in]
        n795 = call "Write Current RxTx.vi"("error in (no error)"=w1594, "RxTx"=w1595, "Channel Manager in"=w1593) -> ("error out"=w1603:errorcluster, "Channel Manager out"=w1589:refnum<class "Channel Manager.lvclass">)  [unwired: 7 in]
        n796 = call-dynamic "Write Channel Manager.lvclass.vi"("error in (no error)"=w1603, "Channel Manager.lvclass"=w1589, "SPARC4_AC in"=w1608) -> ("error out"=w1604:errorcluster, "SPARC4_AC out"=w1605:refnum<class "SPARC4_AC.lvclass">)  [unwired: 7 in]
      }
      event "Pausar 5": Value Change {
        n797 = event-data() -> ()  [unwired: 1 in, 1 out]
        n798 = call-dynamic "Read Channel Manager.lvclass.vi"("error in (no error)"=w1630, "SPARC4_AC in"=w1629) -> ("error out"=w1610:errorcluster, "Channel Manager.lvclass"=w1609:refnum<class "Channel Manager.lvclass">, "SPARC4_AC out"=w1631:refnum<class "SPARC4_AC.lvclass">)  [unwired: 7 in]
        n799 = call-dynamic "Write Current Camera.vi"("error in (no error)"=w1610, "Current Camera"=3, "Channel Manager in"=w1609) -> ("error out"=w1612:errorcluster, "Channel Manager out"=w1613:refnum<class "Channel Manager.lvclass">)  [unwired: 7 in]
        n800 = call "Return Current RxTx.vi"("error in (no error)"=w1612, "Channel Manager in"=w1613) -> ("error out"=w1623:errorcluster, "RxTx"=w1624:refnum<class "RxTx.lvclass">, "Channel Manager out"=w1620:refnum<class "Channel Manager.lvclass">)  [unwired: 7 in]
        n801 = call-dynamic "Read Interface.lvclass.vi"("error in (no error)"=w1623, "RxTx in"=w1624) -> ("error out"=w1616:errorcluster, "Interface.lvclass"=w1619:refnum<class "Interface.lvclass">, "RxTx out"=w1625:refnum<class "RxTx.lvclass">)  [unwired: 7 in]
        n802 = call-dynamic "Write Pause Acq.vi"("error in (no error)"=w1616, "Pause Acq"="Pausar 5", "Interface in"=w1619) -> ("error out"=w1617:errorcluster, "Interface out"=w1618:refnum<class "Interface.lvclass">)  [unwired: 7 in]
        n803 = call-dynamic "Write Interface.lvclass.vi"("error in (no error)"=w1617, "Interface.lvclass"=w1618, "RxTx in"=w1625) -> ("error out"=w1621:errorcluster, "RxTx out"=w1622:refnum<class "RxTx.lvclass">)  [unwired: 7 in]
        n804 = call "Write Current RxTx.vi"("error in (no error)"=w1621, "RxTx"=w1622, "Channel Manager in"=w1620) -> ("error out"=w1626:errorcluster, "Channel Manager out"=w1614:refnum<class "Channel Manager.lvclass">)  [unwired: 7 in]
        n805 = call-dynamic "Write Channel Manager.lvclass.vi"("error in (no error)"=w1626, "Channel Manager.lvclass"=w1614, "SPARC4_AC in"=w1631) -> ("error out"=w1627:errorcluster, "SPARC4_AC out"=w1628:refnum<class "SPARC4_AC.lvclass">)  [unwired: 7 in]
      }
      event "Abort 5": Value Change {
        n806 = event-data() -> ()  [unwired: 1 in, 1 out]
        n807 = call-dynamic "Read Channel Manager.lvclass.vi"("error in (no error)"=w1652, "SPARC4_AC in"=w1653) -> ("error out"=w1633:errorcluster, "Channel Manager.lvclass"=w1632:refnum<class "Channel Manager.lvclass">, "SPARC4_AC out"=w1654:refnum<class "SPARC4_AC.lvclass">)  [unwired: 7 in]
        n808 = call-dynamic "Write Current Camera.vi"("error in (no error)"=w1633, "Current Camera"=3, "Channel Manager in"=w1632) -> ("error out"=w1636:errorcluster, "Channel Manager out"=w1635:refnum<class "Channel Manager.lvclass">)  [unwired: 7 in]
        n809 = call "Return Current RxTx.vi"("error in (no error)"=w1636, "Channel Manager in"=w1635) -> ("error out"=w1646:errorcluster, "RxTx"=w1647:refnum<class "RxTx.lvclass">, "Channel Manager out"=w1643:refnum<class "Channel Manager.lvclass">)  [unwired: 7 in]
        n810 = call-dynamic "Read Interface.lvclass.vi"("error in (no error)"=w1646, "RxTx in"=w1647) -> ("error out"=w1640:errorcluster, "Interface.lvclass"=w1641:refnum<class "Interface.lvclass">, "RxTx out"=w1648:refnum<class "RxTx.lvclass">)  [unwired: 7 in]
        n811 = call-dynamic "Write Abort.vi"("error in (no error)"=w1640, "Abort"="Abort 5", "Interface in"=w1641) -> ("error out"=w1639:errorcluster, "Interface out"=w1642:refnum<class "Interface.lvclass">)  [unwired: 7 in]
        n812 = call-dynamic "Write Interface.lvclass.vi"("error in (no error)"=w1639, "Interface.lvclass"=w1642, "RxTx in"=w1648) -> ("error out"=w1644:errorcluster, "RxTx out"=w1645:refnum<class "RxTx.lvclass">)  [unwired: 7 in]
        n813 = call "Write Current RxTx.vi"("error in (no error)"=w1644, "RxTx"=w1645, "Channel Manager in"=w1643) -> ("error out"=w1649:errorcluster, "Channel Manager out"=w1637:refnum<class "Channel Manager.lvclass">)  [unwired: 7 in]
        n814 = call-dynamic "Write Channel Manager.lvclass.vi"("error in (no error)"=w1649, "Channel Manager.lvclass"=w1637, "SPARC4_AC in"=w1654) -> ("error out"=w1650:errorcluster, "SPARC4_AC out"=w1651:refnum<class "SPARC4_AC.lvclass">)  [unwired: 7 in]
      }
      event "Cooler ON/OFF 4": Value Change {
        n815 = event-data() -> ()  [unwired: 1 in, 1 out]
        n816 = call-dynamic "Read Channel Manager.lvclass.vi"("error in (no error)"=w1682, "SPARC4_AC in"=w1683) -> ("error out"=w1657:errorcluster, "Channel Manager.lvclass"=w1658:refnum<class "Channel Manager.lvclass">, "SPARC4_AC out"=w1684:refnum<class "SPARC4_AC.lvclass">)  [unwired: 7 in]
        n817 = call-dynamic "Write Current Camera.vi"("error in (no error)"=w1657, "Current Camera"=3, "Channel Manager in"=w1658) -> ("error out"=w1660:errorcluster, "Channel Manager out"=w1659:refnum<class "Channel Manager.lvclass">)  [unwired: 7 in]
        n818 = local read "Camera Setup"() -> (w1661:T1)
        n819 = Bundle By Name(cluster=w1661, "Cooler ON/OFF"="Cooler ON/OFF 4") -> (w1663:T1)
        n820 = case shown="0, Default" "Cooler ON/OFF 4" {
          tunnel: ["TURN COOLER OFF" "TURN COOLER ON"] -> w1672
          frame 0, Default {
          }
          frame 1 {
          }
        }
        n821 = call "Return Current RxTx.vi"("error in (no error)"=w1660, "Channel Manager in"=w1659) -> ("error out"=w1664:errorcluster, "RxTx"=w1665:refnum<class "RxTx.lvclass">, "Channel Manager out"=w1668:refnum<class "Channel Manager.lvclass">)  [unwired: 7 in]
        n822 = call-dynamic "Read Interface.lvclass.vi"("error in (no error)"=w1664, "RxTx in"=w1665) -> ("error out"=w1677:errorcluster, "Interface.lvclass"=w1678:refnum<class "Interface.lvclass">, "RxTx out"=w1669:refnum<class "RxTx.lvclass">)  [unwired: 7 in]
        n823 = call "Write Camera Setup.vi"("error in (no error)"=w1677, "Camera Setup"=w1663, "Interface in"=w1678) -> ("error out"=w1670:errorcluster, "Interface out"=w1671:refnum<class "Interface.lvclass">)  [unwired: 7 in]
        n824 = call "Write Command.vi"("error in (no error)"=w1670, "Command"=w1672, "Interface in"=w1671) -> ("error out"=w1674:errorcluster, "Interface out"=w1673:refnum<class "Interface.lvclass">)  [unwired: 7 in]
        n825 = call-dynamic "Write Interface.lvclass.vi"("error in (no error)"=w1674, "Interface.lvclass"=w1673, "RxTx in"=w1669) -> ("error out"=w1676:errorcluster, "RxTx out"=w1675:refnum<class "RxTx.lvclass">)  [unwired: 7 in]
        n826 = call "Enqeue A Message.vi"("error in (no error)"=w1676, "RxTx in"=w1675) -> ("error out"=w1666:errorcluster, "RxTx out"=w1667:refnum<class "RxTx.lvclass">)  [unwired: 8 in]
        n827 = call "Write Current RxTx.vi"("error in (no error)"=w1666, "RxTx"=w1667, "Channel Manager in"=w1668) -> ("error out"=w1679:errorcluster, "Channel Manager out"=w1656:refnum<class "Channel Manager.lvclass">)  [unwired: 7 in]
        n828 = call-dynamic "Write Channel Manager.lvclass.vi"("error in (no error)"=w1679, "Channel Manager.lvclass"=w1656, "SPARC4_AC in"=w1684) -> ("error out"=w1680:errorcluster, "SPARC4_AC out"=w1681:refnum<class "SPARC4_AC.lvclass">)  [unwired: 7 in]
      }
      event "Set temperature 4": Value Change {
        n829 = event-data() -> ()  [unwired: 1 in, 1 out]
        n830 = call-dynamic "Read Channel Manager.lvclass.vi"("error in (no error)"=w1714, "SPARC4_AC in"=w1715) -> ("error out"=w1689:errorcluster, "Channel Manager.lvclass"=w1690:refnum<class "Channel Manager.lvclass">, "SPARC4_AC out"=w1716:refnum<class "SPARC4_AC.lvclass">)  [unwired: 7 in]
        n831 = call-dynamic "Write Current Camera.vi"("error in (no error)"=w1689, "Current Camera"=3, "Channel Manager in"=w1690) -> ("error out"=w1692:errorcluster, "Channel Manager out"=w1691:refnum<class "Channel Manager.lvclass">)  [unwired: 7 in]
        n832 = call "Return Current RxTx.vi"("error in (no error)"=w1692, "Channel Manager in"=w1691) -> ("error out"=w1695:errorcluster, "RxTx"=w1698:refnum<class "RxTx.lvclass">, "Channel Manager out"=w1699:refnum<class "Channel Manager.lvclass">)  [unwired: 7 in]
        n833 = call-dynamic "Read Interface.lvclass.vi"("error in (no error)"=w1695, "RxTx in"=w1698) -> ("error out"=w1704:errorcluster, "Interface.lvclass"=w1703:refnum<class "Interface.lvclass">, "RxTx out"=w1710:refnum<class "RxTx.lvclass">)  [unwired: 7 in]
        n834 = local read "Camera Setup"() -> (w1693:T1)
        n835 = Bundle By Name(cluster=w1693, "Set temperature"="Set temperature 4") -> (w1702:T1)
        n836 = call "Write Camera Setup.vi"("error in (no error)"=w1704, "Camera Setup"=w1702, "Interface in"=w1703) -> ("error out"=w1701:errorcluster, "Interface out"=w1700:refnum<class "Interface.lvclass">)  [unwired: 7 in]
        n837 = call "Write Command.vi"("error in (no error)"=w1701, "Command"="SET TEMPERATURE", "Interface in"=w1700) -> ("error out"=w1708:errorcluster, "Interface out"=w1709:refnum<class "Interface.lvclass">)  [unwired: 7 in]
        n838 = call-dynamic "Write Interface.lvclass.vi"("error in (no error)"=w1708, "Interface.lvclass"=w1709, "RxTx in"=w1710) -> ("error out"=w1706:errorcluster, "RxTx out"=w1707:refnum<class "RxTx.lvclass">)  [unwired: 7 in]
        n839 = call "Enqeue A Message.vi"("error in (no error)"=w1706, "RxTx in"=w1707) -> ("error out"=w1696:errorcluster, "RxTx out"=w1697:refnum<class "RxTx.lvclass">)  [unwired: 8 in]
        n840 = call "Write Current RxTx.vi"("error in (no error)"=w1696, "RxTx"=w1697, "Channel Manager in"=w1699) -> ("error out"=w1711:errorcluster, "Channel Manager out"=w1688:refnum<class "Channel Manager.lvclass">)  [unwired: 7 in]
        n841 = call-dynamic "Write Channel Manager.lvclass.vi"("error in (no error)"=w1711, "Channel Manager.lvclass"=w1688, "SPARC4_AC in"=w1716) -> ("error out"=w1712:errorcluster, "SPARC4_AC out"=w1713:refnum<class "SPARC4_AC.lvclass">)  [unwired: 7 in]
        "Temperature ºC 4" <- "Set temperature 4"
      }
      event "Exposure Time 6": Value Change {
        n842 = event-data() -> ()  [unwired: 1 in, 1 out]
        n843 = local write "Exposure Time 8"("Exposure Time 6") -> ()
      }
      event "# Images 4": Value Change {
        n844 = event-data() -> ()  [unwired: 1 in, 1 out]
        n845 = local read "# Images 4"() -> (w1722:u32)
        n846 = property on="Exposições realizadas 4" class="Slide (strict)"("Scale.Maximum"=w1722) -> ()  [unwired: 2 in, 2 out]
      }
      event "Exposure Time 8": Value Change {
        n847 = event-data() -> ()  [unwired: 1 in, 1 out]
        n848 = local read "Exposure Time 8"() -> (w1725:dbl)
        n849 = local write "Exposure Time 6"(w1725) -> ()
      }
      event "Sub Image 4": Value Change {
        n850 = event-data() -> ()  [unwired: 1 in, 1 out]
        n851 = call-dynamic "Read Channel Manager.lvclass.vi"("error in (no error)"=w1740, "SPARC4_AC in"=w1739) -> ("error out"=w1728:errorcluster, "Channel Manager.lvclass"=w1729:refnum<class "Channel Manager.lvclass">, "SPARC4_AC out"=w1745:refnum<class "SPARC4_AC.lvclass">)  [unwired: 7 in]
        n852 = call-dynamic "Write Current Camera.vi"("error in (no error)"=w1728, "Current Camera"=3, "Channel Manager in"=w1729) -> ("error out"=w1731:errorcluster, "Channel Manager out"=w1730:refnum<class "Channel Manager.lvclass">)  [unwired: 7 in]
        n853 = call "Return Current RxTx.vi"("error in (no error)"=w1731, "Channel Manager in"=w1730) -> ("error out"=w1757:errorcluster, "RxTx"=w1758:refnum<class "RxTx.lvclass">, "Channel Manager out"=w1726:refnum<class "Channel Manager.lvclass">)  [unwired: 7 in]
        n854 = call-dynamic "Read Interface.lvclass.vi"("error in (no error)"=w1757, "RxTx in"=w1758) -> ("error out"=w1755:errorcluster, "Interface.lvclass"=w1756:refnum<class "Interface.lvclass">)  [unwired: 7 in, 1 out]
        n855 = call "Read Camera Status.vi"("error in (no error)"=w1755, "Interface in"=w1756) -> ("error out"=w1746:errorcluster, "Camera Status"=w1754:T6)  [unwired: 7 in, 1 out]
        n856 = Unbundle By Name(w1754) -> ("Final Column"=w1751:u16, "Final Line"=w1750:u16)
        n857 = call-dynamic "Write Channel Manager.lvclass.vi"("error in (no error)"=w1746, "Channel Manager.lvclass"=w1726, "SPARC4_AC in"=w1745) -> ("error out"=w1744:errorcluster, "SPARC4_AC out"=w1743:refnum<class "SPARC4_AC.lvclass">)  [unwired: 7 in]
        n858 = case shown="\"256 x 256\"" "Sub Image 4" {
          tunnel: [128 256 512 512] -> w1749
          frame "256 x 256" {
          }
          frame "512 x 512" {
          }
          frame "1024 x 1024", Default {
          }
          frame "Custom" {
          }
        }
        n859 = case shown="\"1024 x 1024\", Default" "Sub Image 4" {
          tunnel: [T7."Disabled and Grayed Out" ("Disabled") T7."Enabled" ("Disabled")] -> w1736
          frame "1024 x 1024", Default {
          }
          frame "Custom" {
          }
        }
        n860 = Divide(x=w1751, y=2) -> (x/y=w1752:dbl)
        n861 = Divide(x=w1750, y=2) -> (x/y=w1753:dbl)
        n862 = Add(x=w1752, y=w1749) -> (x+y=w1735:dbl)
        n863 = Subtract(x=w1752, y=w1749) -> (x-y=w1748:dbl)
        n864 = Subtract(x=w1753, y=w1749) -> (x-y=w1747:dbl)
        n865 = Add(x=w1753, y=w1749) -> (x+y=w1732:dbl)
        n866 = Increment(x=w1748) -> (x+1=w1734:dbl)
        n867 = Increment(x=w1747) -> (x+1=w1733:dbl)
        n868 = local write "Initial Line 4"(w1735) -> ()
        n869 = local write "Initial Cloumn 4"(w1734) -> ()
        n870 = local write "Final Line 4"(w1733) -> ()
        n871 = local write "Final Column 4"(w1732) -> ()
        n872 = property on="Initial Line 4" class="DigNum (strict)"("DisabledEnum"=w1736) -> ()  [unwired: 2 in, 2 out]
        n873 = property on="Initial Cloumn 4" class="DigNum (strict)"("DisabledEnum"=w1736) -> ()  [unwired: 2 in, 2 out]
        n874 = property on="Final Line 4" class="DigNum (strict)"("DisabledEnum"=w1736) -> ()  [unwired: 2 in, 2 out]
        n875 = property on="Final Column 4" class="DigNum (strict)"("DisabledEnum"=w1736) -> ()  [unwired: 2 in, 2 out]
        n876 = flat-sequence {
          tunnel: w1744 -> [w1770]
          tunnel: w1743 -> [w1771]
          tunnel: [w1771] -> w1738
          tunnel: [w1770] -> w1737
          frame #0 {
            w1764 = cluster{dbl, dbl} {0.0, 0.0}
            n877 = local read "Initial Cloumn 4"() -> (w1763:u16)
            n878 = local read "Final Column 4"() -> (w1761:u16)
            n879 = local read "Initial Line 4"() -> (w1762:u16)
            n880 = local read "Final Line 4"() -> (w1760:u16)
            n881 = Bundle(cluster=w1764, w1763, w1762) -> (w1769:cluster{dbl, dbl})
            n882 = Bundle(cluster=w1764, w1763, w1760) -> (w1768:cluster{dbl, dbl})
            n883 = Bundle(cluster=w1764, w1761, w1760) -> (w1767:cluster{dbl, dbl})
            n884 = Bundle(cluster=w1764, w1761, w1762) -> (w1766:cluster{dbl, dbl})
            n885 = Bundle(cluster=w1764, w1763, w1762) -> (w1765:cluster{dbl, dbl})
            n886 = Build Array(w1769, w1768, w1767, w1766, w1765) -> ()  [unwired: 1 out]
          }
        }
      }
      event "Final Line 4", "Final Column 4", "Initial Cloumn 4", "Initial Line 4": Value Change {
        n887 = event-data() -> ()  [unwired: 1 in, 1 out]
        n888 = disable-structure shown="Disabled" {
          frame Disabled {
            w1780 = cluster{dbl, dbl} {0.0, 0.0}
            n889 = local read "Initial Cloumn 4"() -> (w1784:u16)
            n890 = local read "Final Column 4"() -> (w1782:u16)
            n891 = local read "Initial Line 4"() -> (w1783:u16)
            n892 = local read "Final Line 4"() -> (w1781:u16)
            n893 = Bundle(cluster=w1780, w1784, w1783) -> (w1789:cluster{dbl, dbl})
            n894 = Bundle(cluster=w1780, w1784, w1781) -> (w1788:cluster{dbl, dbl})
            n895 = Bundle(cluster=w1780, w1782, w1781) -> (w1787:cluster{dbl, dbl})
            n896 = Bundle(cluster=w1780, w1782, w1783) -> (w1786:cluster{dbl, dbl})
            n897 = Bundle(cluster=w1780, w1784, w1783) -> (w1785:cluster{dbl, dbl})
            n898 = Build Array(w1789, w1788, w1787, w1786, w1785) -> ()  [unwired: 1 out]
          }
          frame Enabled {
          }
        }
      }
      event "Load Setup": Value Change {
        n899 = event-data() -> ()  [unwired: 1 in, 1 out]
        n900 = call-dynamic "Read Setup File.lvclass.vi"("error in (no error)"=w1806, "SPARC4_AC in"=w1807) -> ("error out"=w1804:errorcluster, "Setup File.lvclass"=w1803:refnum<class "Setup File.lvclass">, "SPARC4_AC out"=w1794:refnum<class "SPARC4_AC.lvclass">)  [unwired: 7 in]
        n901 = call "File Dialog"() -> ("selected path"=w1805:path, "error out"=w1799:errorcluster)  [unwired: 12 in, 2 out]
        n902 = call <vilib>:"Clear Errors.vi"("error in (no error)"=w1799) -> ()  [unwired: 5 in, 2 out]
        n903 = call "Select File.vi"("error in (no error)"=w1804, "File Path Control"=w1805, "Setup File in"=w1803) -> ("error out"=w1802:errorcluster, "Setup File out"=w1801:refnum<class "Setup File.lvclass">)  [unwired: 7 in]
        n904 = call "Read File Path.vi"("error in (no error)"=w1802, "Setup File in"=w1801) -> ("error out"=w1798:errorcluster, "File Path"=→"Setup File Path:":string, "Setup File out"=w1797:refnum<class "Setup File.lvclass">)  [unwired: 7 in]
        n905 = call "Read File.vi"("error in (no error)"=w1798, "Setup File in"=w1797) -> ("error out"=w1796:errorcluster, "CHANNELS"=w1790:i32[], "Array"=w1791:string[][], "Setup File out"=w1795:refnum<class "Setup File.lvclass">)  [unwired: 6 in]
        n906 = call-dynamic "Write Setup File.lvclass.vi"("error in (no error)"=w1796, "Setup File.lvclass"=w1795, "SPARC4_AC in"=w1794) -> ("error out"=w1793:errorcluster, "SPARC4_AC out"=w1792:refnum<class "SPARC4_AC.lvclass">)  [unwired: 7 in]
        n907 = for {
          tunnel: w1791 -> [w1809]
          tunnel: w1790 -> [w1808] mode=indexing
          n908 = case shown="4" w1808 {
            tunnel: w1809 -> [w1810 w1888 w1966 w2044]
            frame 1, Default {
              n909 = for {
                tunnel: w1810 -> [w1815] mode=indexing
                n910 = Index Array(array=w1815, index #1=0 ("index"), index #2=1 ("index")) -> (element #1=w1812:string, element #2=w1811:string)
                n911 = case shown="\"SUBIMAGE\"" w1812 {
                  tunnel: w1811 -> [_ w1816 w1824 w1831 w1835 w1838 w1850 w1852 w1858 w1862 w1872 _ w1880 w1887]
                  frame "False", Default {
                  }
                  frame "EXPOSURETIME" {
                    n912 = Not Equal?(x="", y=w1816) -> (x != y?=w1818:bool)
                    n913 = case shown="True" w1818 {
                      tunnel: w1816 -> [_ w1823]
                      frame False {
                      }
                      frame True {
                        n914 = Fract/Exp String To Number(string=w1823) -> (number=w1820:dbl)  [unwired: 3 in, 1 out]
                        n915 = In Range and Coerce(upper limit=inf, x=w1820, lower limit=0.0 ("y")) -> (coerced(x)=w1819:dbl)  [unwired: 1 out]
                        n916 = local write "Exposure Time"(w1819) -> ()
                        n917 = local write "Exposure Time 2"(w1819) -> ()
                      }
                    }
                  }
                  frame "READOUTRATE" {
                    n918 = case shown="\"1MHz\", Default" w1824 {
                      tunnel: [w1826 w1827 w1828 w1829] -> w1825
                      frame "1MHz", Default {
                        w1826 = u8 0 items=["1 MHz", "10 MHz", "20 MHz", "30 MHz"] ("Readout Rate")
                      }
                      frame "10MHz" {
                        w1827 = u8 1 items=["1 MHz", "10 MHz", "20 MHz", "30 MHz"] ("Readout Rate")
                      }
                      frame "20MHz" {
                        w1828 = u8 2 items=["1 MHz", "10 MHz", "20 MHz", "30 MHz"] ("Readout Rate")
                      }
                      frame "30MHz" {
                        w1829 = u8 3 items=["1 MHz", "10 MHz", "20 MHz", "30 MHz"] ("Readout Rate")
                      }
                    }
                    n919 = local write "Readout Rate"(w1825) -> ()
                  }
                  frame "PREAMP" {
                    n920 = case shown="\"GAIN2\"" w1831 {
                      tunnel: [w1832 w1833] -> w1830
                      frame "GAIN1", Default {
                        w1832 = u8 0 items=["Gain 1", "Gain 2"] ("Pre-amp gain")
                      }
                      frame "GAIN2" {
                        w1833 = u8 1 items=["Gain 1", "Gain 2"] ("Pre-amp gain")
                      }
                    }
                    n921 = local write "Pre-amp gain"(w1830) -> ()
                  }
                  frame "COOLER" {
                    n922 = case shown="\"COOLERON\"" w1835 {
                      tunnel: [w1836 w1837] -> w1834
                      frame "COOLERON" {
                        w1836 = u16 1 items=["Cooler OFF", "Cooler ON"] ("Cooler ON/OFF")
                      }
                      frame "COOLEROFF", Default {
                        w1837 = u16 0 items=["Cooler OFF", "Cooler ON"] ("Cooler ON/OFF")
                      }
                    }
                    n923 = local write "Cooler ON/OFF"(w1834) -> ()
                  }
                  frame "TEMPERATURE" {
                    n924 = Not Equal?(x="", y=w1838) -> (x != y?=w1840:bool)
                    n925 = case shown="True" w1840 {
                      tunnel: w1838 -> [_ w1845]
                      frame False {
                      }
                      frame True {
                        n926 = property on="Set temperature 3" class="DigNum (strict)"() -> ("Maximum"=w1844:dbl)  [unwired: 2 in, 2 out]
                        n927 = property on="Set temperature 3" class="DigNum (strict)"() -> ("Minimum"=w1843:dbl)  [unwired: 2 in, 2 out]
                        n928 = Decimal String To Number(string=w1845) -> (number=w1842:i32)  [unwired: 2 in, 1 out]
                        n929 = In Range and Coerce(upper limit=w1844, x=w1842, lower limit=w1843) -> (coerced(x)=w1841:dbl)  [unwired: 1 out]
                        n930 = local write "Temperature ºC"(w1841) -> ()
                        n931 = local write "Set temperature"(w1841) -> ()
                      }
                    }
                  }
                  frame "INITIALLINE" {
                    n932 = Decimal String To Number(string=w1850) -> (number=w1847:i32)  [unwired: 2 in, 1 out]
                    n933 = call <userlib>:"GetDetector.vi"() -> ("ypixels"=w1849:i32)  [unwired: 4 in, 3 out]
                    n934 = In Range and Coerce(upper limit=w1849, x=w1847, lower limit=1) -> (coerced(x)=w1846:i32)  [unwired: 1 out]
                    n935 = local write "Initial Line"(w1846) -> ()
                  }
                  frame "INITIALCOLUMN" {
                    n936 = Decimal String To Number(string=w1852) -> (number=w1855:i32)  [unwired: 2 in, 1 out]
                    n937 = call <userlib>:"GetDetector.vi"() -> ("xpixels"=w1853:i32)  [unwired: 4 in, 3 out]
                    n938 = In Range and Coerce(upper limit=w1853, x=w1855, lower limit=1) -> (coerced(x)=w1851:i32)  [unwired: 1 out]
                    n939 = local write "Initial Cloumn"(w1851) -> ()
                  }
                  frame "FINALLINE" {
                    n940 = Decimal String To Number(string=w1858) -> (number=w1860:i32)  [unwired: 2 in, 1 out]
                    n941 = call <userlib>:"GetDetector.vi"() -> ("ypixels"=w1856:i32)  [unwired: 4 in, 3 out]
                    n942 = In Range and Coerce(upper limit=w1856, x=w1860, lower limit=1) -> (coerced(x)=w1857:i32)  [unwired: 1 out]
                    n943 = local write "Final Line"(w1857) -> ()
                  }
                  frame "FINALCOLUMN" {
                    n944 = Decimal String To Number(string=w1862) -> (number=w1865:i32)  [unwired: 2 in, 1 out]
                    n945 = call <userlib>:"GetDetector.vi"() -> ("xpixels"=w1864:i32)  [unwired: 4 in, 3 out]
                    n946 = In Range and Coerce(upper limit=w1864, x=w1865, lower limit=1) -> (coerced(x)=w1861:i32)  [unwired: 1 out]
                    n947 = local write "Final Column"(w1861) -> ()
                  }
                  frame "HORIZONTALBINNING" {
                    n948 = Decimal String To Number(string=w1872) -> (number=w1866:i32)  [unwired: 2 in, 1 out]
                    n949 = call <userlib>:"GetDetector.vi"() -> ("xpixels"=w1871:i32)  [unwired: 4 in, 3 out]
                    n950 = Quotient & Remainder(x=w1871, y=w1866) -> (x-y*floor(x/y)=w1870:i32)  [unwired: 1 out]
                    n951 = Equal?(x=0 ("index"), y=w1870) -> (x = y?=w1867:bool)
                    n952 = case shown="True" w1867 {
                      tunnel: "INVALID VALUE FOR HORIZONTAL BINNING" -> [w1874 _]
                      tunnel: w1866 -> [w1873 w1878]
                      frame False {
                        n953 = Number To Decimal String(number=w1873) -> (decimal integer string=w1877:string)  [unwired: 1 in]
                        n954 = Concatenate Strings(w1874, w1877) -> (w1876:string)
                        n955 = One Button Dialog(message=w1876, button name ("OK")="OK") -> ()  [unwired: 1 out]
                      }
                      frame True {
                        n956 = local write "Binning 5"(w1878) -> ()
                      }
                    }
                  }
                  frame "SUBIMAGE" {
                  }
                  frame "EMMODE" {
                    n957 = case shown="\"ELECTRON MULTIPLYING\", Default" w1880 {
                      tunnel: [w1881 w1882] -> w1879
                      frame "ELECTRON MULTIPLYING", Default {
                        w1881 = u8 0 items=["Electron Multiplying", "Conventional"] ("EM Mode")
                      }
                      frame "CONVENTIONAL" {
                        w1882 = u8 1 items=["Electron Multiplying", "Conventional"] ("EM Mode")
                      }
                    }
                    n958 = local write "EM Mode"(w1879) -> ()
                  }
                  frame "EMGAIN" {
                    n959 = Decimal String To Number(string=w1887) -> (number=w1884:i32)  [unwired: 2 in, 1 out]
                    n960 = In Range and Coerce(upper limit=300 ("index"), x=w1884, lower limit=2 ("index")) -> (coerced(x)=w1883:i32)  [unwired: 1 out]
                    n961 = local write "EM Gain"(w1883) -> ()
                  }
                }
              }
            }
            frame 2 {
              n962 = for {
                tunnel: w1888 -> [w1893] mode=indexing
                n963 = Index Array(array=w1893, index #1=0 ("index"), index #2=1 ("index")) -> (element #1=w1890:string, element #2=w1889:string)
                n964 = case shown="\"SUBIMAGE\"" w1890 {
                  tunnel: w1889 -> [_ w1894 w1903 w1909 w1913 w1916 w1928 w1930 w1936 w1940 w1950 _ w1958 w1965]
                  frame "False", Default {
                  }
                  frame "EXPOSURETIME" {
                    n965 = Not Equal?(x="", y=w1894) -> (x != y?=w1896:bool)
                    n966 = case shown="True" w1896 {
                      tunnel: w1894 -> [_ w1901]
                      frame False {
                      }
                      frame True {
                        n967 = Fract/Exp String To Number(string=w1901) -> (number=w1898:dbl)  [unwired: 3 in, 1 out]
                        n968 = In Range and Coerce(upper limit=inf, x=w1898, lower limit=0.0 ("y")) -> (coerced(x)=w1897:dbl)  [unwired: 1 out]
                        n969 = local write "Exposure Time 4"(w1897) -> ()
                        n970 = local write "Exposure Time 3"(w1897) -> ()
                      }
                    }
                  }
                  frame "READOUTRATE" {
                    n971 = case shown="\"1MHz\", Default" w1903 {
                      tunnel: [w1904 w1905 w1906 w1907] -> w1902
                      frame "1MHz", Default {
                        w1904 = u8 0 items=["1 MHz", "10 MHz", "20 MHz", "30 MHz"] ("Readout Rate")
                      }
                      frame "10MHz" {
                        w1905 = u8 1 items=["1 MHz", "10 MHz", "20 MHz", "30 MHz"] ("Readout Rate")
                      }
                      frame "20MHz" {
                        w1906 = u8 2 items=["1 MHz", "10 MHz", "20 MHz", "30 MHz"] ("Readout Rate")
                      }
                      frame "30MHz" {
                        w1907 = u8 3 items=["1 MHz", "10 MHz", "20 MHz", "30 MHz"] ("Readout Rate")
                      }
                    }
                    n972 = local write "Readout Rate 2"(w1902) -> ()
                  }
                  frame "PREAMP" {
                    n973 = case shown="\"GAIN2\"" w1909 {
                      tunnel: [w1910 w1911] -> w1908
                      frame "GAIN1", Default {
                        w1910 = u8 0 items=["Gain 1", "Gain 2"] ("Pre-amp gain")
                      }
                      frame "GAIN2" {
                        w1911 = u8 1 items=["Gain 1", "Gain 2"] ("Pre-amp gain")
                      }
                    }
                    n974 = local write "Pre-amp gain 2"(w1908) -> ()
                  }
                  frame "COOLER" {
                    n975 = case shown="\"COOLERON\"" w1913 {
                      tunnel: [w1914 w1915] -> w1912
                      frame "COOLERON" {
                        w1914 = u16 1 items=["Cooler OFF", "Cooler ON"] ("Cooler ON/OFF")
                      }
                      frame "COOLEROFF", Default {
                        w1915 = u16 0 items=["Cooler OFF", "Cooler ON"] ("Cooler ON/OFF")
                      }
                    }
                    n976 = local write "Cooler ON/OFF 2"(w1912) -> ()
                  }
                  frame "TEMPERATURE" {
                    n977 = Not Equal?(x="", y=w1916) -> (x != y?=w1918:bool)
                    n978 = case shown="True" w1918 {
                      tunnel: w1916 -> [_ w1923]
                      frame False {
                      }
                      frame True {
                        n979 = property on="Set temperature 3" class="DigNum (strict)"() -> ("Maximum"=w1922:dbl)  [unwired: 2 in, 2 out]
                        n980 = property on="Set temperature 3" class="DigNum (strict)"() -> ("Minimum"=w1921:dbl)  [unwired: 2 in, 2 out]
                        n981 = Decimal String To Number(string=w1923) -> (number=w1920:i32)  [unwired: 2 in, 1 out]
                        n982 = In Range and Coerce(upper limit=w1922, x=w1920, lower limit=w1921) -> (coerced(x)=w1919:dbl)  [unwired: 1 out]
                        n983 = local write "Temperature ºC 2"(w1919) -> ()
                        n984 = local write "Set temperature 2"(w1919) -> ()
                      }
                    }
                  }
                  frame "INITIALLINE" {
                    n985 = Decimal String To Number(string=w1928) -> (number=w1925:i32)  [unwired: 2 in, 1 out]
                    n986 = call <userlib>:"GetDetector.vi"() -> ("ypixels"=w1927:i32)  [unwired: 4 in, 3 out]
                    n987 = In Range and Coerce(upper limit=w1927, x=w1925, lower limit=1) -> (coerced(x)=w1924:i32)  [unwired: 1 out]
                    n988 = local write "Initial Line 2"(w1924) -> ()
                  }
                  frame "INITIALCOLUMN" {
                    n989 = Decimal String To Number(string=w1930) -> (number=w1933:i32)  [unwired: 2 in, 1 out]
                    n990 = call <userlib>:"GetDetector.vi"() -> ("xpixels"=w1931:i32)  [unwired: 4 in, 3 out]
                    n991 = In Range and Coerce(upper limit=w1931, x=w1933, lower limit=1) -> (coerced(x)=w1929:i32)  [unwired: 1 out]
                    n992 = local write "Initial Cloumn 2"(w1929) -> ()
                  }
                  frame "FINALLINE" {
                    n993 = Decimal String To Number(string=w1936) -> (number=w1938:i32)  [unwired: 2 in, 1 out]
                    n994 = call <userlib>:"GetDetector.vi"() -> ("ypixels"=w1935:i32)  [unwired: 4 in, 3 out]
                    n995 = In Range and Coerce(upper limit=w1935, x=w1938, lower limit=1) -> (coerced(x)=w1934:i32)  [unwired: 1 out]
                    n996 = local write "Final Line 2"(w1934) -> ()
                  }
                  frame "FINALCOLUMN" {
                    n997 = Decimal String To Number(string=w1940) -> (number=w1943:i32)  [unwired: 2 in, 1 out]
                    n998 = call <userlib>:"GetDetector.vi"() -> ("xpixels"=w1942:i32)  [unwired: 4 in, 3 out]
                    n999 = In Range and Coerce(upper limit=w1942, x=w1943, lower limit=1) -> (coerced(x)=w1939:i32)  [unwired: 1 out]
                    n1000 = local write "Final Column 2"(w1939) -> ()
                  }
                  frame "HORIZONTALBINNING" {
                    n1001 = Decimal String To Number(string=w1950) -> (number=w1944:i32)  [unwired: 2 in, 1 out]
                    n1002 = call <userlib>:"GetDetector.vi"() -> ("xpixels"=w1949:i32)  [unwired: 4 in, 3 out]
                    n1003 = Quotient & Remainder(x=w1949, y=w1944) -> (x-y*floor(x/y)=w1948:i32)  [unwired: 1 out]
                    n1004 = Equal?(x=0 ("index"), y=w1948) -> (x = y?=w1945:bool)
                    n1005 = case shown="True" w1945 {
                      tunnel: "INVALID VALUE FOR HORIZONTAL BINNING" -> [w1952 _]
                      tunnel: w1944 -> [w1951 w1956]
                      frame False {
                        n1006 = Number To Decimal String(number=w1951) -> (decimal integer string=w1955:string)  [unwired: 1 in]
                        n1007 = Concatenate Strings(w1952, w1955) -> (w1954:string)
                        n1008 = One Button Dialog(message=w1954, button name ("OK")="OK") -> ()  [unwired: 1 out]
                      }
                      frame True {
                        n1009 = local write "Binning 6"(w1956) -> ()
                      }
                    }
                  }
                  frame "SUBIMAGE" {
                  }
                  frame "EMMODE" {
                    n1010 = case shown="\"ELECTRON MULTIPLYING\", Default" w1958 {
                      tunnel: [w1959 w1960] -> w1957
                      frame "ELECTRON MULTIPLYING", Default {
                        w1959 = u8 0 items=["Electron Multiplying", "Conventional"] ("EM Mode")
                      }
                      frame "CONVENTIONAL" {
                        w1960 = u8 1 items=["Electron Multiplying", "Conventional"] ("EM Mode")
                      }
                    }
                    n1011 = local write "EM Mode 2"(w1957) -> ()
                  }
                  frame "EMGAIN" {
                    n1012 = Decimal String To Number(string=w1965) -> (number=w1962:i32)  [unwired: 2 in, 1 out]
                    n1013 = In Range and Coerce(upper limit=300 ("index"), x=w1962, lower limit=2 ("index")) -> (coerced(x)=w1961:i32)  [unwired: 1 out]
                    n1014 = local write "EM Gain 2"(w1961) -> ()
                  }
                }
              }
            }
            frame 3 {
              n1015 = for {
                tunnel: w1966 -> [w1971] mode=indexing
                n1016 = Index Array(array=w1971, index #1=0 ("index"), index #2=1 ("index")) -> (element #1=w1968:string, element #2=w1967:string)
                n1017 = case shown="\"FINALCOLUMN\"" w1968 {
                  tunnel: w1967 -> [_ w1972 w1981 w1987 w1991 w1994 w2006 w2008 w2014 w2018 w2028 _ w2036 w2043]
                  frame "False", Default {
                  }
                  frame "EXPOSURETIME" {
                    n1018 = Not Equal?(x="", y=w1972) -> (x != y?=w1974:bool)
                    n1019 = case shown="True" w1974 {
                      tunnel: w1972 -> [_ w1979]
                      frame False {
                      }
                      frame True {
                        n1020 = Fract/Exp String To Number(string=w1979) -> (number=w1976:dbl)  [unwired: 3 in, 1 out]
                        n1021 = In Range and Coerce(upper limit=inf, x=w1976, lower limit=0.0 ("y")) -> (coerced(x)=w1975:dbl)  [unwired: 1 out]
                        n1022 = local write "Exposure Time 7"(w1975) -> ()
                        n1023 = local write "Exposure Time 5"(w1975) -> ()
                      }
                    }
                  }
                  frame "READOUTRATE" {
                    n1024 = case shown="\"1MHz\", Default" w1981 {
                      tunnel: [w1982 w1983 w1984 w1985] -> w1980
                      frame "1MHz", Default {
                        w1982 = u8 0 items=["1 MHz", "10 MHz", "20 MHz", "30 MHz"] ("Readout Rate")
                      }
                      frame "10MHz" {
                        w1983 = u8 1 items=["1 MHz", "10 MHz", "20 MHz", "30 MHz"] ("Readout Rate")
                      }
                      frame "20MHz" {
                        w1984 = u8 2 items=["1 MHz", "10 MHz", "20 MHz", "30 MHz"] ("Readout Rate")
                      }
                      frame "30MHz" {
                        w1985 = u8 3 items=["1 MHz", "10 MHz", "20 MHz", "30 MHz"] ("Readout Rate")
                      }
                    }
                    n1025 = local write "Readout Rate 3"(w1980) -> ()
                  }
                  frame "PREAMP" {
                    n1026 = case shown="\"GAIN2\"" w1987 {
                      tunnel: [w1988 w1989] -> w1986
                      frame "GAIN1", Default {
                        w1988 = u8 0 items=["Gain 1", "Gain 2"] ("Pre-amp gain")
                      }
                      frame "GAIN2" {
                        w1989 = u8 1 items=["Gain 1", "Gain 2"] ("Pre-amp gain")
                      }
                    }
                    n1027 = local write "Pre-amp gain 3"(w1986) -> ()
                  }
                  frame "COOLER" {
                    n1028 = case shown="\"COOLERON\"" w1991 {
                      tunnel: [w1992 w1993] -> w1990
                      frame "COOLERON" {
                        w1992 = u16 1 items=["Cooler OFF", "Cooler ON"] ("Cooler ON/OFF")
                      }
                      frame "COOLEROFF", Default {
                        w1993 = u16 0 items=["Cooler OFF", "Cooler ON"] ("Cooler ON/OFF")
                      }
                    }
                    n1029 = local write "Cooler ON/OFF 3"(w1990) -> ()
                  }
                  frame "TEMPERATURE" {
                    n1030 = Not Equal?(x="", y=w1994) -> (x != y?=w1996:bool)
                    n1031 = case shown="True" w1996 {
                      tunnel: w1994 -> [_ w2001]
                      frame False {
                      }
                      frame True {
                        n1032 = property on="Set temperature 3" class="DigNum (strict)"() -> ("Maximum"=w2000:dbl)  [unwired: 2 in, 2 out]
                        n1033 = property on="Set temperature 3" class="DigNum (strict)"() -> ("Minimum"=w1999:dbl)  [unwired: 2 in, 2 out]
                        n1034 = Decimal String To Number(string=w2001) -> (number=w1998:i32)  [unwired: 2 in, 1 out]
                        n1035 = In Range and Coerce(upper limit=w2000, x=w1998, lower limit=w1999) -> (coerced(x)=w1997:dbl)  [unwired: 1 out]
                        n1036 = local write "Set temperature 3"(w1997) -> ()
                        n1037 = local write "Temperature ºC 3"(w1997) -> ()
                      }
                    }
                  }
                  frame "INITIALLINE" {
                    n1038 = Decimal String To Number(string=w2006) -> (number=w2003:i32)  [unwired: 2 in, 1 out]
                    n1039 = call <userlib>:"GetDetector.vi"() -> ("ypixels"=w2005:i32)  [unwired: 4 in, 3 out]
                    n1040 = In Range and Coerce(upper limit=w2005, x=w2003, lower limit=1) -> (coerced(x)=w2002:i32)  [unwired: 1 out]
                    n1041 = local write "Initial Line 3"(w2002) -> ()
                  }
                  frame "INITIALCOLUMN" {
                    n1042 = Decimal String To Number(string=w2008) -> (number=w2011:i32)  [unwired: 2 in, 1 out]
                    n1043 = call <userlib>:"GetDetector.vi"() -> ("xpixels"=w2009:i32)  [unwired: 4 in, 3 out]
                    n1044 = In Range and Coerce(upper limit=w2009, x=w2011, lower limit=1) -> (coerced(x)=w2007:i32)  [unwired: 1 out]
                    n1045 = local write "Initial Cloumn 3"(w2007) -> ()
                  }
                  frame "FINALLINE" {
                    n1046 = Decimal String To Number(string=w2014) -> (number=w2016:i32)  [unwired: 2 in, 1 out]
                    n1047 = call <userlib>:"GetDetector.vi"() -> ("ypixels"=w2013:i32)  [unwired: 4 in, 3 out]
                    n1048 = In Range and Coerce(upper limit=w2013, x=w2016, lower limit=1) -> (coerced(x)=w2012:i32)  [unwired: 1 out]
                    n1049 = local write "Final Line 3"(w2012) -> ()
                  }
                  frame "FINALCOLUMN" {
                    n1050 = Decimal String To Number(string=w2018) -> (number=w2021:i32)  [unwired: 2 in, 1 out]
                    n1051 = call <userlib>:"GetDetector.vi"() -> ("xpixels"=w2020:i32)  [unwired: 4 in, 3 out]
                    n1052 = In Range and Coerce(upper limit=w2020, x=w2021, lower limit=1) -> (coerced(x)=w2017:i32)  [unwired: 1 out]
                    n1053 = local write "Final Column 3"(w2017) -> ()
                  }
                  frame "HORIZONTALBINNING" {
                    n1054 = Decimal String To Number(string=w2028) -> (number=w2022:i32)  [unwired: 2 in, 1 out]
                    n1055 = call <userlib>:"GetDetector.vi"() -> ("xpixels"=w2027:i32)  [unwired: 4 in, 3 out]
                    n1056 = Quotient & Remainder(x=w2027, y=w2022) -> (x-y*floor(x/y)=w2026:i32)  [unwired: 1 out]
                    n1057 = Equal?(x=0 ("index"), y=w2026) -> (x = y?=w2023:bool)
                    n1058 = case shown="True" w2023 {
                      tunnel: "INVALID VALUE FOR HORIZONTAL BINNING" -> [w2030 _]
                      tunnel: w2022 -> [w2029 w2034]
                      frame False {
                        n1059 = Number To Decimal String(number=w2029) -> (decimal integer string=w2033:string)  [unwired: 1 in]
                        n1060 = Concatenate Strings(w2030, w2033) -> (w2032:string)
                        n1061 = One Button Dialog(message=w2032, button name ("OK")="OK") -> ()  [unwired: 1 out]
                      }
                      frame True {
                        n1062 = local write "Binning 7"(w2034) -> ()
                      }
                    }
                  }
                  frame "SUBIMAGE" {
                  }
                  frame "EMMODE" {
                    n1063 = case shown="\"ELECTRON MULTIPLYING\", Default" w2036 {
                      tunnel: [w2037 w2038] -> w2035
                      frame "ELECTRON MULTIPLYING", Default {
                        w2037 = u8 0 items=["Electron Multiplying", "Conventional"] ("EM Mode")
                      }
                      frame "CONVENTIONAL" {
                        w2038 = u8 1 items=["Electron Multiplying", "Conventional"] ("EM Mode")
                      }
                    }
                    n1064 = local write "EM Mode 3"(w2035) -> ()
                  }
                  frame "EMGAIN" {
                    n1065 = Decimal String To Number(string=w2043) -> (number=w2040:i32)  [unwired: 2 in, 1 out]
                    n1066 = In Range and Coerce(upper limit=300 ("index"), x=w2040, lower limit=2 ("index")) -> (coerced(x)=w2039:i32)  [unwired: 1 out]
                    n1067 = local write "EM Gain 3"(w2039) -> ()
                  }
                }
              }
            }
            frame 4 {
              n1068 = for {
                tunnel: w2044 -> [w2049] mode=indexing
                n1069 = Index Array(array=w2049, index #1=0 ("index"), index #2=1 ("index")) -> (element #1=w2046:string, element #2=w2045:string)
                n1070 = case shown="\"SUBIMAGE\"" w2046 {
                  tunnel: w2045 -> [_ w2050 w2059 w2065 w2069 w2072 w2084 w2086 w2092 w2096 w2106 _ w2114 w2121]
                  frame "False", Default {
                  }
                  frame "EXPOSURETIME" {
                    n1071 = Not Equal?(x="", y=w2050) -> (x != y?=w2052:bool)
                    n1072 = case shown="True" w2052 {
                      tunnel: w2050 -> [_ w2057]
                      frame False {
                      }
                      frame True {
                        n1073 = Fract/Exp String To Number(string=w2057) -> (number=w2054:dbl)  [unwired: 3 in, 1 out]
                        n1074 = In Range and Coerce(upper limit=inf, x=w2054, lower limit=0.0 ("y")) -> (coerced(x)=w2053:dbl)  [unwired: 1 out]
                        n1075 = local write "Exposure Time 8"(w2053) -> ()
                        n1076 = local write "Exposure Time 6"(w2053) -> ()
                      }
                    }
                  }
                  frame "READOUTRATE" {
                    n1077 = case shown="\"1MHz\", Default" w2059 {
                      tunnel: [w2060 w2061 w2062 w2063] -> w2058
                      frame "1MHz", Default {
                        w2060 = u8 0 items=["1 MHz", "10 MHz", "20 MHz", "30 MHz"] ("Readout Rate")
                      }
                      frame "10MHz" {
                        w2061 = u8 1 items=["1 MHz", "10 MHz", "20 MHz", "30 MHz"] ("Readout Rate")
                      }
                      frame "20MHz" {
                        w2062 = u8 2 items=["1 MHz", "10 MHz", "20 MHz", "30 MHz"] ("Readout Rate")
                      }
                      frame "30MHz" {
                        w2063 = u8 3 items=["1 MHz", "10 MHz", "20 MHz", "30 MHz"] ("Readout Rate")
                      }
                    }
                    n1078 = local write "Readout Rate 4"(w2058) -> ()
                  }
                  frame "PREAMP" {
                    n1079 = case shown="\"GAIN2\"" w2065 {
                      tunnel: [w2066 w2067] -> w2064
                      frame "GAIN1", Default {
                        w2066 = u8 0 items=["Gain 1", "Gain 2"] ("Pre-amp gain")
                      }
                      frame "GAIN2" {
                        w2067 = u8 1 items=["Gain 1", "Gain 2"] ("Pre-amp gain")
                      }
                    }
                    n1080 = local write "Pre-amp gain 4"(w2064) -> ()
                  }
                  frame "COOLER" {
                    n1081 = case shown="\"COOLERON\"" w2069 {
                      tunnel: [w2070 w2071] -> w2068
                      frame "COOLERON" {
                        w2070 = u16 1 items=["Cooler OFF", "Cooler ON"] ("Cooler ON/OFF")
                      }
                      frame "COOLEROFF", Default {
                        w2071 = u16 0 items=["Cooler OFF", "Cooler ON"] ("Cooler ON/OFF")
                      }
                    }
                    n1082 = local write "Cooler ON/OFF 4"(w2068) -> ()
                  }
                  frame "TEMPERATURE" {
                    n1083 = Not Equal?(x="", y=w2072) -> (x != y?=w2074:bool)
                    n1084 = case shown="True" w2074 {
                      tunnel: w2072 -> [_ w2079]
                      frame False {
                      }
                      frame True {
                        n1085 = property on="Set temperature 3" class="DigNum (strict)"() -> ("Maximum"=w2078:dbl)  [unwired: 2 in, 2 out]
                        n1086 = property on="Set temperature 3" class="DigNum (strict)"() -> ("Minimum"=w2077:dbl)  [unwired: 2 in, 2 out]
                        n1087 = Decimal String To Number(string=w2079) -> (number=w2076:i32)  [unwired: 2 in, 1 out]
                        n1088 = In Range and Coerce(upper limit=w2078, x=w2076, lower limit=w2077) -> (coerced(x)=w2075:dbl)  [unwired: 1 out]
                        n1089 = local write "Set temperature 4"(w2075) -> ()
                        n1090 = local write "Temperature ºC 4"(w2075) -> ()
                      }
                    }
                  }
                  frame "INITIALLINE" {
                    n1091 = Decimal String To Number(string=w2084) -> (number=w2081:i32)  [unwired: 2 in, 1 out]
                    n1092 = call <userlib>:"GetDetector.vi"() -> ("ypixels"=w2083:i32)  [unwired: 4 in, 3 out]
                    n1093 = In Range and Coerce(upper limit=w2083, x=w2081, lower limit=1) -> (coerced(x)=w2080:i32)  [unwired: 1 out]
                    n1094 = local write "Initial Line 4"(w2080) -> ()
                  }
                  frame "INITIALCOLUMN" {
                    n1095 = Decimal String To Number(string=w2086) -> (number=w2089:i32)  [unwired: 2 in, 1 out]
                    n1096 = call <userlib>:"GetDetector.vi"() -> ("xpixels"=w2087:i32)  [unwired: 4 in, 3 out]
                    n1097 = In Range and Coerce(upper limit=w2087, x=w2089, lower limit=1) -> (coerced(x)=w2085:i32)  [unwired: 1 out]
                    n1098 = local write "Initial Cloumn 4"(w2085) -> ()
                  }
                  frame "FINALLINE" {
                    n1099 = Decimal String To Number(string=w2092) -> (number=w2094:i32)  [unwired: 2 in, 1 out]
                    n1100 = call <userlib>:"GetDetector.vi"() -> ("ypixels"=w2091:i32)  [unwired: 4 in, 3 out]
                    n1101 = In Range and Coerce(upper limit=w2091, x=w2094, lower limit=1) -> (coerced(x)=w2090:i32)  [unwired: 1 out]
                    n1102 = local write "Final Line 4"(w2090) -> ()
                  }
                  frame "FINALCOLUMN" {
                    n1103 = Decimal String To Number(string=w2096) -> (number=w2099:i32)  [unwired: 2 in, 1 out]
                    n1104 = call <userlib>:"GetDetector.vi"() -> ("xpixels"=w2098:i32)  [unwired: 4 in, 3 out]
                    n1105 = In Range and Coerce(upper limit=w2098, x=w2099, lower limit=1) -> (coerced(x)=w2095:i32)  [unwired: 1 out]
                    n1106 = local write "Final Column 4"(w2095) -> ()
                  }
                  frame "HORIZONTALBINNING" {
                    n1107 = Decimal String To Number(string=w2106) -> (number=w2100:i32)  [unwired: 2 in, 1 out]
                    n1108 = call <userlib>:"GetDetector.vi"() -> ("xpixels"=w2105:i32)  [unwired: 4 in, 3 out]
                    n1109 = Quotient & Remainder(x=w2105, y=w2100) -> (x-y*floor(x/y)=w2104:i32)  [unwired: 1 out]
                    n1110 = Equal?(x=0 ("index"), y=w2104) -> (x = y?=w2101:bool)
                    n1111 = case shown="False" w2101 {
                      tunnel: "INVALID VALUE FOR HORIZONTAL BINNING" -> [w2108 _]
                      tunnel: w2100 -> [w2107 w2112]
                      frame False {
                        n1112 = Number To Decimal String(number=w2107) -> (decimal integer string=w2111:string)  [unwired: 1 in]
                        n1113 = Concatenate Strings(w2108, w2111) -> (w2110:string)
                        n1114 = One Button Dialog(message=w2110, button name ("OK")="OK") -> ()  [unwired: 1 out]
                      }
                      frame True {
                        n1115 = local write "Binning 8"(w2112) -> ()
                      }
                    }
                  }
                  frame "SUBIMAGE" {
                  }
                  frame "EMMODE" {
                    n1116 = case shown="\"ELECTRON MULTIPLYING\", Default" w2114 {
                      tunnel: [w2115 w2116] -> w2113
                      frame "ELECTRON MULTIPLYING", Default {
                        w2115 = u8 0 items=["Electron Multiplying", "Conventional"] ("EM Mode")
                      }
                      frame "CONVENTIONAL" {
                        w2116 = u8 1 items=["Electron Multiplying", "Conventional"] ("EM Mode")
                      }
                    }
                    n1117 = local write "EM Mode 4"(w2113) -> ()
                  }
                  frame "EMGAIN" {
                    n1118 = Decimal String To Number(string=w2121) -> (number=w2118:i32)  [unwired: 2 in, 1 out]
                    n1119 = In Range and Coerce(upper limit=300 ("index"), x=w2118, lower limit=2 ("index")) -> (coerced(x)=w2117:i32)  [unwired: 1 out]
                    n1120 = local write "EM Gain 4"(w2117) -> ()
                  }
                }
              }
            }
          }
        }
      }
      event "Save CH1": Value Change {
        w2124 = 50 ("number")
        n1121 = event-data() -> ()  [unwired: 1 in, 1 out]
        n1122 = local read "EM Mode"() -> (w2170:u8)
        n1123 = local read "Cooler ON/OFF"() -> (w2168:u16)
        n1124 = local read "Readout Rate"() -> (w2169:u8)
        n1125 = local read "Pre-amp gain"() -> (w2167:u8)
        n1126 = case shown="1" w2170 {
          tunnel: ["CONVENTIONAL" "ELECTRON MULTIPLYING"] -> w2157
          frame 0, Default {
          }
          frame 1 {
          }
        }
        n1127 = case shown="3" w2169 {
          tunnel: ["1 MHz" "10 MHz" "20 MHz" "30 MHz"] -> w2163
          frame 0, Default {
          }
          frame 1 {
          }
          frame 2 {
          }
          frame 3 {
          }
        }
        n1128 = case shown="1" w2167 {
          tunnel: ["GAIN 1" "GAIN 2"] -> w2162
          frame 0, Default {
          }
          frame 1 {
          }
        }
        n1129 = case shown="1" w2168 {
          tunnel: ["COOLER OFF" "COOLER ON"] -> w2159
          frame 0, Default {
          }
          frame 1 {
          }
        }
        n1130 = local read "Exposure Time 2"() -> (w2148:dbl)
        n1131 = local read "Set temperature"() -> (w2150:i8)
        n1132 = local read "Initial Cloumn"() -> (w2152:u16)
        n1133 = local read "Binning 5"() -> (w2155:u8)
        n1134 = Bundle By Name(cluster="Setup", "CHANNEL"="1", "Read Mode"="IMAGE", "Trigger"="EXTERNAL START", "VShift Speed"="4,33", "Readout rate"=w2163, "Pre amp"=w2162, "Shutter Mode"="CLOSED", "Shutter TTL"="TTL LOW", "Cooler"=w2159, "Acquisition Mode"="KINETIC", "Initial Line"=w2157) -> (w2137:T2)
        n1135 = local read "Final Column"() -> (w2154:u16)
        n1136 = local read "Initial Line"() -> (w2151:u16)
        n1137 = local read "Final Line"() -> (w2153:u16)
        n1138 = local read "EM Gain"() -> (w2149:u16)
        n1139 = Number To Fractional String(number=sgl 4.33) -> (F-format string=w2122:string)  [unwired: 3 in]
        n1140 = Number To Decimal String(number=w2148) -> (decimal integer string=w2147:string)  [unwired: 1 in]
        n1141 = Number To Decimal String(number=w2124) -> (decimal integer string=w2146:string)  [unwired: 1 in]
        n1142 = Number To Decimal String(number=w2124) -> (decimal integer string=w2145:string)  [unwired: 1 in]
        n1143 = Number To Decimal String(number=w2150) -> (decimal integer string=w2144:string)  [unwired: 1 in]
        n1144 = Number To Decimal String(number=w2151) -> (decimal integer string=w2143:string)  [unwired: 1 in]
        n1145 = Number To Decimal String(number=w2152) -> (decimal integer string=w2142:string)  [unwired: 1 in]
        n1146 = Number To Decimal String(number=w2153) -> (decimal integer string=w2141:string)  [unwired: 1 in]
        n1147 = Number To Decimal String(number=w2154) -> (decimal integer string=w2140:string)  [unwired: 1 in]
        n1148 = Number To Decimal String(number=w2155) -> (decimal integer string=w2139:string)  [unwired: 1 in]
        n1149 = Number To Decimal String(number=w2149) -> (decimal integer string=w2138:string)  [unwired: 1 in]
        n1150 = Bundle By Name(cluster=w2137, "Exposure Time"=w2147, "Time to open shutter"=w2146, "Time to close shutter"=w2145, "Temperature"=w2144, "Initial Line"=w2143, "Initial Column"=w2142, "Final Line"=w2141, "Final Column"=w2140, "Horizontal binning"=w2139, "Vertical binning"=w2122, "EM Gain"=w2138) -> (w2136:T2)
        n1151 = call-dynamic "Read Setup File.lvclass.vi"("error in (no error)"=w2132, "SPARC4_AC in"=w2133) -> ("error out"=w2131:errorcluster, "Setup File.lvclass"=w2130:refnum<class "Setup File.lvclass">, "SPARC4_AC out"=w2129:refnum<class "SPARC4_AC.lvclass">)  [unwired: 7 in]
        n1152 = call "Write File Setup.vi"("error in (no error)"=w2131, "Setup"=w2136, "Setup File in"=w2130) -> ("error out"=w2128:errorcluster, "Setup File out"=w2125:refnum<class "Setup File.lvclass">)  [unwired: 7 in]
        n1153 = call "Write Customized File.vi"("error in (no error)"=w2128, "Setup File in"=w2125) -> ("error out"=w2127:errorcluster, "Setup File out"=w2126:refnum<class "Setup File.lvclass">)  [unwired: 8 in]
        n1154 = call-dynamic "Write Setup File.lvclass.vi"("error in (no error)"=w2127, "Setup File.lvclass"=w2126, "SPARC4_AC in"=w2129) -> ("error out"=w2135:errorcluster, "SPARC4_AC out"=w2134:refnum<class "SPARC4_AC.lvclass">)  [unwired: 7 in]
      }
      event "Save CH2": Value Change {
        w2183 = 50 ("number")
        n1155 = event-data() -> ()  [unwired: 1 in, 1 out]
        n1156 = local read "Cooler ON/OFF 2"() -> (w2193:u16)
        n1157 = local read "EM Mode 2"() -> (w2192:u8)
        n1158 = local read "Readout Rate 2"() -> (w2195:u8)
        n1159 = local read "Pre-amp gain 2"() -> (w2194:u8)
        n1160 = case shown="1" w2192 {
          tunnel: ["CONVENTIONAL" "ELECTRON MULTIPLYING"] -> w2210
          frame 0, Default {
          }
          frame 1 {
          }
        }
        n1161 = case shown="3" w2195 {
          tunnel: ["1 MHz" "10 MHz" "20 MHz" "30 MHz"] -> w2216
          frame 0, Default {
          }
          frame 1 {
          }
          frame 2 {
          }
          frame 3 {
          }
        }
        n1162 = case shown="1" w2194 {
          tunnel: ["GAIN 1" "GAIN 2"] -> w2215
          frame 0, Default {
          }
          frame 1 {
          }
        }
        n1163 = case shown="1" w2193 {
          tunnel: ["COOLER OFF" "COOLER ON"] -> w2212
          frame 0, Default {
          }
          frame 1 {
          }
        }
        n1164 = local read "Set temperature 2"() -> (w2190:i8)
        n1165 = local read "Initial Cloumn 2"() -> (w2187:u16)
        n1166 = local read "Exposure Time 4"() -> (w2189:u32)
        n1167 = local read "Final Column 2"() -> (w2185:u16)
        n1168 = local read "Binning 6"() -> (w2182:u16)
        n1169 = local read "Initial Line 2"() -> (w2188:u16)
        n1170 = local read "Final Line 2"() -> (w2186:u16)
        n1171 = local read "EM Gain 2"() -> (w2191:u16)
        n1172 = local read "Setup"() -> (w2196:T2)
        n1173 = Bundle By Name(cluster=w2196, "CHANNEL"="2", "Read Mode"="IMAGE", "Trigger"="EXTERNAL START", "VShift Speed"="4,33", "Readout rate"=w2216, "Pre amp"=w2215, "Shutter Mode"="CLOSED", "Shutter TTL"="TTL LOW", "Cooler"=w2212, "Acquisition Mode"="KINETIC", "Initial Line"=w2210) -> (w2198:T2)
        n1174 = Number To Decimal String(number=w2189) -> (decimal integer string=w2209:string)  [unwired: 1 in]
        n1175 = Number To Decimal String(number=w2183) -> (decimal integer string=w2208:string)  [unwired: 1 in]
        n1176 = Number To Decimal String(number=w2183) -> (decimal integer string=w2207:string)  [unwired: 1 in]
        n1177 = Number To Decimal String(number=w2190) -> (decimal integer string=w2206:string)  [unwired: 1 in]
        n1178 = Number To Decimal String(number=w2188) -> (decimal integer string=w2205:string)  [unwired: 1 in]
        n1179 = Number To Decimal String(number=w2187) -> (decimal integer string=w2204:string)  [unwired: 1 in]
        n1180 = Number To Decimal String(number=w2186) -> (decimal integer string=w2203:string)  [unwired: 1 in]
        n1181 = Number To Decimal String(number=w2185) -> (decimal integer string=w2202:string)  [unwired: 1 in]
        n1182 = Number To Decimal String(number=w2182) -> (decimal integer string=w2201:string)  [unwired: 1 in]
        n1183 = Number To Decimal String(number=w2182) -> (decimal integer string=w2200:string)  [unwired: 1 in]
        n1184 = Number To Decimal String(number=w2191) -> (decimal integer string=w2199:string)  [unwired: 1 in]
        n1185 = Bundle By Name(cluster=w2198, "Exposure Time"=w2209, "Time to open shutter"=w2208, "Time to close shutter"=w2207, "Temperature"=w2206, "Initial Line"=w2205, "Initial Column"=w2204, "Final Line"=w2203, "Final Column"=w2202, "Horizontal binning"=w2201, "Vertical binning"=w2200, "EM Gain"=w2199) -> (w2184:T2)
        n1186 = call-dynamic "Read Setup File.lvclass.vi"("error in (no error)"=w2220, "SPARC4_AC in"=w2221) -> ("error out"=w2230:errorcluster, "Setup File.lvclass"=w2229:refnum<class "Setup File.lvclass">, "SPARC4_AC out"=w2228:refnum<class "SPARC4_AC.lvclass">)  [unwired: 7 in]
        n1187 = call "Write File Setup.vi"("error in (no error)"=w2230, "Setup"=w2184, "Setup File in"=w2229) -> ("error out"=w2227:errorcluster, "Setup File out"=w2224:refnum<class "Setup File.lvclass">)  [unwired: 7 in]
        n1188 = call "Write Customized File.vi"("error in (no error)"=w2227, "Setup File in"=w2224) -> ("error out"=w2226:errorcluster, "Setup File out"=w2225:refnum<class "Setup File.lvclass">)  [unwired: 8 in]
        n1189 = call-dynamic "Write Setup File.lvclass.vi"("error in (no error)"=w2226, "Setup File.lvclass"=w2225, "SPARC4_AC in"=w2228) -> ("error out"=w2223:errorcluster, "SPARC4_AC out"=w2222:refnum<class "SPARC4_AC.lvclass">)  [unwired: 7 in]
      }
      event "Save CH3": Value Change {
        w2242 = 50 ("number")
        n1190 = event-data() -> ()  [unwired: 1 in, 1 out]
        n1191 = local read "EM Mode 3"() -> (w2254:u8)
        n1192 = local read "Cooler ON/OFF 3"() -> (w2253:u16)
        n1193 = local read "Pre-amp gain 3"() -> (w2252:u8)
        n1194 = local read "Readout Rate 3"() -> (w2251:u8)
        n1195 = case shown="1" w2254 {
          tunnel: ["CONVENTIONAL" "ELECTRON MULTIPLYING"] -> w2274
          frame 0, Default {
          }
          frame 1 {
          }
        }
        n1196 = case shown="3" w2251 {
          tunnel: ["1 MHz" "10 MHz" "20 MHz" "30 MHz"] -> w2280
          frame 0, Default {
          }
          frame 1 {
          }
          frame 2 {
          }
          frame 3 {
          }
        }
        n1197 = case shown="1" w2252 {
          tunnel: ["GAIN 1" "GAIN 2"] -> w2279
          frame 0, Default {
          }
          frame 1 {
          }
        }
        n1198 = case shown="1" w2253 {
          tunnel: ["COOLER OFF" "COOLER ON"] -> w2276
          frame 0, Default {
          }
          frame 1 {
          }
        }
        n1199 = local read "Initial Line 3"() -> (w2247:u16)
        n1200 = local read "Initial Cloumn 3"() -> (w2246:u16)
        n1201 = local read "Final Line 3"() -> (w2245:u16)
        n1202 = local read "Final Column 3"() -> (w2244:u16)
        n1203 = local read "Set temperature 3"() -> (w2250:i8)
        n1204 = local read "Exposure Time 7"() -> (w2249:dbl)
        n1205 = local read "Binning 7"() -> (w2243:u16)
        n1206 = local read "EM Gain 3"() -> (w2248:u16)
        n1207 = local read "Setup"() -> (w2261:T2)
        n1208 = Bundle By Name(cluster=w2261, "CHANNEL"="2", "Read Mode"="IMAGE", "Trigger"="EXTERNAL START", "VShift Speed"="4,33", "Readout rate"=w2280, "Pre amp"=w2279, "Shutter Mode"="CLOSED", "Shutter TTL"="TTL LOW", "Cooler"=w2276, "Acquisition Mode"="KINETIC", "Initial Line"=w2274) -> (w2262:T2)
        n1209 = Number To Decimal String(number=w2249) -> (decimal integer string=w2273:string)  [unwired: 1 in]
        n1210 = Number To Decimal String(number=w2242) -> (decimal integer string=w2272:string)  [unwired: 1 in]
        n1211 = Number To Decimal String(number=w2242) -> (decimal integer string=w2271:string)  [unwired: 1 in]
        n1212 = Number To Decimal String(number=w2250) -> (decimal integer string=w2270:string)  [unwired: 1 in]
        n1213 = Number To Decimal String(number=w2247) -> (decimal integer string=w2269:string)  [unwired: 1 in]
        n1214 = Number To Decimal String(number=w2246) -> (decimal integer string=w2268:string)  [unwired: 1 in]
        n1215 = Number To Decimal String(number=w2245) -> (decimal integer string=w2267:string)  [unwired: 1 in]
        n1216 = Number To Decimal String(number=w2244) -> (decimal integer string=w2266:string)  [unwired: 1 in]
        n1217 = Number To Decimal String(number=w2243) -> (decimal integer string=w2265:string)  [unwired: 1 in]
        n1218 = Number To Decimal String(number=4.33) -> (decimal integer string=w2264:string)  [unwired: 1 in]
        n1219 = Number To Decimal String(number=w2248) -> (decimal integer string=w2263:string)  [unwired: 1 in]
        n1220 = Bundle By Name(cluster=w2262, "Exposure Time"=w2273, "Time to open shutter"=w2272, "Time to close shutter"=w2271, "Temperature"=w2270, "Initial Line"=w2269, "Initial Column"=w2268, "Final Line"=w2267, "Final Column"=w2266, "Horizontal binning"=w2265, "Vertical binning"=w2264, "EM Gain"=w2263) -> (w2260:T2)
        n1221 = call-dynamic "Read Setup File.lvclass.vi"("error in (no error)"=w2255, "SPARC4_AC in"=w2256) -> ("error out"=w2290:errorcluster, "Setup File.lvclass"=w2289:refnum<class "Setup File.lvclass">, "SPARC4_AC out"=w2288:refnum<class "SPARC4_AC.lvclass">)  [unwired: 7 in]
        n1222 = call "Write File Setup.vi"("error in (no error)"=w2290, "Setup"=w2260, "Setup File in"=w2289) -> ("error out"=w2287:errorcluster, "Setup File out"=w2284:refnum<class "Setup File.lvclass">)  [unwired: 7 in]
        n1223 = call "Write Customized File.vi"("error in (no error)"=w2287, "Setup File in"=w2284) -> ("error out"=w2286:errorcluster, "Setup File out"=w2285:refnum<class "Setup File.lvclass">)  [unwired: 8 in]
        n1224 = call-dynamic "Write Setup File.lvclass.vi"("error in (no error)"=w2286, "Setup File.lvclass"=w2285, "SPARC4_AC in"=w2288) -> ("error out"=w2258:errorcluster, "SPARC4_AC out"=w2257:refnum<class "SPARC4_AC.lvclass">)  [unwired: 7 in]
      }
      event "Save CH4": Value Change {
        w2302 = 0
        n1225 = event-data() -> ()  [unwired: 1 in, 1 out]
        n1226 = local read "Cooler ON/OFF 4"() -> (w2314:u16)
        n1227 = local read "EM Mode 4"() -> (w2313:u8)
        n1228 = local read "Pre-amp gain 4"() -> (w2311:u8)
        n1229 = local read "Readout Rate 4"() -> (w2312:u8)
        n1230 = case shown="1" w2313 {
          tunnel: ["CONVENTIONAL" "ELECTRON MULTIPLYING"] -> w2334
          frame 0, Default {
          }
          frame 1 {
          }
        }
        n1231 = case shown="3" w2312 {
          tunnel: ["1 MHz" "10 MHz" "20 MHz" "30 MHz"] -> w2340
          frame 0, Default {
          }
          frame 1 {
          }
          frame 2 {
          }
          frame 3 {
          }
        }
        n1232 = case shown="1" w2311 {
          tunnel: ["GAIN 1" "GAIN 2"] -> w2339
          frame 0, Default {
          }
          frame 1 {
          }
        }
        n1233 = case shown="1" w2314 {
          tunnel: ["COOLER OFF" "COOLER ON"] -> w2336
          frame 0, Default {
          }
          frame 1 {
          }
        }
        n1234 = local read "Set temperature 4"() -> (w2309:i8)
        n1235 = local read "Exposure Time 8"() -> (w2310:dbl)
        n1236 = local read "Initial Cloumn 4"() -> (w2306:u16)
        n1237 = local read "Binning 8"() -> (w2303:u16)
        n1238 = local read "Final Column 4"() -> (w2304:u16)
        n1239 = local read "Initial Line 4"() -> (w2307:u16)
        n1240 = local read "Final Line 4"() -> (w2305:u16)
        n1241 = local read "EM Gain 4"() -> (w2308:u16)
        n1242 = local read "Setup"() -> (w2322:T2)
        n1243 = Bundle By Name(cluster=w2322, "CHANNEL"="2", "Read Mode"="IMAGE", "Trigger"="EXTERNAL START", "VShift Speed"="4,33", "Readout rate"=w2340, "Pre amp"=w2339, "Shutter Mode"="CLOSED", "Shutter TTL"="TTL LOW", "Cooler"=w2336, "Acquisition Mode"="KINETIC", "Initial Line"=w2334) -> (w2323:T2)
        n1244 = Number To Decimal String(number=w2310) -> (decimal integer string=w2333:string)  [unwired: 1 in]
        n1245 = Number To Decimal String(number=w2302) -> (decimal integer string=w2332:string)  [unwired: 1 in]
        n1246 = Number To Decimal String(number=w2302) -> (decimal integer string=w2331:string)  [unwired: 1 in]
        n1247 = Number To Decimal String(number=w2309) -> (decimal integer string=w2330:string)  [unwired: 1 in]
        n1248 = Number To Decimal String(number=w2307) -> (decimal integer string=w2329:string)  [unwired: 1 in]
        n1249 = Number To Decimal String(number=w2306) -> (decimal integer string=w2328:string)  [unwired: 1 in]
        n1250 = Number To Decimal String(number=w2305) -> (decimal integer string=w2327:string)  [unwired: 1 in]
        n1251 = Number To Decimal String(number=w2304) -> (decimal integer string=w2326:string)  [unwired: 1 in]
        n1252 = Number To Decimal String(number=w2303) -> (decimal integer string=w2325:string)  [unwired: 1 in]
        n1253 = Number To Fractional String(number=4.33) -> (F-format string=w2324:string)  [unwired: 3 in]
        n1254 = Number To Decimal String(number=w2308) -> (decimal integer string=w2315:string)  [unwired: 1 in]
        n1255 = Bundle By Name(cluster=w2323, "Exposure Time"=w2333, "Time to open shutter"=w2332, "Time to close shutter"=w2331, "Temperature"=w2330, "Initial Line"=w2329, "Initial Column"=w2328, "Final Line"=w2327, "Final Column"=w2326, "Horizontal binning"=w2325, "Vertical binning"=w2324, "EM Gain"=w2315) -> (w2321:T2)
        n1256 = call-dynamic "Read Setup File.lvclass.vi"("error in (no error)"=w2317, "SPARC4_AC in"=w2316) -> ("error out"=w2350:errorcluster, "Setup File.lvclass"=w2349:refnum<class "Setup File.lvclass">, "SPARC4_AC out"=w2348:refnum<class "SPARC4_AC.lvclass">)  [unwired: 7 in]
        n1257 = call "Write File Setup.vi"("error in (no error)"=w2350, "Setup"=w2321, "Setup File in"=w2349) -> ("error out"=w2347:errorcluster, "Setup File out"=w2344:refnum<class "Setup File.lvclass">)  [unwired: 7 in]
        n1258 = call "Write Customized File.vi"("error in (no error)"=w2347, "Setup File in"=w2344) -> ("error out"=w2346:errorcluster, "Setup File out"=w2345:refnum<class "Setup File.lvclass">)  [unwired: 8 in]
        n1259 = call-dynamic "Write Setup File.lvclass.vi"("error in (no error)"=w2346, "Setup File.lvclass"=w2345, "SPARC4_AC in"=w2348) -> ("error out"=w2319:errorcluster, "SPARC4_AC out"=w2318:refnum<class "SPARC4_AC.lvclass">)  [unwired: 7 in]
      }
      event "BIAS": Value Change {
        w2361 = 0
        n1260 = event-data() -> ()  [unwired: 1 in, 1 out]
        n1261 = local write "Exposure Time"(w2361) -> ()
        n1262 = local write "Exposure Time 3"(w2361) -> ()
        n1263 = local write "Exposure Time 6"(w2361) -> ()
        n1264 = local write "Exposure Time 5"(w2361) -> ()
        n1265 = local write "Exposure Time 2"(w2361) -> ()
        n1266 = local write "Exposure Time 4"(w2361) -> ()
        n1267 = local write "Exposure Time 7"(w2361) -> ()
        n1268 = local write "Exposure Time 8"(w2361) -> ()
      }
      event "Read mode": Value Change {
        n1269 = event-data() -> ()  [unwired: 1 in, 1 out]
        n1270 = case shown="\"1\", Default" "Read mode" {
          tunnel: [w2369 w2371 w2373] -> _
          tunnel: [w2368 w2370 w2372] -> w2364
          frame "1", Default {
            w2368 = u8 3 items=["1 MHz", "10 MHz", "20 MHz", "30 MHz"] ("Readout Rate 4")
            w2369 = u8 0 items=["0.6", "1.13", "2.2", "4.33"] ("Vertical Shift \nSpeed 4")
          }
          frame "2" {
            w2370 = u8 2 items=["1 MHz", "10 MHz", "20 MHz", "30 MHz"] ("Readout Rate 4")
            w2371 = u8 1 items=["0.6", "1.13", "2.2", "4.33"] ("Vertical Shift \nSpeed 4")
          }
          frame "3" {
            w2372 = u8 0 items=["1 MHz", "10 MHz", "20 MHz", "30 MHz"] ("Readout Rate 4")
            w2373 = u8 3 items=["0.6", "1.13", "2.2", "4.33"] ("Vertical Shift \nSpeed 4")
          }
        }
        n1271 = local write "Readout Rate"(w2364) -> ()
        n1272 = local write "Readout Rate 2"(w2364) -> ()
        n1273 = local write "Readout Rate 3"(w2364) -> ()
        n1274 = local write "Readout Rate 4"(w2364) -> ()
      }
      event "Night Directory": Value Change {
        n1275 = event-data() -> ()  [unwired: 1 in, 1 out]
        n1276 = local read "Night Directory"() -> (w2377:string)
        n1277 = String Length(string=w2377) -> (length=w2382:i32)
        n1278 = Decrement(x=w2382) -> (x-1=w2381:i32)
        n1279 = String Subset(string=w2377, offset (0)=w2381) -> (substring=w2380:string)  [unwired: 1 in]
        n1280 = Equal?(x=w2380, y="\\") -> (x = y?=w2379:bool)
        n1281 = case shown="True" w2379 {
          tunnel: [w2385 w2386] -> w2376
          tunnel: w2377 -> [w2383 w2386]
          frame False {
            n1282 = Concatenate Strings(w2383, "\\") -> (w2385:string)
          }
          frame True {
          }
        }
        n1283 = local write "Night Directory"(w2376) -> ()
      }
      event "EM Mode": Value Change {
        w2388 = u8 0 items=["30 MHz", "20 MHz", "10 MHz", "1 MHz"] ("Readout Rate")
        n1284 = event-data() -> ()  [unwired: 1 in, 2 out]
        n1285 = local read "EM Mode"() -> (w2389:u8)
        n1286 = local write "Readout Rate"(w2388) -> ()
        n1287 = case shown="0, Default" w2389 {
          tunnel: [string[] ["30 MHz", "20 MHz", "10 MHz", "  1 MHz"] string[] ["   1 MHz", "0.1 MHz"]] -> w2387
          frame 0, Default {
          }
          frame 1 {
          }
        }
        n1288 = property on="Readout Rate" class="Ring (strict)"("Strings []"=w2387) -> ()  [unwired: 2 in, 2 out]
      }
    }
    n1289 = Wait Until Next ms Multiple(millisecond multiple=u32 5) -> ()  [unwired: 1 out]
  }
  n1290 = call-dynamic "Read Sync Box.lvclass.vi"("SPARC4_AC in"=w77) -> ("error out"=w75:errorcluster, "Sync Box.lvclass"=w76:refnum<class "Sync Box.lvclass">, "SPARC4_AC out"=w72:refnum<class "SPARC4_AC.lvclass">)  [unwired: 8 in]
  n1291 = call "Close Connection.vi"("error in (no error)"=w75, "Sync Box in"=w76) -> ("error out"=w74:errorcluster, "Sync Box out"=w73:refnum<class "Sync Box.lvclass">)  [unwired: 8 in]
  n1292 = call-dynamic "Write Sync Box.lvclass.vi"("error in (no error)"=w74, "Sync Box.lvclass"=w73, "SPARC4_AC in"=w72) -> ("error out"=w71:errorcluster, "SPARC4_AC out"=w70:refnum<class "SPARC4_AC.lvclass">)  [unwired: 7 in]
  n1293 = call-dynamic "Read Channel Manager.lvclass.vi"("error in (no error)"=w71, "SPARC4_AC in"=w70) -> ("error out"=w29:errorcluster, "Channel Manager.lvclass"=w30:refnum<class "Channel Manager.lvclass">)  [unwired: 7 in, 1 out]
  n1294 = call-dynamic "Read Available Cameras.vi"("error in (no error)"=w29, "Channel Manager in"=w30) -> ("error out"=w28:errorcluster, "Available Cameras"=w26:u8, "Channel Manager out"=w27:refnum<class "Channel Manager.lvclass">)  [unwired: 7 in]
  n1295 = for {
    N: w26 -> [_]
    tunnel: w27 -> [w2396]
    tunnel: w28 -> [w2395]
    tunnel: [w2400] -> w54
    tunnel: [w2399] -> w55
    i -> [w2394]
    n1296 = call-dynamic "Write Current Camera.vi"("error in (no error)"=w2395, "Current Camera"=w2394, "Channel Manager in"=w2396) -> ("error out"=w2398:errorcluster, "Channel Manager out"=w2397:refnum<class "Channel Manager.lvclass">)  [unwired: 7 in]
    n1297 = call "Return Current RxTx.vi"("error in (no error)"=w2398, "Channel Manager in"=w2397) -> ("error out"=w2404:errorcluster, "RxTx"=w2405:refnum<class "RxTx.lvclass">, "Channel Manager out"=w2401:refnum<class "Channel Manager.lvclass">)  [unwired: 7 in]
    n1298 = Number To Decimal String(number=w2394) -> (decimal integer string=w2407:string)  [unwired: 1 in]
    n1299 = Concatenate Strings("STOP CH", w2407) -> (w2406:string)
    n1300 = call-dynamic "Read Interface.lvclass.vi"("error in (no error)"=w2404, "RxTx in"=w2405) -> ("error out"=w2414:errorcluster, "Interface.lvclass"=w2415:refnum<class "Interface.lvclass">, "RxTx out"=w2409:refnum<class "RxTx.lvclass">)  [unwired: 7 in]
    n1301 = call "Write Command.vi"("error in (no error)"=w2414, "Command"=w2406, "Interface in"=w2415) -> ("error out"=w2411:errorcluster, "Interface out"=w2410:refnum<class "Interface.lvclass">)  [unwired: 7 in]
    n1302 = call-dynamic "Write Interface.lvclass.vi"("error in (no error)"=w2411, "Interface.lvclass"=w2410, "RxTx in"=w2409) -> ("error out"=w2413:errorcluster, "RxTx out"=w2412:refnum<class "RxTx.lvclass">)  [unwired: 7 in]
    n1303 = call "Enqeue A Message.vi"("error in (no error)"=w2413, "RxTx in"=w2412) -> ("error out"=w2403:errorcluster, "RxTx out"=w2402:refnum<class "RxTx.lvclass">)  [unwired: 8 in]
    n1304 = call "Write Current RxTx.vi"("error in (no error)"=w2403, "RxTx"=w2402, "Channel Manager in"=w2401) -> ("error out"=w2400:errorcluster, "Channel Manager out"=w2399:refnum<class "Channel Manager.lvclass">)  [unwired: 7 in]
  }
  n1305 = flat-sequence {
    tunnel: w55 -> [_]
    tunnel: w54 -> [_]
    frame #0 {
      w2417 = u16 0 items=["Cooler OFF", "Cooler ON"] ("Cooler ON/OFF")
      w2427 = u8 0 items=["Electron Multiplying", "Conventional"] ("EM Mode")
      (unwired) u8 0 items=["0.6", "1.13", "2.2", "4.33"] ("Vertical Shift \nSpeed")
      w2429 = u8 0 items=["1 MHz", "10 MHz", "20 MHz", "30 MHz"] ("Readout Rate")
      w2430 = u8 0 items=["Gain 1", "Gain 2"] ("Pre-amp gain")
      w2434 = u16 1024 ("Final Line")
      w2435 = u16 1 ("Initial Line")
      w2436 = u32 14079702
      n1306 = Bundle(u32 1985280, u32 1985280) -> (w2442:cluster{u32, u32})  [unwired: 1 in]
      n1307 = control-ref of="Initialization"() -> (w2438:refnum<vi>)
      n1308 = Build Array(w2442) -> (w2439:cluster{u32, u32}[])
      n1309 = local write "Initial Line"(w2435) -> ()
      n1310 = local write "Initial Cloumn"(w2435) -> ()
      n1311 = local write "Final Line"(w2434) -> ()
      n1312 = local write "Final Column"(w2434) -> ()
      n1313 = property on="Property Node" class="Bool (strict)"(reference=w2438, "Colors [4]"=w2439) -> ()  [unwired: 1 in, 2 out]
      n1314 = local write "Binning 5"(u16 1 ("Vertical Binning")) -> ()
      n1315 = property on="Readout Rate" class="Ring (strict)"("Strings []"=string[] ["30 MHz", "20 MHz", "10 MHz", "  1 MHz"]) -> ()  [unwired: 2 in, 2 out]
      n1316 = local write "Sub Image"(T8."1024 x 1024" ("Sub Image")) -> ()
      n1317 = local write "Kinetic Series Length"(u32 1 ("Kinetic Series Length")) -> ()
      n1318 = local write "Cooler ON/OFF"(w2417) -> ()
      n1319 = local write "Set temperature"(i8 20 ("Set temperature")) -> ()
      n1320 = local write "Stop Button"(FALSE ("Stop Button")) -> ()
      n1321 = local write "Temperature ºC"(20.0 ("Temperature ºC")) -> ()
      n1322 = local write "Initialization"(FALSE ("Initialization")) -> ()
      n1323 = property on="Temperature" class="DigNum (strict)"("NumText.BGColor"=w2436) -> ()  [unwired: 2 in, 2 out]
      n1324 = property on="Temperature" class="DigNum (strict)"("NumText.BG Color"=w2436) -> ()  [unwired: 2 in, 2 out]
      n1325 = local write "Exposure Time 2"(1e-05 ("Exposure Time 2")) -> ()
      n1326 = local write "EM Mode"(w2427) -> ()
      n1327 = local write "EM Gain"(u16 2 ("EM Gain")) -> ()
      n1328 = local write "Readout Rate"(w2429) -> ()
      n1329 = local write "Pre-amp gain"(w2430) -> ()
      n1330 = local write "Exposure Time"(1e-05 ("Exposure Time")) -> ()
      n1331 = local write "Exposições realizadas"(u8 0 ("Exposições realizadas")) -> ()
      n1332 = property on="Exposições realizadas" class="Slide (strict)"("Scale.Maximum"=1.0 ("Scale.Range:Maximum")) -> ()  [unwired: 2 in, 2 out]
      n1333 = local write "Exposing"(FALSE ("Stop Button")) -> ()
      n1334 = local write "# Ciclos"(u32 1 ("# Images")) -> ()
      n1335 = local write "Set temperature"(i8 20 ("Set temperature")) -> ()
      n1336 = local write "Temperature"(i16 20 ("Temperature")) -> ()
      n1337 = local write "# Ciclos"(u32 1 ("# Images")) -> ()
    }
    frame #1 {
      w2447 = FALSE ("Initialization 2")
      w2449 = u32 14079702
      w2460 = u8 0 items=["Electron Multiplying", "Conventional"] ("EM Mode")
      w2462 = u8 0 items=["Gain 1", "Gain 2"] ("Pre-amp gain")
      w2464 = u8 0 items=["1 MHz", "10 MHz", "20 MHz", "30 MHz"] ("Readout Rate")
      w2467 = u16 0 items=["Cooler OFF", "Cooler ON"] ("Cooler ON/OFF")
      w2468 = 20.0 ("Temperature ºC")
      n1338 = Bundle(u32 1985280, u32 1985280) -> (w2452:cluster{u32, u32})  [unwired: 1 in]
      n1339 = control-ref of="Initialization 2"() -> (w2451:refnum<vi>)
      n1340 = local write "EM Gain 2"(u16 2 ("EM Gain")) -> ()
      n1341 = local write "Exposure Time 4"(0.0 ("Exposure Time 2")) -> ()
      n1342 = local write "Final Line 2"(u16 1 ("Initial Line")) -> ()
      n1343 = local write "Readout Rate 2"(w2464) -> ()
      n1344 = local write "Final Column 2"(u16 1024 ("Final Line")) -> ()
      n1345 = local write "Pre-amp gain 2"(w2462) -> ()
      n1346 = local write "Set temperature 2"(w2468) -> ()
      n1347 = local write "Temperature ºC 2"(w2468) -> ()
      n1348 = local write "Cooler ON/OFF 2"(w2467) -> ()
      n1349 = local write "Exposure Time 3"(0.0 ("Exposure Time 2")) -> ()
      n1350 = Build Array(w2452) -> (w2455:cluster{u32, u32}[])
      n1351 = local write "Binning 6"(u16 1 ("Initial Line")) -> ()
      n1352 = local write "Initial Cloumn 2"(u32 1 ("# Images")) -> ()
      n1353 = local write "Initial Line 2"(u16 1 ("Initial Line")) -> ()
      n1354 = local write "# Images 2"(u32 1 ("# Images")) -> ()
      n1355 = local write "EM Mode 2"(w2460) -> ()
      n1356 = property on="Property Node" class="Bool (strict)"(reference=w2451, "Colors [4]"=w2455) -> ()  [unwired: 1 in, 2 out]
      n1357 = local write "Exposing 2"(FALSE ("Stop Button")) -> ()
      n1358 = local write "Exposições realizadas 2"(u8 0 ("Exposições realizadas 2")) -> ()
      n1359 = property on="Exposições realizadas 2" class="Slide (strict)"("Scale.Maximum"=1.0 ("Scale.Range:Maximum")) -> ()  [unwired: 2 in, 2 out]
      n1360 = local write "Initialization 2"(w2447) -> ()
      n1361 = local write "Sync Mode"(w2447) -> ()
      n1362 = property on="Temperature 2" class="DigNum (strict)"("NumText.BGColor"=w2449) -> ()  [unwired: 2 in, 2 out]
      n1363 = property on="Temperature 2" class="DigNum (strict)"("NumText.BG Color"=w2449) -> ()  [unwired: 2 in, 2 out]
    }
    frame #2 {
      w2473 = u32 14079702
      w2480 = u16 0 items=["Cooler OFF", "Cooler ON"] ("Cooler ON/OFF")
      w2486 = u16 1 ("Initial Cloumn 3")
      w2487 = u8 0 items=["1 MHz", "10 MHz", "20 MHz", "30 MHz"] ("Readout Rate 3")
      w2488 = u8 0 items=["Electron Multiplying", "Conventional"] ("EM Mode 3")
      w2489 = u8 0 items=["Gain 1", "Gain 2"] ("Pre-amp gain 3")
      n1364 = Bundle(u32 1985280, u32 1985280) -> (w2478:cluster{u32, u32})  [unwired: 1 in]
      n1365 = control-ref of="Initialization 3"() -> (w2479:refnum<vi>)
      n1366 = Build Array(w2478) -> (w2475:cluster{u32, u32}[])
      n1367 = local write "Pre-amp gain 3"(w2489) -> ()
      n1368 = local write "Readout Rate 3"(w2487) -> ()
      n1369 = local write "Initial Cloumn 3"(w2486) -> ()
      n1370 = local write "Initial Line 3"(w2486) -> ()
      n1371 = local write "Final Line 3"(u16 1024 ("Final Line 3")) -> ()
      n1372 = local write "EM Gain 3"(u16 2 ("EM Gain 3")) -> ()
      n1373 = local write "Final Column 3"(u16 1024 ("Final Column 3")) -> ()
      n1374 = local write "Exposure Time 7"(0.0 ("Exposure Time 7")) -> ()
      n1375 = property on="Temperature 3" class="DigNum (strict)"("NumText.BGColor"=w2473) -> ()  [unwired: 2 in, 2 out]
      n1376 = property on="Temperature 3" class="DigNum (strict)"("NumText.BG Color"=w2473) -> ()  [unwired: 2 in, 2 out]
      n1377 = local write "Cooler ON/OFF 3"(w2480) -> ()
      n1378 = property on="Exposições realizadas 3" class="Slide (strict)"("Scale.Maximum"=1.0 ("Scale.Range:Maximum")) -> ()  [unwired: 2 in, 2 out]
      n1379 = local write "# Images 3"(u32 1 ("# Images 3")) -> ()
      n1380 = property on="Property Node" class="Bool (strict)"(reference=w2479, "Colors [4]"=w2475) -> ()  [unwired: 1 in, 2 out]
      n1381 = local write "EM Mode 3"(w2488) -> ()
      n1382 = local write "Binning 7"(u16 1 ("Horizontal Binning 3")) -> ()
      n1383 = local write "Exposições realizadas 3"(u8 0 ("Exposições realizadas 2")) -> ()
      n1384 = local write "Initialization 3"(FALSE ("Initialization 2")) -> ()
      n1385 = local write "Exposing 3"(FALSE ("Stop Button")) -> ()
    }
    frame #3 {
      w2494 = u32 14079702
      w2501 = u8 0 items=["1 MHz", "10 MHz", "20 MHz", "30 MHz"] ("Readout Rate 4")
      w2502 = u8 0 items=["Gain 1", "Gain 2"] ("Pre-amp gain 4")
      w2510 = u8 0 items=["Electron Multiplying", "Conventional"] ("EM Mode 4")
      n1386 = Bundle(u32 1985280, u32 1985280) -> (w2497:cluster{u32, u32})  [unwired: 1 in]
      n1387 = local write "Initial Line 4"(u16 1 ("Initial Line 4")) -> ()
      n1388 = local write "# Images 4"(u32 1 ("# Images 4")) -> ()
      n1389 = local write "EM Gain 4"(u16 2 ("EM Gain 4")) -> ()
      n1390 = local write "Initial Cloumn 4"(u16 1 ("Initial Cloumn 4")) -> ()
      n1391 = control-ref of="Initialization 4"() -> (w2496:refnum<vi>)
      n1392 = local write "Exposure Time 8"(0.0 ("Exposure Time 8")) -> ()
      n1393 = local write "Final Line 4"(u16 1024 ("Final Line 4")) -> ()
      n1394 = local write "Final Column 4"(u16 1024 ("Final Column 4")) -> ()
      n1395 = local write "Exposições realizadas 4"(u8 0 ("Exposições realizadas 2")) -> ()
      n1396 = property on="Exposições realizadas 4" class="Slide (strict)"("Scale.Maximum"=1.0 ("Scale.Range:Maximum")) -> ()  [unwired: 2 in, 2 out]
      n1397 = local write "Pre-amp gain 4"(w2502) -> ()
      n1398 = local write "Readout Rate 4"(w2501) -> ()
      n1399 = property on="Temperature 4" class="DigNum (strict)"("NumText.BGColor"=w2494) -> ()  [unwired: 2 in, 2 out]
      n1400 = property on="Temperature 4" class="DigNum (strict)"("NumText.BG Color"=w2494) -> ()  [unwired: 2 in, 2 out]
      n1401 = local write "Binning 8"(u16 1 ("Horizontal Binning 4")) -> ()
      n1402 = Build Array(w2497) -> (w2500:cluster{u32, u32}[])
      n1403 = local write "Initialization 4"(FALSE ("Initialization 2")) -> ()
      n1404 = local write "Exposing 4"(FALSE ("Stop Button")) -> ()
      n1405 = property on="Property Node" class="Bool (strict)"(reference=w2496, "Colors [4]"=w2500) -> ()  [unwired: 1 in, 2 out]
      n1406 = local write "EM Mode 4"(w2510) -> ()
    }
    frame #4 {
      w2512 = T7."Enabled" ("Disabled")
      w2514 = T7."Disabled and Grayed Out" ("Disabled")
      n1407 = property on="Adquirir" class="Bool"("DisabledEnum"=w2512) -> ()  [unwired: 2 in, 2 out]
      n1408 = property on="Stop Acq" class="Bool"("DisabledEnum"=w2512) -> ()  [unwired: 2 in, 2 out]
      n1409 = property on="Pausar" class="Bool (strict)"("DisabledEnum"=w2512) -> ()  [unwired: 2 in, 2 out]
      n1410 = property on="Abort" class="Bool"("DisabledEnum"=w2512) -> ()  [unwired: 2 in, 2 out]
      n1411 = local write "Sync Mode"(FALSE ("Sync Mode")) -> ()
      n1412 = local write "Sync Mode: 2"(T3."Radio Selection 1" ("Sync Mode: 2")) -> ()
      n1413 = property on="Adquirir 2" class="Bool"("DisabledEnum"=w2512) -> ()  [unwired: 2 in, 2 out]
      n1414 = property on="Stop Acq 2" class="Bool"("DisabledEnum"=w2512) -> ()  [unwired: 2 in, 2 out]
      n1415 = property on="Pausar 2" class="Bool (strict)"("DisabledEnum"=w2512) -> ()  [unwired: 2 in, 2 out]
      n1416 = property on="Abort 2" class="Bool"("DisabledEnum"=w2512) -> ()  [unwired: 2 in, 2 out]
      n1417 = property on="Sync Mode: 2" class="RadioBtnsControl (strict)"("DisabledEnum"=w2514) -> ()  [unwired: 2 in, 2 out]
      n1418 = property on="Adquirir 3" class="Bool"("DisabledEnum"=T7."Disabled and Grayed Out" ("Disabled")) -> ()  [unwired: 2 in, 2 out]
      n1419 = property on="Stop Acq 3" class="Bool"("DisabledEnum"=T7."Disabled and Grayed Out" ("Disabled")) -> ()  [unwired: 2 in, 2 out]
      n1420 = property on="Pausar 3" class="Bool (strict)"("DisabledEnum"=w2514) -> ()  [unwired: 2 in, 2 out]
      n1421 = property on="Abort 3" class="Bool"("DisabledEnum"=T7."Disabled and Grayed Out" ("Disabled")) -> ()  [unwired: 2 in, 2 out]
      n1422 = property on="Adquirir 4" class="Bool"("DisabledEnum"=w2512) -> ()  [unwired: 2 in, 2 out]
      n1423 = property on="Stop Acq 4" class="Bool"("DisabledEnum"=w2512) -> ()  [unwired: 2 in, 2 out]
      n1424 = property on="Pausar 4" class="Bool (strict)"("DisabledEnum"=w2512) -> ()  [unwired: 2 in, 2 out]
      n1425 = property on="Abort 4" class="Bool"("DisabledEnum"=w2512) -> ()  [unwired: 2 in, 2 out]
      n1426 = property on="Adquirir 5" class="Bool"("DisabledEnum"=w2512) -> ()  [unwired: 2 in, 2 out]
      n1427 = property on="Stop Acq 5" class="Bool"("DisabledEnum"=w2512) -> ()  [unwired: 2 in, 2 out]
      n1428 = property on="Pausar 5" class="Bool (strict)"("DisabledEnum"=w2512) -> ()  [unwired: 2 in, 2 out]
      n1429 = property on="Abort 5" class="Bool"("DisabledEnum"=w2512) -> ()  [unwired: 2 in, 2 out]
    }
  }
